vi "Main_GraphBasedSLAM.vi"() -> ()   [LabVIEW 2019]
uses:
  Ctrl/cmd_ini-RW.ctl
  Ctrl/cmd_common.ctl
  <vilib>/Analysis/Matrix/Datatypes/RealMatrix.ctl
  <vilib>/Analysis/Matrix/Numeric/Conversions/Matrix To Array - RM.vi
  <vilib>/Analysis/Matrix/NI_Matrix.lvlib
panel:
  in  "tab":enum32{"ini val", "Graph"}(tab)=enum."Graph"
  in  "rf_id":cluster{"x":dbl, "y":dbl, "yaw":dbl}[](array[cluster])=[{"x"=10.0, "y"=-2.0, "yaw"=0.0}, {"x"=15.0, "y"=10.0, "yaw"=0.0}, {"x"=3.0, "y"=15.0, "yaw"=0.0}, {"x"=-5.0, "y"=20.0, "yaw"=0.0}, {"x"=-5.0, "y"=5.0, "yaw"=0.0}]
  out "x_opt out":cluster{"x":dbl, "y":dbl, "yaw":dbl}[](array[cluster])
  out "cost":cluster{"cost":dbl, "cost sum":dbl}(graph)
  out "inv(H) matrix":dbl[][](graph)
  out "H matrix":dbl[][](graph)
  in  "Show graph time":dbl=5.0
  out "GNSS Lat-Long":T1(graph)=[{[{"Real Matrix Element"=-0.03468968743701403, "Real Matrix Element"=0.0}, {"Real Matrix Element"=0.0053006342525533596, "Real Matrix Element"=0.0026827157844343482}, {"Real Matrix Element"=0.07941001084047958, "Real Matrix Element"=0.004354973789417695}, {"Real Matrix Element"=0.3362327951507724, "Real Matrix Element"=-0.0058186211497051445}, {"Real Matrix Element"=0.583991471643908, "Real Matrix Element"=-0.014127319370192896}, {"Real Matrix Element"=0.6015779562809649, "Real Matrix Element"=-0.01792914288198029}, {"Real Matrix Element"=0.781024837247035, "Real Matrix Element"=-0.03778541178555447}, {"Real Matrix Element"=0.7766402178508468, "Real Matrix Element"=-0.030292841174655537}, {"Real Matrix Element"=0.9431072219093555, "Real Matrix Element"=-0.011465267340174822}, {"Real Matrix Element"=0.9753969820468079, "Real Matrix Element"=-0.015941763963851434}, {"Real Matrix Element"=1.2132401576078795, "Real Matrix Element"=0.041893519310891164}, {"Real Matrix Element"=1.225107293796763, "Real Matrix Element"=0.047604652068552356}, {"Real Matrix Element"=1.2761491555327105, "Real Matrix Element"=0.0704489082853088}, {"Real Matrix Element"=1.4096463396242502, "Real Matrix Element"=0.0514810355329801}, {"Real Matrix Element"=1.6740586724996822, "Real Matrix Element"=0.009317748649650522}, {"Real Matrix Element"=1.8512682178384547, "Real Matrix Element"=-0.00638301099148434}, {"Real Matrix Element"=1.7681597665695883, "Real Matrix Element"=0.01034169292533106}, {"Real Matrix Element"=1.695081912768819, "Real Matrix Element"=0.0771652637847412}, {"Real Matrix Element"=1.8401006709321701, "Real Matrix Element"=0.03677338128353985}, {"Real Matrix Element"=2.1461565709863093, "Real Matrix Element"=0.01382817628790585}, {"Real Matrix Element"=2.1374096596401855, "Real Matrix Element"=0.057469030626545535}, {"Real Matrix Element"=2.1543438113032565, "Real Matrix Element"=0.1009952688750678}, {"Real Matrix Element"=2.146823758678734, "Real Matrix Element"=0.1367303180764168}, {"Real Matrix Element"=2.313726904376567, "Real Matrix Element"=0.15669480341095504}, {"Real Matrix Element"=2.448165076358712, "Real Matrix Element"=0.11806130227193384}, {"Real Matrix Element"=2.7581327970333787, "Real Matrix Element"=0.26114866202850523}, {"Real Matrix Element"=2.7786219786094453, "Real Matrix Element"=0.26959867008849003}, {"Real Matrix Element"=2.7594754945447324, "Real Matrix Element"=0.3049764548145187}, {"Real Matrix Element"=2.84464001198685, "Real Matrix Element"=0.3740548085974285}, {"Real Matrix Element"=3.0672617807939404, "Real Matrix Element"=0.4708806158706211}, {"Real Matrix Element"=3.0361758327160504, "Real Matrix Element"=0.44569336725203174}, {"Real Matrix Element"=3.2385063300702264, "Real Matrix Element"=0.6279704263246847}, {"Real Matrix Element"=3.158876246209658, "Real Matrix Element"=0.5887655997024159}, {"Real Matrix Element"=3.2657902319652283, "Real Matrix Element"=0.5698844075564534}, {"Real Matrix Element"=3.4763236561457407, "Real Matrix Element"=0.6411314057308733}, {"Real Matrix Element"=3.7070629090554124, "Real Matrix Element"=0.7376824418190701}, {"Real Matrix Element"=3.471507531519639, "Real Matrix Element"=0.6082208970914108}, {"Real Matrix Element"=3.468422407890875, "Real Matrix Element"=0.5832337660513986}, {"Real Matrix Element"=3.6926573968702523, "Real Matrix Element"=0.650637040965163}, {"Real Matrix Element"=3.786513246652574, "Real Matrix Element"=0.6968034902141617}, {"Real Matrix Element"=3.8331446853344846, "Real Matrix Element"=0.7214149291160856}, {"Real Matrix Element"=4.139757466627785, "Real Matrix Element"=0.809998000333033}, {"Real Matrix Element"=4.248379077592784, "Real Matrix Element"=0.8887749010940235}, {"Real Matrix Element"=4.291416416102754, "Real Matrix Element"=0.9302004333873511}, {"Real Matrix Element"=4.388536273927073, "Real Matrix Element"=0.9726232319618774}, {"Real Matrix Element"=4.441533604730054, "Real Matrix Element"=0.982456213949647}, {"Real Matrix Element"=4.378412481659074, "Real Matrix Element"=0.9890784356681216}, {"Real Matrix Element"=4.340768240114929, "Real Matrix Element"=0.9501541887317771}, {"Real Matrix Element"=4.730916620020055, "Real Matrix Element"=1.0838146366018384}, {"Real Matrix Element"=4.912452197538009, "Real Matrix Element"=1.162342901661344}, {"Real Matrix Element"=4.825944638027306, "Real Matrix Element"=1.1586414211370888}, {"Real Matrix Element"=4.9213835121734855, "Real Matrix Element"=1.2233317580436667}, {"Real Matrix Element"=5.101684298563478, "Real Matrix Element"=1.28468992427372}, {"Real Matrix Element"=5.158081340723653, "Real Matrix Element"=1.3099289126706322}, {"Real Matrix Element"=5.159416761230016, "Real Matrix Element"=1.398556706013839}, {"Real Matrix Element"=5.3471415623690275, "Real Matrix Element"=1.5654936582727805}, {"Real Matrix Element"=5.328698595785637, "Real Matrix Element"=1.5248269436628135}, {"Real Matrix Element"=5.379360527810359, "Real Matrix Element"=1.5866110047489936}, {"Real Matrix Element"=5.35038316326285, "Real Matrix Element"=1.5377931623663355}, {"Real Matrix Element"=5.443660439629705, "Real Matrix Element"=1.5760009953026846}, {"Real Matrix Element"=5.55009144649403, "Real Matrix Element"=1.5827157152432425}, {"Real Matrix Element"=5.630932772361487, "Real Matrix Element"=1.651698572576983}, {"Real Matrix Element"=5.80878936655062, "Real Matrix Element"=1.7980429647417366}, {"Real Matrix Element"=5.866750613452901, "Real Matrix Element"=1.8406843191521158}, {"Real Matrix Element"=6.148904460793132, "Real Matrix Element"=2.0349587948261143}, {"Real Matrix Element"=6.199722277513993, "Real Matrix Element"=2.162546289313033}, {"Real Matrix Element"=6.273186799733598, "Real Matrix Element"=2.2143895799792257}, {"Real Matrix Element"=6.257435774415471, "Real Matrix Element"=2.16572006395123}, {"Real Matrix Element"=6.305396243815897, "Real Matrix Element"=2.137282024059232}, {"Real Matrix Element"=6.505305716477432, "Real Matrix Element"=2.2743982916383523}, {"Real Matrix Element"=6.724475476833821, "Real Matrix Element"=2.439450988877147}, {"Real Matrix Element"=6.946569400735926, "Real Matrix Element"=2.604318681364871}, {"Real Matrix Element"=6.653000783211806, "Real Matrix Element"=2.4169256335119607}, {"Real Matrix Element"=6.73427443971705, "Real Matrix Element"=2.491353741536716}, {"Real Matrix Element"=6.9052374013046345, "Real Matrix Element"=2.626868519132758}, {"Real Matrix Element"=6.893956205594916, "Real Matrix Element"=2.624484623904043}, {"Real Matrix Element"=7.04426827535472, "Real Matrix Element"=2.747191138164331}, {"Real Matrix Element"=6.990174871380481, "Real Matrix Element"=2.695254099345242}, {"Real Matrix Element"=7.007024544463572, "Real Matrix Element"=2.7211094022272366}, {"Real Matrix Element"=7.1766175063450195, "Real Matrix Element"=2.870310687044355}, {"Real Matrix Element"=7.449190792560847, "Real Matrix Element"=3.1179512689421256}, {"Real Matrix Element"=7.469388700071343, "Real Matrix Element"=3.1398319180341128}, {"Real Matrix Element"=7.624314922187709, "Real Matrix Element"=3.2932663538566587}, {"Real Matrix Element"=7.781989543008123, "Real Matrix Element"=3.437678606345636}, {"Real Matrix Element"=7.77953650519987, "Real Matrix Element"=3.479662617914875}, {"Real Matrix Element"=7.751830731131396, "Real Matrix Element"=3.564090678543888}, {"Real Matrix Element"=7.679780382368366, "Real Matrix Element"=3.5042469842473074}, {"Real Matrix Element"=7.68903372893383, "Real Matrix Element"=3.5235343769124006}, {"Real Matrix Element"=7.7500557341243885, "Real Matrix Element"=3.5803002767540892}, {"Real Matrix Element"=7.879450248061815, "Real Matrix Element"=3.6595173257087565}, {"Real Matrix Element"=8.043957091054015, "Real Matrix Element"=3.8685315777721416}, {"Real Matrix Element"=8.05864625885395, "Real Matrix Element"=3.919715437341979}, {"Real Matrix Element"=8.028384162747386, "Real Matrix Element"=3.8964158670860845}, {"Real Matrix Element"=8.127439035035303, "Real Matrix Element"=3.955172234989489}, {"Real Matrix Element"=8.197030981277198, "Real Matrix Element"=4.051067169641669}, {"Real Matrix Element"=8.290825422349103, "Real Matrix Element"=4.254545440502117}, {"Real Matrix Element"=8.365502774498013, "Real Matrix Element"=4.352985571112935}, {"Real Matrix Element"=8.443200210371124, "Real Matrix Element"=4.451055738157268}, {"Real Matrix Element"=8.431750227334298, "Real Matrix Element"=4.5050817067549245}, {"Real Matrix Element"=8.550286889019615, "Real Matrix Element"=4.587270025887594}, {"Real Matrix Element"=8.655984807507547, "Real Matrix Element"=4.702848486958322}, {"Real Matrix Element"=8.7348113753029, "Real Matrix Element"=4.822863446270891}, {"Real Matrix Element"=8.890929752995335, "Real Matrix Element"=4.884559500188374}, {"Real Matrix Element"=8.904444786282742, "Real Matrix Element"=4.8913058137575085}, {"Real Matrix Element"=8.95248901538359, "Real Matrix Element"=5.043214702865114}, {"Real Matrix Element"=8.862493310795744, "Real Matrix Element"=4.941626877820068}, {"Real Matrix Element"=9.09178551016537, "Real Matrix Element"=5.215355670008168}, {"Real Matrix Element"=9.227547238024945, "Real Matrix Element"=5.418909983280011}, {"Real Matrix Element"=9.019949270660604, "Real Matrix Element"=5.381190670011399}, {"Real Matrix Element"=8.902531951325166, "Real Matrix Element"=5.293441005377548}, {"Real Matrix Element"=8.943158857688749, "Real Matrix Element"=5.417283923897843}, {"Real Matrix Element"=8.954552232844819, "Real Matrix Element"=5.542174997187985}, {"Real Matrix Element"=8.974372300088339, "Real Matrix Element"=5.642063167864399}, {"Real Matrix Element"=8.962737155688917, "Real Matrix Element"=5.654404711386451}, {"Real Matrix Element"=9.025737618510878, "Real Matrix Element"=5.833298394107455}, {"Real Matrix Element"=9.075254784427909, "Real Matrix Element"=6.021350980226874}, {"Real Matrix Element"=9.065960884888513, "Real Matrix Element"=6.027867120575307}, {"Real Matrix Element"=9.224204901053707, "Real Matrix Element"=6.105947456671318}, {"Real Matrix Element"=9.187613712193818, "Real Matrix Element"=6.051245464291332}, {"Real Matrix Element"=9.246097071838237, "Real Matrix Element"=6.157461731815137}, {"Real Matrix Element"=9.349248799464768, "Real Matrix Element"=6.313060466328618}, {"Real Matrix Element"=9.532656646093448, "Real Matrix Element"=6.465934574847335}, {"Real Matrix Element"=9.621107831340138, "Real Matrix Element"=6.601895387534528}, {"Real Matrix Element"=9.633238827003911, "Real Matrix Element"=6.586457724060519}, {"Real Matrix Element"=9.629635920761233, "Real Matrix Element"=6.668819486890973}, {"Real Matrix Element"=9.848505498190669, "Real Matrix Element"=6.980639728314059}, {"Real Matrix Element"=9.776130216267585, "Real Matrix Element"=7.0039438168116215}, {"Real Matrix Element"=9.724835179001373, "Real Matrix Element"=6.999432070804583}, {"Real Matrix Element"=9.769350212050192, "Real Matrix Element"=7.11657047190726}, {"Real Matrix Element"=9.84737105007721, "Real Matrix Element"=7.2787851626182904}, {"Real Matrix Element"=9.904498370680217, "Real Matrix Element"=7.7022006939560725}, {"Real Matrix Element"=9.852720819729717, "Real Matrix Element"=7.526539204709166}, {"Real Matrix Element"=9.871788029686165, "Real Matrix Element"=7.5037016748604}, {"Real Matrix Element"=9.900351156834887, "Real Matrix Element"=7.648470740173559}, {"Real Matrix Element"=9.88986257123532, "Real Matrix Element"=7.678880896080778}, {"Real Matrix Element"=10.07847433662867, "Real Matrix Element"=8.082474114095065}, {"Real Matrix Element"=10.022684238972921, "Real Matrix Element"=7.958307280059712}, {"Real Matrix Element"=10.02463365645684, "Real Matrix Element"=8.012849780357792}, {"Real Matrix Element"=10.029412871278998, "Real Matrix Element"=8.165425351868802}, {"Real Matrix Element"=10.054328298882655, "Real Matrix Element"=8.374441730258086}, {"Real Matrix Element"=9.961596787706776, "Real Matrix Element"=8.285582107994475}, {"Real Matrix Element"=10.00575919840209, "Real Matrix Element"=8.59102227348544}, {"Real Matrix Element"=10.116701880207133, "Real Matrix Element"=8.662211347605572}, {"Real Matrix Element"=10.067266555941785, "Real Matrix Element"=8.474118654060423}, {"Real Matrix Element"=10.128057929134007, "Real Matrix Element"=8.660141128696779}, {"Real Matrix Element"=10.079071156248302, "Real Matrix Element"=8.768850612025686}, {"Real Matrix Element"=10.10027890687739, "Real Matrix Element"=8.991463361488702}, {"Real Matrix Element"=10.060651726414047, "Real Matrix Element"=9.11908297578028}, {"Real Matrix Element"=9.916440339048242, "Real Matrix Element"=9.285053689363842}, {"Real Matrix Element"=9.91586017664551, "Real Matrix Element"=9.463518857014039}, {"Real Matrix Element"=9.81173882931321, "Real Matrix Element"=9.442756978179288}, {"Real Matrix Element"=9.96137271074314, "Real Matrix Element"=9.286782455007117}, {"Real Matrix Element"=9.824565598325435, "Real Matrix Element"=9.619284721164862}, {"Real Matrix Element"=9.92793838557228, "Real Matrix Element"=9.524140760440789}, {"Real Matrix Element"=9.880931444609335, "Real Matrix Element"=9.788960416667566}, {"Real Matrix Element"=9.915039245751517, "Real Matrix Element"=9.810297209615387}, {"Real Matrix Element"=9.924016272338754, "Real Matrix Element"=9.79733578278899}, {"Real Matrix Element"=9.918698787142002, "Real Matrix Element"=9.828787008204957}, {"Real Matrix Element"=9.920719096710409, "Real Matrix Element"=9.981572114989616}, {"Real Matrix Element"=9.945958087549677, "Real Matrix Element"=10.045720805438242}, {"Real Matrix Element"=9.860041385600256, "Real Matrix Element"=10.238399836578763}, {"Real Matrix Element"=9.9507002921587, "Real Matrix Element"=10.295744294865079}, {"Real Matrix Element"=10.01278224421081, "Real Matrix Element"=10.476659456234666}, {"Real Matrix Element"=9.991508550805726, "Real Matrix Element"=10.683837189279918}, {"Real Matrix Element"=9.945592240943817, "Real Matrix Element"=10.958614838986609}, {"Real Matrix Element"=9.945377330760733, "Real Matrix Element"=11.0469128019319}, {"Real Matrix Element"=9.941295397295482, "Real Matrix Element"=11.005648846749006}, {"Real Matrix Element"=9.875761349770913, "Real Matrix Element"=11.280257076914275}, {"Real Matrix Element"=9.87579740713653, "Real Matrix Element"=11.374864690067911}, {"Real Matrix Element"=9.855083135796619, "Real Matrix Element"=11.473145479478884}, {"Real Matrix Element"=9.829514681159326, "Real Matrix Element"=11.510988849300338}, {"Real Matrix Element"=9.894649739442537, "Real Matrix Element"=11.436291080516865}, {"Real Matrix Element"=9.88686381414674, "Real Matrix Element"=11.553454826976933}, {"Real Matrix Element"=9.794425116792429, "Real Matrix Element"=11.677862098534543}, {"Real Matrix Element"=9.804426340818509, "Real Matrix Element"=11.632584157808767}, {"Real Matrix Element"=9.77039061025429, "Real Matrix Element"=11.723572483384102}, {"Real Matrix Element"=9.834314051242325, "Real Matrix Element"=12.11952531981535}, {"Real Matrix Element"=9.867716180129866, "Real Matrix Element"=12.172936851702284}, {"Real Matrix Element"=9.901883644300801, "Real Matrix Element"=12.160348147158548}, {"Real Matrix Element"=9.890220710596573, "Real Matrix Element"=12.001850458445725}, {"Real Matrix Element"=9.837432718319059, "Real Matrix Element"=12.377725051617269}, {"Real Matrix Element"=9.867957576127036, "Real Matrix Element"=12.225752433857426}, {"Real Matrix Element"=9.845226898568914, "Real Matrix Element"=12.52471434746288}, {"Real Matrix Element"=9.816843082217062, "Real Matrix Element"=12.73812142324634}, {"Real Matrix Element"=9.662390401222558, "Real Matrix Element"=12.853985192052154}, {"Real Matrix Element"=9.571821797416716, "Real Matrix Element"=12.852708844948223}, {"Real Matrix Element"=9.551552455445933, "Real Matrix Element"=12.936960509671016}, {"Real Matrix Element"=9.54527834591418, "Real Matrix Element"=13.009467072593939}, {"Real Matrix Element"=9.517297725748248, "Real Matrix Element"=13.13902990376155}, {"Real Matrix Element"=9.434993632431034, "Real Matrix Element"=13.325924259956803}, {"Real Matrix Element"=9.501864840546176, "Real Matrix Element"=13.258855685075169}, {"Real Matrix Element"=9.426267292147163, "Real Matrix Element"=13.34674762888347}, {"Real Matrix Element"=9.532841939869472, "Real Matrix Element"=13.505649986724883}, {"Real Matrix Element"=9.42207728143737, "Real Matrix Element"=13.49945444707442}, {"Real Matrix Element"=9.394580285201748, "Real Matrix Element"=13.758550318867218}, {"Real Matrix Element"=9.234980449171267, "Real Matrix Element"=13.665985485091577}, {"Real Matrix Element"=9.161996981698925, "Real Matrix Element"=13.817063958882272}, {"Real Matrix Element"=9.20591574506749, "Real Matrix Element"=13.798712837375055}, {"Real Matrix Element"=9.133725667437963, "Real Matrix Element"=13.88782288668861}, {"Real Matrix Element"=9.09201417149409, "Real Matrix Element"=14.07472354474414}, {"Real Matrix Element"=9.146446373431704, "Real Matrix Element"=13.964969514003947}, {"Real Matrix Element"=9.003214752914296, "Real Matrix Element"=14.289688224115656}, {"Real Matrix Element"=9.03187905272531, "Real Matrix Element"=14.352718328431514}, {"Real Matrix Element"=8.987197663892374, "Real Matrix Element"=14.503874917434764}, {"Real Matrix Element"=8.896568382331566, "Real Matrix Element"=14.711155955179148}, {"Real Matrix Element"=8.863582369910583, "Real Matrix Element"=14.6807068039072}, {"Real Matrix Element"=8.92755362952385, "Real Matrix Element"=14.807019909032793}, {"Real Matrix Element"=8.929160525699093, "Real Matrix Element"=14.704743536172431}, {"Real Matrix Element"=8.793900022113176, "Real Matrix Element"=14.949367130028444}, {"Real Matrix Element"=8.78017150877093, "Real Matrix Element"=15.141187262957187}, {"Real Matrix Element"=8.7399034089085, "Real Matrix Element"=15.16159237871607}, {"Real Matrix Element"=8.695367104843049, "Real Matrix Element"=15.156410157813466}, {"Real Matrix Element"=8.622573306792289, "Real Matrix Element"=15.211836228911128}, {"Real Matrix Element"=8.590260308077044, "Real Matrix Element"=15.259754921652934}, {"Real Matrix Element"=8.585189846021304, "Real Matrix Element"=15.3261291919036}, {"Real Matrix Element"=8.494497336103569, "Real Matrix Element"=15.522870439592577}, {"Real Matrix Element"=8.393519437393039, "Real Matrix Element"=15.632209768168496}, {"Real Matrix Element"=8.361143425952093, "Real Matrix Element"=15.646702119363924}, {"Real Matrix Element"=8.290414268944321, "Real Matrix Element"=15.797940613467164}, {"Real Matrix Element"=8.304590461322375, "Real Matrix Element"=15.75698759980346}, {"Real Matrix Element"=8.13659747350902, "Real Matrix Element"=15.971144102734959}, {"Real Matrix Element"=8.09466233970046, "Real Matrix Element"=15.972848079670731}, {"Real Matrix Element"=8.05644908252468, "Real Matrix Element"=16.08570451873167}, {"Real Matrix Element"=7.935908043214175, "Real Matrix Element"=16.185270719148416}, {"Real Matrix Element"=7.930561082846518, "Real Matrix Element"=16.306740941355194}, {"Real Matrix Element"=7.84899646736477, "Real Matrix Element"=16.38735469492071}, {"Real Matrix Element"=7.700072424649776, "Real Matrix Element"=16.455917496120126}, {"Real Matrix Element"=7.6471251254366, "Real Matrix Element"=16.551010044009914}, {"Real Matrix Element"=7.454767277572828, "Real Matrix Element"=16.783973139564825}, {"Real Matrix Element"=7.5801749729545795, "Real Matrix Element"=16.666587689528857}, {"Real Matrix Element"=7.438916557973434, "Real Matrix Element"=16.84169933095558}, {"Real Matrix Element"=7.395363755908117, "Real Matrix Element"=16.838151132574154}, {"Real Matrix Element"=7.4484757425925485, "Real Matrix Element"=16.82163101720974}, {"Real Matrix Element"=7.369431097348007, "Real Matrix Element"=16.88966005377285}, {"Real Matrix Element"=7.210792803295144, "Real Matrix Element"=17.016807905066592}, {"Real Matrix Element"=7.106956799863978, "Real Matrix Element"=17.131262550453613}, {"Real Matrix Element"=7.001706371541313, "Real Matrix Element"=17.211281387632894}, {"Real Matrix Element"=6.920493430282399, "Real Matrix Element"=17.26139699652119}, {"Real Matrix Element"=6.810628273383016, "Real Matrix Element"=17.305106911503472}, {"Real Matrix Element"=6.84712382939114, "Real Matrix Element"=17.269094879356864}, {"Real Matrix Element"=6.755046661796092, "Real Matrix Element"=17.334649555369104}, {"Real Matrix Element"=6.566821376801988, "Real Matrix Element"=17.47474399500857}, {"Real Matrix Element"=6.60002989528175, "Real Matrix Element"=17.443611940496975}, {"Real Matrix Element"=6.5551302313636235, "Real Matrix Element"=17.469096460361676}, {"Real Matrix Element"=6.429289906630709, "Real Matrix Element"=17.515201018696605}, {"Real Matrix Element"=6.240429162253012, "Real Matrix Element"=17.63474300564612}, {"Real Matrix Element"=6.163426397206234, "Real Matrix Element"=17.666570824258184}, {"Real Matrix Element"=6.117660748561346, "Real Matrix Element"=17.707596110492428}, {"Real Matrix Element"=6.104767709273946, "Real Matrix Element"=17.747512932765417}, {"Real Matrix Element"=5.950168620943996, "Real Matrix Element"=17.88641202980151}, {"Real Matrix Element"=5.904601353299042, "Real Matrix Element"=17.940683062231695}, {"Real Matrix Element"=5.845969221242629, "Real Matrix Element"=17.989450748140335}, {"Real Matrix Element"=5.703357185170327, "Real Matrix Element"=18.09683074564596}, {"Real Matrix Element"=5.678480689976378, "Real Matrix Element"=18.099871485054056}, {"Real Matrix Element"=5.740684153548074, "Real Matrix Element"=18.08967913636726}, {"Real Matrix Element"=5.585136340987132, "Real Matrix Element"=18.169440706276227}, {"Real Matrix Element"=5.3073483746023005, "Real Matrix Element"=18.54045821787915}, {"Real Matrix Element"=5.375714581930705, "Real Matrix Element"=18.396726460097458}, {"Real Matrix Element"=5.299163987326189, "Real Matrix Element"=18.46403607778465}, {"Real Matrix Element"=5.197099253400948, "Real Matrix Element"=18.42474704623824}, {"Real Matrix Element"=5.112611553578863, "Real Matrix Element"=18.503154499182703}, {"Real Matrix Element"=5.107015922545976, "Real Matrix Element"=18.507797384563784}, {"Real Matrix Element"=4.849586707929752, "Real Matrix Element"=18.6799037480304}, {"Real Matrix Element"=4.722423547350224, "Real Matrix Element"=18.780231817315997}, {"Real Matrix Element"=4.869826401939896, "Real Matrix Element"=18.708003302908597}, {"Real Matrix Element"=4.74859656744415, "Real Matrix Element"=18.869336901249984}, {"Real Matrix Element"=4.5694141893642675, "Real Matrix Element"=18.889400570921037}, {"Real Matrix Element"=4.539116202957918, "Real Matrix Element"=18.89774860310237}, {"Real Matrix Element"=4.392750957458958, "Real Matrix Element"=19.002789093207806}, {"Real Matrix Element"=4.259250678983671, "Real Matrix Element"=19.106175271197937}, {"Real Matrix Element"=4.214743643664578, "Real Matrix Element"=19.125419485795376}, {"Real Matrix Element"=4.053996318029018, "Real Matrix Element"=19.15470643355179}, {"Real Matrix Element"=4.140094621473842, "Real Matrix Element"=19.130161466921308}, {"Real Matrix Element"=3.980832730840746, "Real Matrix Element"=19.182537301901146}, {"Real Matrix Element"=4.150663980302334, "Real Matrix Element"=19.124313608890354}, {"Real Matrix Element"=3.771477111182339, "Real Matrix Element"=19.253717732931225}, {"Real Matrix Element"=3.883391674301052, "Real Matrix Element"=19.21556098701026}, {"Real Matrix Element"=3.633298371658127, "Real Matrix Element"=19.36355241512018}, {"Real Matrix Element"=3.382858863495134, "Real Matrix Element"=19.49921752990067}, {"Real Matrix Element"=3.299124750722708, "Real Matrix Element"=19.516605026087763}, {"Real Matrix Element"=3.325406725344531, "Real Matrix Element"=19.4547048398925}, {"Real Matrix Element"=3.30930200264818, "Real Matrix Element"=19.445182272776503}, {"Real Matrix Element"=3.170858419727473, "Real Matrix Element"=19.450369189313836}, {"Real Matrix Element"=2.845488706168646, "Real Matrix Element"=19.48817024077186}, {"Real Matrix Element"=3.041244663695119, "Real Matrix Element"=19.47052087030442}, {"Real Matrix Element"=2.7533033875306785, "Real Matrix Element"=19.463339757850196}, {"Real Matrix Element"=2.6246487056615937, "Real Matrix Element"=19.460627830947473}, {"Real Matrix Element"=2.9047802348563616, "Real Matrix Element"=19.49715553720029}, {"Real Matrix Element"=2.7062109840561086, "Real Matrix Element"=19.52593914748948}, {"Real Matrix Element"=2.361347671892243, "Real Matrix Element"=19.572854909054836}, {"Real Matrix Element"=2.2725283450898237, "Real Matrix Element"=19.55826516258584}, {"Real Matrix Element"=2.19872425393435, "Real Matrix Element"=19.59030951897816}, {"Real Matrix Element"=2.1622345703484163, "Real Matrix Element"=19.612913135702247}, {"Real Matrix Element"=2.128802658214441, "Real Matrix Element"=19.622403545017747}, {"Real Matrix Element"=1.9205973027856327, "Real Matrix Element"=19.642540187711802}, {"Real Matrix Element"=1.8052733841439972, "Real Matrix Element"=19.74165067445746}, {"Real Matrix Element"=1.6495538333392152, "Real Matrix Element"=19.7949447338851}, {"Real Matrix Element"=1.7192914610727683, "Real Matrix Element"=19.761747770990944}, {"Real Matrix Element"=1.556265366384677, "Real Matrix Element"=19.800857592102552}, {"Real Matrix Element"=1.417189572852484, "Real Matrix Element"=19.86483478616262}, {"Real Matrix Element"=1.3514533837893123, "Real Matrix Element"=19.862084716110417}, {"Real Matrix Element"=1.303871192734623, "Real Matrix Element"=19.871784081912875}, {"Real Matrix Element"=1.0676898847775556, "Real Matrix Element"=19.878112855124755}, {"Real Matrix Element"=0.8553293895647015, "Real Matrix Element"=19.924170695347865}, {"Real Matrix Element"=0.9604404595298575, "Real Matrix Element"=19.976005244858452}, {"Real Matrix Element"=0.9649235343696104, "Real Matrix Element"=19.98753680102894}, {"Real Matrix Element"=0.8401836142037414, "Real Matrix Element"=19.98351883772752}, {"Real Matrix Element"=0.7777104207534306, "Real Matrix Element"=19.985452835528907}, {"Real Matrix Element"=0.5985248413407827, "Real Matrix Element"=19.988987840963414}, {"Real Matrix Element"=0.6832745873564265, "Real Matrix Element"=20.001097694331946}, {"Real Matrix Element"=0.4579433023653162, "Real Matrix Element"=20.013471752238175}, {"Real Matrix Element"=0.025252478555629333, "Real Matrix Element"=20.095975685216963}, {"Real Matrix Element"=0.10693563275810292, "Real Matrix Element"=20.04489196388176}, {"Real Matrix Element"=-0.023780220086366658, "Real Matrix Element"=20.098438489972807}, {"Real Matrix Element"=0.08565945343971836, "Real Matrix Element"=20.06208688314802}, {"Real Matrix Element"=-0.06961325067465408, "Real Matrix Element"=20.136202695962055}, {"Real Matrix Element"=-0.11782645235843013, "Real Matrix Element"=20.131313182314383}, {"Real Matrix Element"=-0.08864992694348649, "Real Matrix Element"=20.0838270762904}, {"Real Matrix Element"=-0.22527915335645132, "Real Matrix Element"=20.127339372978586}, {"Real Matrix Element"=-0.3008712929292075, "Real Matrix Element"=20.131856580310075}, {"Real Matrix Element"=-0.34993206608568295, "Real Matrix Element"=20.090931373866063}, {"Real Matrix Element"=-0.5606787922516503, "Real Matrix Element"=20.065695516748203}, {"Real Matrix Element"=-0.7344999957322501, "Real Matrix Element"=20.077125959313413}, {"Real Matrix Element"=-1.003215412542282, "Real Matrix Element"=20.15461564571834}, {"Real Matrix Element"=-0.8083322075081077, "Real Matrix Element"=20.110072726393966}, {"Real Matrix Element"=-1.0671356357128223, "Real Matrix Element"=20.05904561404013}, {"Real Matrix Element"=-1.1161243930073745, "Real Matrix Element"=20.125503707343547}, {"Real Matrix Element"=-1.0928943575333043, "Real Matrix Element"=20.10460355047025}, {"Real Matrix Element"=-1.5554084477534762, "Real Matrix Element"=19.89003881334554}, {"Real Matrix Element"=-1.4732909705297064, "Real Matrix Element"=19.945033728043533}, {"Real Matrix Element"=-1.616024054603416, "Real Matrix Element"=19.91638549584566}, {"Real Matrix Element"=-1.7280533180145414, "Real Matrix Element"=19.93688811338996}, {"Real Matrix Element"=-1.725748298380875, "Real Matrix Element"=19.959482347190107}, {"Real Matrix Element"=-1.9504954301010005, "Real Matrix Element"=19.878786399546257}, {"Real Matrix Element"=-2.0858677203107128, "Real Matrix Element"=19.79520978554725}, {"Real Matrix Element"=-2.2091876801094967, "Real Matrix Element"=19.79573865461739}, {"Real Matrix Element"=-2.2713678806879813, "Real Matrix Element"=19.71575089895021}, {"Real Matrix Element"=-2.24376238704464, "Real Matrix Element"=19.735929252462512}, {"Real Matrix Element"=-2.307608832675007, "Real Matrix Element"=19.68923282966359}, {"Real Matrix Element"=-2.5267571172198457, "Real Matrix Element"=19.585328161548528}, {"Real Matrix Element"=-2.5902824988184316, "Real Matrix Element"=19.528192985336272}, {"Real Matrix Element"=-2.67290080254935, "Real Matrix Element"=19.507395436734758}, {"Real Matrix Element"=-3.003101850803522, "Real Matrix Element"=19.369644360111597}, {"Real Matrix Element"=-2.840899292110878, "Real Matrix Element"=19.473696896354642}, {"Real Matrix Element"=-3.203599795409282, "Real Matrix Element"=19.233920942218855}, {"Real Matrix Element"=-3.1882922096648953, "Real Matrix Element"=19.216371676412567}, {"Real Matrix Element"=-3.101426504698728, "Real Matrix Element"=19.380018935207303}, {"Real Matrix Element"=-3.2711676533941567, "Real Matrix Element"=19.28399706452759}, {"Real Matrix Element"=-3.117392703935339, "Real Matrix Element"=19.335628442459814}, {"Real Matrix Element"=-3.2426814371583745, "Real Matrix Element"=19.24510341802347}, {"Real Matrix Element"=-3.4071355244128156, "Real Matrix Element"=19.093821789981522}, {"Real Matrix Element"=-3.9048827836161837, "Real Matrix Element"=18.880166385784243}, {"Real Matrix Element"=-4.077255257963245, "Real Matrix Element"=18.81383739339177}, {"Real Matrix Element"=-4.029606594227185, "Real Matrix Element"=18.838304395565302}, {"Real Matrix Element"=-4.2984807288347895, "Real Matrix Element"=18.784742761715002}, {"Real Matrix Element"=-4.436864314013776, "Real Matrix Element"=18.7622278090133}, {"Real Matrix Element"=-4.319217979210337, "Real Matrix Element"=18.819478727854012}, {"Real Matrix Element"=-4.427657051545266, "Real Matrix Element"=18.821164352722153}, {"Real Matrix Element"=-4.356975054402508, "Real Matrix Element"=18.85221308620525}, {"Real Matrix Element"=-4.370875708069801, "Real Matrix Element"=18.86670987692545}, {"Real Matrix Element"=-4.310049522897323, "Real Matrix Element"=18.884446687718025}, {"Real Matrix Element"=-4.487771427316906, "Real Matrix Element"=18.845350255771045}, {"Real Matrix Element"=-4.6397633010224615, "Real Matrix Element"=18.82340494809872}, {"Real Matrix Element"=-4.651801350127629, "Real Matrix Element"=18.812742138977836}, {"Real Matrix Element"=-4.6893642256318975, "Real Matrix Element"=18.81466813682964}, {"Real Matrix Element"=-4.665439374714008, "Real Matrix Element"=18.814998157937772}, {"Real Matrix Element"=-4.872454287142064, "Real Matrix Element"=18.803788578530508}, {"Real Matrix Element"=-4.881354605377065, "Real Matrix Element"=18.75695911286054}, {"Real Matrix Element"=-4.8558911993319915, "Real Matrix Element"=18.79590156264286}, {"Real Matrix Element"=-5.152468466352134, "Real Matrix Element"=18.679556363896324}, {"Real Matrix Element"=-5.1933725207390555, "Real Matrix Element"=18.64544269803664}, {"Real Matrix Element"=-5.180252523018569, "Real Matrix Element"=18.668274416385408}, {"Real Matrix Element"=-5.388781087135984, "Real Matrix Element"=18.591838248712097}, {"Real Matrix Element"=-5.509059219227287, "Real Matrix Element"=18.53114306080663}, {"Real Matrix Element"=-5.5747637778320716, "Real Matrix Element"=18.474170114674536}, {"Real Matrix Element"=-5.4892095700566, "Real Matrix Element"=18.51676948923419}, {"Real Matrix Element"=-5.907690917127198, "Real Matrix Element"=18.30202644450812}, {"Real Matrix Element"=-5.8657596522743125, "Real Matrix Element"=18.302191986474273}, {"Real Matrix Element"=-5.99680425478754, "Real Matrix Element"=18.21094264801285}, {"Real Matrix Element"=-6.086979939707041, "Real Matrix Element"=18.070339950914555}, {"Real Matrix Element"=-6.2046975725010105, "Real Matrix Element"=17.935906399008484}, {"Real Matrix Element"=-6.3102497725908435, "Real Matrix Element"=17.804907067541333}, {"Real Matrix Element"=-6.212079019489753, "Real Matrix Element"=17.900630411864885}, {"Real Matrix Element"=-6.381388661509583, "Real Matrix Element"=17.727286242364976}, {"Real Matrix Element"=-6.506495579939761, "Real Matrix Element"=17.615817816001783}, {"Real Matrix Element"=-6.6366758844601295, "Real Matrix Element"=17.41944136660784}, {"Real Matrix Element"=-6.592704953759556, "Real Matrix Element"=17.45314106792762}, {"Real Matrix Element"=-6.671727990276716, "Real Matrix Element"=17.388438561751403}, {"Real Matrix Element"=-6.7273633427276724, "Real Matrix Element"=17.287879851753246}, {"Real Matrix Element"=-6.71565746420877, "Real Matrix Element"=17.26371709134385}, {"Real Matrix Element"=-6.734650398864989, "Real Matrix Element"=17.288869842934478}, {"Real Matrix Element"=-6.841021712844639, "Real Matrix Element"=17.159365675690673}, {"Real Matrix Element"=-6.8676576989971805, "Real Matrix Element"=17.14280139733503}, {"Real Matrix Element"=-7.166339827243839, "Real Matrix Element"=17.009240206456166}, {"Real Matrix Element"=-7.178174746968349, "Real Matrix Element"=16.982879082657504}, {"Real Matrix Element"=-7.307231236015355, "Real Matrix Element"=16.84267365474082}, {"Real Matrix Element"=-7.264181866720001, "Real Matrix Element"=16.961498100257952}, {"Real Matrix Element"=-7.2835182188912535, "Real Matrix Element"=16.919565190312372}, {"Real Matrix Element"=-7.358445979441395, "Real Matrix Element"=16.80680545713764}, {"Real Matrix Element"=-7.51419390004495, "Real Matrix Element"=16.576903807234874}, {"Real Matrix Element"=-7.75647770871642, "Real Matrix Element"=16.33858485457655}, {"Real Matrix Element"=-7.705797618399651, "Real Matrix Element"=16.45902962975307}, {"Real Matrix Element"=-7.672887004988971, "Real Matrix Element"=16.43970442849819}, {"Real Matrix Element"=-7.747705835104613, "Real Matrix Element"=16.2381645673467}, {"Real Matrix Element"=-7.757059637689601, "Real Matrix Element"=16.111368412182422}, {"Real Matrix Element"=-7.777702178243173, "Real Matrix Element"=16.08941764369036}, {"Real Matrix Element"=-7.839455487366121, "Real Matrix Element"=16.073164274545586}, {"Real Matrix Element"=-7.926026471661833, "Real Matrix Element"=15.969141684528921}, {"Real Matrix Element"=-7.952966009543173, "Real Matrix Element"=15.980146211190188}, {"Real Matrix Element"=-8.113776134634865, "Real Matrix Element"=15.80044311301177}, {"Real Matrix Element"=-8.130048057406029, "Real Matrix Element"=15.729626698016906}, {"Real Matrix Element"=-8.236713293984314, "Real Matrix Element"=15.296853315108786}, {"Real Matrix Element"=-8.342754997977586, "Real Matrix Element"=15.18296811845647}, {"Real Matrix Element"=-8.370762066115942, "Real Matrix Element"=15.358968318913758}, {"Real Matrix Element"=-8.381429927525462, "Real Matrix Element"=15.253530619738031}, {"Real Matrix Element"=-8.363944412668513, "Real Matrix Element"=15.294907087562413}, {"Real Matrix Element"=-8.40834196865725, "Real Matrix Element"=15.26395939863297}, {"Real Matrix Element"=-8.467803869576606, "Real Matrix Element"=15.114674106508865}, {"Real Matrix Element"=-8.461425727231195, "Real Matrix Element"=14.979357437671437}, {"Real Matrix Element"=-8.470231135387081, "Real Matrix Element"=14.808527623729177}, {"Real Matrix Element"=-8.576965505977258, "Real Matrix Element"=14.595640664874901}, {"Real Matrix Element"=-8.602417438363338, "Real Matrix Element"=14.612468877225915}, {"Real Matrix Element"=-8.677315674258576, "Real Matrix Element"=14.615174533374743}, {"Real Matrix Element"=-8.796794924731106, "Real Matrix Element"=14.349268243241097}, {"Real Matrix Element"=-8.699569343333666, "Real Matrix Element"=14.426798766746401}, {"Real Matrix Element"=-8.786891089482891, "Real Matrix Element"=14.374625456995261}, {"Real Matrix Element"=-8.79161926708816, "Real Matrix Element"=14.242347471759878}, {"Real Matrix Element"=-8.83516829481909, "Real Matrix Element"=14.137868659310213}, {"Real Matrix Element"=-8.917358778499143, "Real Matrix Element"=14.074728687709603}, {"Real Matrix Element"=-9.033628172356075, "Real Matrix Element"=13.866404734370539}, {"Real Matrix Element"=-9.04604901658646, "Real Matrix Element"=13.826471761683957}, {"Real Matrix Element"=-9.101229828436852, "Real Matrix Element"=13.731162907343656}, {"Real Matrix Element"=-9.142639740950186, "Real Matrix Element"=13.750750915932526}, {"Real Matrix Element"=-9.272906033638222, "Real Matrix Element"=13.623347404179313}, {"Real Matrix Element"=-9.316825252418147, "Real Matrix Element"=13.498178004676195}, {"Real Matrix Element"=-9.361231960210254, "Real Matrix Element"=13.348989409182197}, {"Real Matrix Element"=-9.439619097551835, "Real Matrix Element"=13.176468796322212}, {"Real Matrix Element"=-9.438749345177813, "Real Matrix Element"=13.09876698909348}, {"Real Matrix Element"=-9.441527299982695, "Real Matrix Element"=13.140845064475062}, {"Real Matrix Element"=-9.507918387155469, "Real Matrix Element"=12.929917848570275}, {"Real Matrix Element"=-9.4899633664178, "Real Matrix Element"=12.940765336695351}, {"Real Matrix Element"=-9.552008153103746, "Real Matrix Element"=12.837787513899904}, {"Real Matrix Element"=-9.53442766413345, "Real Matrix Element"=12.966902865524078}, {"Real Matrix Element"=-9.588948268675548, "Real Matrix Element"=12.726215900628691}, {"Real Matrix Element"=-9.663583011355795, "Real Matrix Element"=12.501523423539087}, {"Real Matrix Element"=-9.65847918432415, "Real Matrix Element"=12.529203496462221}, {"Real Matrix Element"=-9.616608831907893, "Real Matrix Element"=12.523872479546519}, {"Real Matrix Element"=-9.664990017122054, "Real Matrix Element"=12.46120046684089}, {"Real Matrix Element"=-9.689403243643538, "Real Matrix Element"=12.41941350651441}, {"Real Matrix Element"=-9.680902808260875, "Real Matrix Element"=12.470326128473157}, {"Real Matrix Element"=-9.790077408098906, "Real Matrix Element"=11.991627836860527}, {"Real Matrix Element"=-9.748058925769437, "Real Matrix Element"=12.102152734956432}, {"Real Matrix Element"=-9.823144998021322, "Real Matrix Element"=11.805492409999692}, {"Real Matrix Element"=-9.687119684296322, "Real Matrix Element"=11.359966425225359}, {"Real Matrix Element"=-9.751768259953707, "Real Matrix Element"=11.912149317743783}, {"Real Matrix Element"=-9.882135012151021, "Real Matrix Element"=11.714498905647757}, {"Real Matrix Element"=-9.900909419759667, "Real Matrix Element"=11.388487064073724}, {"Real Matrix Element"=-9.88888050784687, "Real Matrix Element"=11.323451509200464}, {"Real Matrix Element"=-9.925410807736219, "Real Matrix Element"=11.32835870644055}, {"Real Matrix Element"=-9.964218333912799, "Real Matrix Element"=11.117984935041259}, {"Real Matrix Element"=-9.935628492048927, "Real Matrix Element"=10.866267413716496}, {"Real Matrix Element"=-9.892821252634336, "Real Matrix Element"=10.90473676534773}, {"Real Matrix Element"=-9.86832387306563, "Real Matrix Element"=10.798200420829753}, {"Real Matrix Element"=-9.929082099860894, "Real Matrix Element"=10.764830522453984}, {"Real Matrix Element"=-9.919490036176747, "Real Matrix Element"=10.535745346450652}, {"Real Matrix Element"=-9.9486859295269, "Real Matrix Element"=10.551399755916371}, {"Real Matrix Element"=-9.925961654218693, "Real Matrix Element"=10.536678196197943}, {"Real Matrix Element"=-9.903128577862049, "Real Matrix Element"=10.460066754563963}, {"Real Matrix Element"=-9.964924851111109, "Real Matrix Element"=10.54382926217752}, {"Real Matrix Element"=-9.969160087851126, "Real Matrix Element"=10.45375056609254}, {"Real Matrix Element"=-9.91080218532036, "Real Matrix Element"=10.343656726424491}, {"Real Matrix Element"=-9.85292860657401, "Real Matrix Element"=10.236578434956833}, {"Real Matrix Element"=-9.889155203225133, "Real Matrix Element"=9.988087484180248}, {"Real Matrix Element"=-9.870291176639551, "Real Matrix Element"=9.695733226391777}, {"Real Matrix Element"=-9.863770290590983, "Real Matrix Element"=9.64052348491733}, {"Real Matrix Element"=-9.871339272800107, "Real Matrix Element"=9.62859899666055}, {"Real Matrix Element"=-9.860207843026556, "Real Matrix Element"=9.190307780920994}, {"Real Matrix Element"=-9.845054385919727, "Real Matrix Element"=9.140757544925142}, {"Real Matrix Element"=-9.840152579856525, "Real Matrix Element"=9.161983105044573}, {"Real Matrix Element"=-9.824422480110215, "Real Matrix Element"=9.152742100638456}, {"Real Matrix Element"=-9.832635243157402, "Real Matrix Element"=9.095380333996147}, {"Real Matrix Element"=-9.847510136907843, "Real Matrix Element"=9.128398196755574}, {"Real Matrix Element"=-9.685219689279036, "Real Matrix Element"=8.664855587621863}, {"Real Matrix Element"=-9.710010733341566, "Real Matrix Element"=8.667992764944568}, {"Real Matrix Element"=-9.699723488316309, "Real Matrix Element"=8.447839420987114}, {"Real Matrix Element"=-9.744172863896251, "Real Matrix Element"=8.629624179132312}, {"Real Matrix Element"=-9.743011381603814, "Real Matrix Element"=8.555283433988944}, {"Real Matrix Element"=-9.77606000992399, "Real Matrix Element"=8.351688187508161}, {"Real Matrix Element"=-9.694349476669203, "Real Matrix Element"=8.185528786499576}, {"Real Matrix Element"=-9.620994351989884, "Real Matrix Element"=8.061756874574638}, {"Real Matrix Element"=-9.566844018955424, "Real Matrix Element"=7.846516370586158}, {"Real Matrix Element"=-9.59821506672264, "Real Matrix Element"=7.954859888164237}, {"Real Matrix Element"=-9.55387171110457, "Real Matrix Element"=7.7678174993235904}, {"Real Matrix Element"=-9.579363216184452, "Real Matrix Element"=7.800539592577933}, {"Real Matrix Element"=-9.595760755314881, "Real Matrix Element"=7.758405549155411}, {"Real Matrix Element"=-9.581374939215609, "Real Matrix Element"=7.6633969632017624}, {"Real Matrix Element"=-9.5202454956336, "Real Matrix Element"=7.445286887116947}, {"Real Matrix Element"=-9.543442384724043, "Real Matrix Element"=7.298261935412495}, {"Real Matrix Element"=-9.53454666092335, "Real Matrix Element"=7.136237223778328}, {"Real Matrix Element"=-9.556772372391219, "Real Matrix Element"=7.337836644679887}, {"Real Matrix Element"=-9.53864241690208, "Real Matrix Element"=7.1408900897714105}, {"Real Matrix Element"=-9.56658327678482, "Real Matrix Element"=7.044649634457716}, {"Real Matrix Element"=-9.570874338893901, "Real Matrix Element"=6.963449886207173}, {"Real Matrix Element"=-9.429465711563042, "Real Matrix Element"=6.661848006895548}, {"Real Matrix Element"=-9.428042278090976, "Real Matrix Element"=6.593605470977914}, {"Real Matrix Element"=-9.334396891272643, "Real Matrix Element"=6.506235338117513}, {"Real Matrix Element"=-9.236302991916991, "Real Matrix Element"=6.414600237002674}, {"Real Matrix Element"=-9.205298086496173, "Real Matrix Element"=6.401580106408379}, {"Real Matrix Element"=-9.16761250590211, "Real Matrix Element"=6.289360848805674}, {"Real Matrix Element"=-9.196697213892403, "Real Matrix Element"=6.295991843952822}, {"Real Matrix Element"=-9.093849953482003, "Real Matrix Element"=6.175604937329429}, {"Real Matrix Element"=-9.121811653039588, "Real Matrix Element"=6.1279694463025765}, {"Real Matrix Element"=-9.093191338985443, "Real Matrix Element"=6.002553999906821}, {"Real Matrix Element"=-9.125800308346756, "Real Matrix Element"=6.086374754193676}, {"Real Matrix Element"=-9.039493417166895, "Real Matrix Element"=5.902743844225093}, {"Real Matrix Element"=-9.002638158338971, "Real Matrix Element"=5.822507307736133}, {"Real Matrix Element"=-8.716880218832562, "Real Matrix Element"=5.594745327036123}, {"Real Matrix Element"=-8.762169650136814, "Real Matrix Element"=5.576085564357628}, {"Real Matrix Element"=-8.818912600721744, "Real Matrix Element"=5.6046906608515625}, {"Real Matrix Element"=-8.794660673117287, "Real Matrix Element"=5.500709013101367}, {"Real Matrix Element"=-8.801407638234533, "Real Matrix Element"=5.423470383849976}, {"Real Matrix Element"=-8.792273860009324, "Real Matrix Element"=5.3374503347805105}, {"Real Matrix Element"=-8.690222121448, "Real Matrix Element"=5.126326086026486}, {"Real Matrix Element"=-8.65986764347385, "Real Matrix Element"=5.077433753158627}, {"Real Matrix Element"=-8.57159158186599, "Real Matrix Element"=4.9319923140617234}, {"Real Matrix Element"=-8.454122524827369, "Real Matrix Element"=4.6561744106120795}, {"Real Matrix Element"=-8.404791384464085, "Real Matrix Element"=4.643695661123129}, {"Real Matrix Element"=-8.4162933210205, "Real Matrix Element"=4.69600547991946}, {"Real Matrix Element"=-8.30236127627309, "Real Matrix Element"=4.433444264825811}, {"Real Matrix Element"=-8.311958931476608, "Real Matrix Element"=4.460911798351172}, {"Real Matrix Element"=-8.15602702389522, "Real Matrix Element"=4.161249857753865}, {"Real Matrix Element"=-8.245429127394113, "Real Matrix Element"=4.317292586733914}, {"Real Matrix Element"=-8.151900663355969, "Real Matrix Element"=4.160863747741385}, {"Real Matrix Element"=-8.137460903109433, "Real Matrix Element"=4.160272214201775}, {"Real Matrix Element"=-8.135393198735516, "Real Matrix Element"=4.141687242861944}, {"Real Matrix Element"=-7.957489201926172, "Real Matrix Element"=3.9710092983704466}, {"Real Matrix Element"=-7.931595279053337, "Real Matrix Element"=4.032303213595297}, {"Real Matrix Element"=-7.840856639153985, "Real Matrix Element"=3.928963904581966}, {"Real Matrix Element"=-7.780518738103036, "Real Matrix Element"=3.898321684286224}, {"Real Matrix Element"=-7.765034954557837, "Real Matrix Element"=3.8908996558234503}, {"Real Matrix Element"=-7.616303023575313, "Real Matrix Element"=3.7455066528028103}, {"Real Matrix Element"=-7.411740072861701, "Real Matrix Element"=3.591511044215894}, {"Real Matrix Element"=-7.372289137511588, "Real Matrix Element"=3.5902570774057474}, {"Real Matrix Element"=-7.367213551969565, "Real Matrix Element"=3.53256200543927}, {"Real Matrix Element"=-7.230151629317489, "Real Matrix Element"=3.4103754939171296}, {"Real Matrix Element"=-7.142198648397332, "Real Matrix Element"=3.267919432593225}, {"Real Matrix Element"=-7.142622682052703, "Real Matrix Element"=3.2158024949626767}, {"Real Matrix Element"=-7.077975740842653, "Real Matrix Element"=2.960883565502989}, {"Real Matrix Element"=-7.11149409519979, "Real Matrix Element"=2.980434960583258}, {"Real Matrix Element"=-6.946063501923866, "Real Matrix Element"=2.668435348885316}, {"Real Matrix Element"=-6.907635288605566, "Real Matrix Element"=2.570212672441143}, {"Real Matrix Element"=-6.937947678681285, "Real Matrix Element"=2.6455401725123653}, {"Real Matrix Element"=-6.979605265473616, "Real Matrix Element"=2.82279844717505}, {"Real Matrix Element"=-6.975030204189117, "Real Matrix Element"=2.863117775702541}, {"Real Matrix Element"=-6.933628586240636, "Real Matrix Element"=2.717192874460288}, {"Real Matrix Element"=-6.823557832451774, "Real Matrix Element"=2.452131450843491}, {"Real Matrix Element"=-6.578164566342432, "Real Matrix Element"=2.359399768641936}, {"Real Matrix Element"=-6.31201991428602, "Real Matrix Element"=2.2370288696605045}, {"Real Matrix Element"=-6.3451049609711845, "Real Matrix Element"=2.259807114786354}, {"Real Matrix Element"=-6.245189126780757, "Real Matrix Element"=2.1981880375955942}, {"Real Matrix Element"=-6.289139915750641, "Real Matrix Element"=2.2254617046123615}, {"Real Matrix Element"=-6.183826762230907, "Real Matrix Element"=2.1465455275287844}, {"Real Matrix Element"=-6.102945756325922, "Real Matrix Element"=2.0835206336671632}, {"Real Matrix Element"=-5.996404460928842, "Real Matrix Element"=1.9942416958718912}, {"Real Matrix Element"=-5.8307561687410825, "Real Matrix Element"=1.8425164047946476}, {"Real Matrix Element"=-5.693729364251016, "Real Matrix Element"=1.7710322036667696}, {"Real Matrix Element"=-5.762813053330886, "Real Matrix Element"=1.80576202182336}, {"Real Matrix Element"=-5.675712861782517, "Real Matrix Element"=1.7433626328452454}, {"Real Matrix Element"=-5.49821900230417, "Real Matrix Element"=1.7249400472367766}, {"Real Matrix Element"=-5.472716058727373, "Real Matrix Element"=1.7120986083674588}, {"Real Matrix Element"=-5.580833108782727, "Real Matrix Element"=1.774284898621329}, {"Real Matrix Element"=-5.4891921354582545, "Real Matrix Element"=1.7269166347033162}, {"Real Matrix Element"=-5.381151658819562, "Real Matrix Element"=1.6796630738975014}, {"Real Matrix Element"=-5.237641882725536, "Real Matrix Element"=1.6199357679285364}, {"Real Matrix Element"=-4.938874164189613, "Real Matrix Element"=1.2683575766135806}, {"Real Matrix Element"=-4.91499289524495, "Real Matrix Element"=1.2017318696335924}, {"Real Matrix Element"=-4.936663355050133, "Real Matrix Element"=1.2557670296443573}, {"Real Matrix Element"=-4.889440927650259, "Real Matrix Element"=1.302121028272718}, {"Real Matrix Element"=-4.861355581363706, "Real Matrix Element"=1.3060839806437174}, {"Real Matrix Element"=-4.784687131527333, "Real Matrix Element"=1.2180865923885313}, {"Real Matrix Element"=-4.712818693402973, "Real Matrix Element"=1.173795431143632}, {"Real Matrix Element"=-4.477845438933498, "Real Matrix Element"=0.9959726592717439}, {"Real Matrix Element"=-4.445164537014579, "Real Matrix Element"=0.9778633039076446}, {"Real Matrix Element"=-4.304288755638437, "Real Matrix Element"=0.9583772463781385}, {"Real Matrix Element"=-4.2466059092384665, "Real Matrix Element"=0.9116335298363291}, {"Real Matrix Element"=-4.229375501080681, "Real Matrix Element"=0.9042259899498809}, {"Real Matrix Element"=-4.049954398622778, "Real Matrix Element"=0.8537058599867107}, {"Real Matrix Element"=-3.8194721591332277, "Real Matrix Element"=0.978507297971665}, {"Real Matrix Element"=-3.999492858425133, "Real Matrix Element"=0.9323873016084036}, {"Real Matrix Element"=-3.828984577462761, "Real Matrix Element"=0.8775450629203853}, {"Real Matrix Element"=-3.871205075688366, "Real Matrix Element"=0.8588025984039368}, {"Real Matrix Element"=-3.6709434403160497, "Real Matrix Element"=0.7972989450575733}, {"Real Matrix Element"=-3.5192320672533186, "Real Matrix Element"=0.7173372534722566}, {"Real Matrix Element"=-3.345507073599771, "Real Matrix Element"=0.6524612681176445}, {"Real Matrix Element"=-3.348266669656683, "Real Matrix Element"=0.6684333599677963}, {"Real Matrix Element"=-3.1875146910386354, "Real Matrix Element"=0.6114704017642564}, {"Real Matrix Element"=-3.0404805525489955, "Real Matrix Element"=0.5207978587052569}, {"Real Matrix Element"=-2.988950173848367, "Real Matrix Element"=0.49700017820196235}, {"Real Matrix Element"=-2.8338442902367302, "Real Matrix Element"=0.4472615050378237}, {"Real Matrix Element"=-2.685899306266628, "Real Matrix Element"=0.3294281364304737}, {"Real Matrix Element"=-2.844499084827324, "Real Matrix Element"=0.4243618502599534}, {"Real Matrix Element"=-2.5914315375213226, "Real Matrix Element"=0.32166309791325287}, {"Real Matrix Element"=-2.4084666194623536, "Real Matrix Element"=0.21393369651678448}, {"Real Matrix Element"=-2.2821301688759674, "Real Matrix Element"=0.20989734498023896}, {"Real Matrix Element"=-2.0704099290057583, "Real Matrix Element"=0.04872971624650477}, {"Real Matrix Element"=-2.211762742095328, "Real Matrix Element"=0.16775354587269842}, {"Real Matrix Element"=-2.1585307561154443, "Real Matrix Element"=0.18416501292381265}, {"Real Matrix Element"=-1.8962194141145476, "Real Matrix Element"=0.17799606856185363}, {"Real Matrix Element"=-1.8979975095246266, "Real Matrix Element"=0.15080040734614927}, {"Real Matrix Element"=-1.9195677507148479, "Real Matrix Element"=0.15727813351418743}, {"Real Matrix Element"=-1.9051820105067776, "Real Matrix Element"=0.14046928484745663}, {"Real Matrix Element"=-1.673496549788643, "Real Matrix Element"=0.20405990424022147}, {"Real Matrix Element"=-1.7484696831182176, "Real Matrix Element"=0.1722039923175607}, {"Real Matrix Element"=-1.2981358494055688, "Real Matrix Element"=0.1996633688958312}, {"Real Matrix Element"=-1.291846177225915, "Real Matrix Element"=0.21317397616247113}, {"Real Matrix Element"=-1.1897678559056013, "Real Matrix Element"=0.27760485346088914}, {"Real Matrix Element"=-1.112898671453695, "Real Matrix Element"=0.24323677110579384}, {"Real Matrix Element"=-1.159725832784002, "Real Matrix Element"=0.23996740089066398}, {"Real Matrix Element"=-1.0104198572781093, "Real Matrix Element"=0.2686011059698839}, {"Real Matrix Element"=-1.0769022320075783, "Real Matrix Element"=0.20932632856437794}, {"Real Matrix Element"=-0.9605746306541683, "Real Matrix Element"=0.22575706856279393}, {"Real Matrix Element"=-0.6598891055426613, "Real Matrix Element"=0.21961176698627802}, {"Real Matrix Element"=-0.5940983339974449, "Real Matrix Element"=0.18920303348373524}, {"Real Matrix Element"=-0.4686115310467917, "Real Matrix Element"=0.11354674938274689}, {"Real Matrix Element"=-0.385567661366674, "Real Matrix Element"=0.08515402668212922}, {"Real Matrix Element"=-0.4541449312553905, "Real Matrix Element"=0.08127859195148279}, {"Real Matrix Element"=-0.33701803408294617, "Real Matrix Element"=0.06392028511039594}, {"Real Matrix Element"=-0.25009242998944714, "Real Matrix Element"=0.06552582806209707}, {"Real Matrix Element"=-0.004358422272312156, "Real Matrix Element"=0.0709727489552854}, {"Real Matrix Element"=0.056862391330129866, "Real Matrix Element"=0.0881150794775779}, {"Real Matrix Element"=0.2806716415817157, "Real Matrix Element"=0.06769301899334014}, {"Real Matrix Element"=0.37342055474424174, "Real Matrix Element"=0.033925906300860745}, {"Real Matrix Element"=0.5086651328136088, "Real Matrix Element"=-0.018257465620279325}, {"Real Matrix Element"=0.4987791510651565, "Real Matrix Element"=0.088292923931462}, {"Real Matrix Element"=0.8089384541486138, "Real Matrix Element"=0.0817207244688458}, {"Real Matrix Element"=0.5934064996824356, "Real Matrix Element"=0.042278953597911104}, {"Real Matrix Element"=0.7493885472973185, "Real Matrix Element"=0.09845399748143607}, {"Real Matrix Element"=1.0643031261728126, "Real Matrix Element"=0.07843151459066114}, {"Real Matrix Element"=1.0303345159539494, "Real Matrix Element"=0.052814892493281446}, {"Real Matrix Element"=1.1860003529012708, "Real Matrix Element"=0.15463053943029373}, {"Real Matrix Element"=1.334645615102202, "Real Matrix Element"=0.11271959661411662}, {"Real Matrix Element"=1.386357495972317, "Real Matrix Element"=0.05818196843373065}, {"Real Matrix Element"=1.3345004402476672, "Real Matrix Element"=0.08709692595855081}, {"Real Matrix Element"=1.5049686665604514, "Real Matrix Element"=0.18023805426398987}, {"Real Matrix Element"=1.796113604770399, "Real Matrix Element"=0.2727782406974419}, {"Real Matrix Element"=1.8253471527009015, "Real Matrix Element"=0.19636701402589218}, {"Real Matrix Element"=2.0298803125778355, "Real Matrix Element"=0.2050945998577422}, {"Real Matrix Element"=2.1131441886044104, "Real Matrix Element"=0.2575817154140886}, {"Real Matrix Element"=2.088441783058089, "Real Matrix Element"=0.2832396419541013}, {"Real Matrix Element"=2.234641467649826, "Real Matrix Element"=0.26566514720175244}, {"Real Matrix Element"=2.0491938814572426, "Real Matrix Element"=0.2454545667123883}, {"Real Matrix Element"=2.3192377786228273, "Real Matrix Element"=0.2698193892969923}, {"Real Matrix Element"=2.2908220556332197, "Real Matrix Element"=0.33992331471996656}, {"Real Matrix Element"=2.749769738871576, "Real Matrix Element"=0.36663796051038444}, {"Real Matrix Element"=2.5095755772389685, "Real Matrix Element"=0.3516819852032583}, {"Real Matrix Element"=2.6579948809961476, "Real Matrix Element"=0.3635906673686652}, {"Real Matrix Element"=2.782886990484266, "Real Matrix Element"=0.32715481264681634}, {"Real Matrix Element"=2.9056649569674744, "Real Matrix Element"=0.3478152773830737}, {"Real Matrix Element"=3.1364357083529795, "Real Matrix Element"=0.45374987809516737}, {"Real Matrix Element"=3.1103538340349535, "Real Matrix Element"=0.49977143329327633}, {"Real Matrix Element"=3.117261604707535, "Real Matrix Element"=0.4736150279122502}, {"Real Matrix Element"=3.335182768192005, "Real Matrix Element"=0.5231718703333259}, {"Real Matrix Element"=3.5453586016075795, "Real Matrix Element"=0.5920353792857493}, {"Real Matrix Element"=3.653800229067975, "Real Matrix Element"=0.6800613075573605}, {"Real Matrix Element"=3.645748068346742, "Real Matrix Element"=0.6677551019630433}, {"Real Matrix Element"=3.6678640128302913, "Real Matrix Element"=0.7905746893563288}, {"Real Matrix Element"=3.7255578910203577, "Real Matrix Element"=0.8009521002747795}, {"Real Matrix Element"=3.827199469075306, "Real Matrix Element"=0.9163162386941972}, {"Real Matrix Element"=4.009474904646554, "Real Matrix Element"=0.9763536140198523}, {"Real Matrix Element"=3.9516757822313004, "Real Matrix Element"=0.8858919070997742}, {"Real Matrix Element"=4.011318809383869, "Real Matrix Element"=0.9707558618492947}, {"Real Matrix Element"=4.073332872811307, "Real Matrix Element"=0.9882266731422583}, {"Real Matrix Element"=4.167641985098122, "Real Matrix Element"=0.9961419976473832}, {"Real Matrix Element"=4.205435438599394, "Real Matrix Element"=0.9182682444426271}, {"Real Matrix Element"=4.473464752914125, "Real Matrix Element"=1.0718144913275691}, {"Real Matrix Element"=4.647422100115804, "Real Matrix Element"=1.21299923008441}, {"Real Matrix Element"=4.698994211726901, "Real Matrix Element"=1.241286374113763}, {"Real Matrix Element"=4.813521221898043, "Real Matrix Element"=1.3313419943647602}, {"Real Matrix Element"=5.056692600492057, "Real Matrix Element"=1.4210304151964794}, {"Real Matrix Element"=5.040038976022885, "Real Matrix Element"=1.3372693533279365}, {"Real Matrix Element"=5.017309648278492, "Real Matrix Element"=1.3329513836094742}, {"Real Matrix Element"=5.208159687565554, "Real Matrix Element"=1.4517235904136907}, {"Real Matrix Element"=5.284311534109123, "Real Matrix Element"=1.4823740979822448}, {"Real Matrix Element"=5.502729131930209, "Real Matrix Element"=1.5799588831042737}, {"Real Matrix Element"=5.437326733877642, "Real Matrix Element"=1.5458339159022392}, {"Real Matrix Element"=5.394055764991277, "Real Matrix Element"=1.5340772630494226}, {"Real Matrix Element"=5.4048214934320065, "Real Matrix Element"=1.5144892546522504}, {"Real Matrix Element"=5.3534648866887435, "Real Matrix Element"=1.517370294116197}, {"Real Matrix Element"=5.654003552524832, "Real Matrix Element"=1.6353526103659972}, {"Real Matrix Element"=5.687936062183252, "Real Matrix Element"=1.6624365534720413}, {"Real Matrix Element"=6.044993982923136, "Real Matrix Element"=1.8398205999029362}, {"Real Matrix Element"=5.9978369899196915, "Real Matrix Element"=1.8600051093480818}, {"Real Matrix Element"=6.135421317258252, "Real Matrix Element"=2.082481552326532}, {"Real Matrix Element"=6.243696325817253, "Real Matrix Element"=2.131176659180894}, {"Real Matrix Element"=6.314994981032224, "Real Matrix Element"=2.135166697749251}, {"Real Matrix Element"=6.17597630426492, "Real Matrix Element"=2.0889623707741865}, {"Real Matrix Element"=6.364545796315758, "Real Matrix Element"=2.2339468718828823}, {"Real Matrix Element"=6.533072833531854, "Real Matrix Element"=2.1798656095341187}, {"Real Matrix Element"=6.3957189871986975, "Real Matrix Element"=2.28077244166509}, {"Real Matrix Element"=6.590007262141513, "Real Matrix Element"=2.490560468010627}, {"Real Matrix Element"=6.695409533281442, "Real Matrix Element"=2.5822626561678512}, {"Real Matrix Element"=6.737224300631012, "Real Matrix Element"=2.5838330862165395}, {"Real Matrix Element"=6.827122522687116, "Real Matrix Element"=2.663220749720166}, {"Real Matrix Element"=6.882624518186017, "Real Matrix Element"=2.7248366269202453}, {"Real Matrix Element"=6.918603149302258, "Real Matrix Element"=2.72213896893756}, {"Real Matrix Element"=6.991060736294549, "Real Matrix Element"=2.8654738496072145}, {"Real Matrix Element"=7.060289243947935, "Real Matrix Element"=3.011231011905791}, {"Real Matrix Element"=7.055444995956011, "Real Matrix Element"=2.963684032149325}, {"Real Matrix Element"=7.174837074097535, "Real Matrix Element"=3.0701358617057237}, {"Real Matrix Element"=7.392880439977292, "Real Matrix Element"=3.184798750276924}, {"Real Matrix Element"=7.441859663452126, "Real Matrix Element"=3.321200326164854}, {"Real Matrix Element"=7.47067934175207, "Real Matrix Element"=3.338287887234092}, {"Real Matrix Element"=7.39911730267326, "Real Matrix Element"=3.2686602543506638}, {"Real Matrix Element"=7.479251250105851, "Real Matrix Element"=3.398872417052792}, {"Real Matrix Element"=7.504920361037026, "Real Matrix Element"=3.3994439599708044}, {"Real Matrix Element"=7.617897752292696, "Real Matrix Element"=3.495005168158899}, {"Real Matrix Element"=7.651286073273848, "Real Matrix Element"=3.5774395398657837}, {"Real Matrix Element"=7.739950496239503, "Real Matrix Element"=3.6527734145094866}, {"Real Matrix Element"=7.892251575021676, "Real Matrix Element"=3.84526759555801}, {"Real Matrix Element"=7.910473314338433, "Real Matrix Element"=3.839807020012921}, {"Real Matrix Element"=7.931569933001409, "Real Matrix Element"=3.8513863798486274}, {"Real Matrix Element"=7.991555303786628, "Real Matrix Element"=4.137334548345187}, {"Real Matrix Element"=8.029802725951564, "Real Matrix Element"=3.9878060002145186}, {"Real Matrix Element"=8.082801274117664, "Real Matrix Element"=4.156953164451653}, {"Real Matrix Element"=8.308088952161265, "Real Matrix Element"=4.323047838161546}, {"Real Matrix Element"=8.343590446277053, "Real Matrix Element"=4.501191612504699}, {"Real Matrix Element"=8.393302438291649, "Real Matrix Element"=4.53974634637022}, {"Real Matrix Element"=8.445253389828574, "Real Matrix Element"=4.658913377705868}, {"Real Matrix Element"=8.391084624199513, "Real Matrix Element"=4.620020530855246}, {"Real Matrix Element"=8.408210003282406, "Real Matrix Element"=4.677274033460871}, {"Real Matrix Element"=8.401670096442947, "Real Matrix Element"=4.6851537546848565}, {"Real Matrix Element"=8.428632543132323, "Real Matrix Element"=4.769874744172709}, {"Real Matrix Element"=8.470442643706425, "Real Matrix Element"=4.877474729011388}, {"Real Matrix Element"=8.558818732688854, "Real Matrix Element"=5.157084949439115}, {"Real Matrix Element"=8.506870181969823, "Real Matrix Element"=4.9176490359078615}, {"Real Matrix Element"=8.539865386861141, "Real Matrix Element"=5.0322306209061125}, {"Real Matrix Element"=8.549873900638975, "Real Matrix Element"=5.028154558901196}, {"Real Matrix Element"=8.660639366069136, "Real Matrix Element"=5.263169380599752}, {"Real Matrix Element"=8.581428415850402, "Real Matrix Element"=5.1925510074827805}, {"Real Matrix Element"=8.701530572480015, "Real Matrix Element"=5.5391681005944875}, {"Real Matrix Element"=8.80070575643965, "Real Matrix Element"=5.787796011578065}, {"Real Matrix Element"=8.958151458737191, "Real Matrix Element"=5.892696700263682}, {"Real Matrix Element"=9.06108236094766, "Real Matrix Element"=6.0109519910138385}, {"Real Matrix Element"=9.06592212334002, "Real Matrix Element"=5.963204537369079}, {"Real Matrix Element"=9.248725252163732, "Real Matrix Element"=6.312163268413845}, {"Real Matrix Element"=9.18572461493545, "Real Matrix Element"=6.205613658194413}, {"Real Matrix Element"=9.155608225774095, "Real Matrix Element"=6.184061853557403}, {"Real Matrix Element"=9.167672123533894, "Real Matrix Element"=6.1732743691917475}, {"Real Matrix Element"=9.239122739227549, "Real Matrix Element"=6.307472012252517}, {"Real Matrix Element"=9.317589393529584, "Real Matrix Element"=6.5024709529422005}, {"Real Matrix Element"=9.336358337997723, "Real Matrix Element"=6.535274738436384}, {"Real Matrix Element"=9.31226063591658, "Real Matrix Element"=6.507830502104101}, {"Real Matrix Element"=9.521217527298111, "Real Matrix Element"=6.818017974269288}, {"Real Matrix Element"=9.526274396490242, "Real Matrix Element"=6.944366830633533}, {"Real Matrix Element"=9.463965266725051, "Real Matrix Element"=7.0443834439523165}, {"Real Matrix Element"=9.583310261858015, "Real Matrix Element"=7.181019170549652}, {"Real Matrix Element"=9.71405700210094, "Real Matrix Element"=7.30467982920008}, {"Real Matrix Element"=9.651801651876788, "Real Matrix Element"=7.217199163130451}, {"Real Matrix Element"=9.732226473233137, "Real Matrix Element"=7.427943621926604}, {"Real Matrix Element"=9.872959446755818, "Real Matrix Element"=7.670105101160749}, {"Real Matrix Element"=9.741996939944361, "Real Matrix Element"=7.4729633385636145}, {"Real Matrix Element"=9.874768469610222, "Real Matrix Element"=7.701031757117981}, {"Real Matrix Element"=9.851448865412012, "Real Matrix Element"=7.68571284661257}, {"Real Matrix Element"=9.921388930537328, "Real Matrix Element"=7.848762721384946}, {"Real Matrix Element"=9.860200569467583, "Real Matrix Element"=7.752805704889625}, {"Real Matrix Element"=9.923083866533553, "Real Matrix Element"=7.958073312642442}, {"Real Matrix Element"=9.834873134958144, "Real Matrix Element"=7.9769494158792345}, {"Real Matrix Element"=9.862374950245371, "Real Matrix Element"=8.198184384916557}, {"Real Matrix Element"=9.921625947052272, "Real Matrix Element"=8.368788470007265}, {"Real Matrix Element"=9.935007771737114, "Real Matrix Element"=8.292376359076215}, {"Real Matrix Element"=10.115991283702483, "Real Matrix Element"=8.618664997002945}, {"Real Matrix Element"=9.968281630743501, "Real Matrix Element"=8.811937104770522}, {"Real Matrix Element"=9.945401385264168, "Real Matrix Element"=8.81586387190795}, {"Real Matrix Element"=10.057524803858092, "Real Matrix Element"=8.97130897472962}, {"Real Matrix Element"=9.996227559661884, "Real Matrix Element"=8.820309131698592}, {"Real Matrix Element"=10.0967766845661, "Real Matrix Element"=9.080835139105117}, {"Real Matrix Element"=10.04360152684346, "Real Matrix Element"=9.109386748324958}, {"Real Matrix Element"=9.947399575431245, "Real Matrix Element"=8.981901640625598}, {"Real Matrix Element"=9.943688006822917, "Real Matrix Element"=9.287661233088905}, {"Real Matrix Element"=9.845943521642214, "Real Matrix Element"=9.253519401111651}, {"Real Matrix Element"=9.961174515060794, "Real Matrix Element"=9.407464567679183}, {"Real Matrix Element"=10.029935835355706, "Real Matrix Element"=9.661983300052214}, {"Real Matrix Element"=10.10050118829862, "Real Matrix Element"=9.751307852894556}, {"Real Matrix Element"=10.087155599981381, "Real Matrix Element"=9.757386167320666}, {"Real Matrix Element"=10.265343294583388, "Real Matrix Element"=9.991441469387244}, {"Real Matrix Element"=10.235314443241014, "Real Matrix Element"=10.032551915523374}, {"Real Matrix Element"=10.177098441092548, "Real Matrix Element"=10.017806502378209}, {"Real Matrix Element"=10.201540049853964, "Real Matrix Element"=10.159550503835314}, {"Real Matrix Element"=10.067435820788544, "Real Matrix Element"=10.4146170872031}, {"Real Matrix Element"=10.057166633819763, "Real Matrix Element"=10.45146629303184}, {"Real Matrix Element"=10.065351553734802, "Real Matrix Element"=10.519877507818594}, {"Real Matrix Element"=10.066288570297546, "Real Matrix Element"=10.467395229469107}, {"Real Matrix Element"=10.052721567440464, "Real Matrix Element"=10.746080483474062}, {"Real Matrix Element"=10.062355128273063, "Real Matrix Element"=10.57005365381229}, {"Real Matrix Element"=10.045304325028928, "Real Matrix Element"=10.821371587392822}, {"Real Matrix Element"=10.083205828585477, "Real Matrix Element"=10.915529985169119}, {"Real Matrix Element"=10.027972047318785, "Real Matrix Element"=11.125421533054627}, {"Real Matrix Element"=10.085163542434609, "Real Matrix Element"=11.096870689698116}, {"Real Matrix Element"=9.980981145684785, "Real Matrix Element"=11.152505394190493}, {"Real Matrix Element"=9.917590266941566, "Real Matrix Element"=11.269476180732907}, {"Real Matrix Element"=9.91227602245228, "Real Matrix Element"=11.320643536369689}, {"Real Matrix Element"=9.754296757636823, "Real Matrix Element"=11.549621445853054}, {"Real Matrix Element"=9.716228999480041, "Real Matrix Element"=11.591239125083625}, {"Real Matrix Element"=9.784571788088417, "Real Matrix Element"=11.888426885054972}, {"Real Matrix Element"=9.684691855728708, "Real Matrix Element"=11.816042275828579}, {"Real Matrix Element"=9.723627286527698, "Real Matrix Element"=12.012568621671894}, {"Real Matrix Element"=9.763225197810009, "Real Matrix Element"=12.054090227836916}, {"Real Matrix Element"=9.776611375654474, "Real Matrix Element"=12.189369778491287}, {"Real Matrix Element"=9.768048808305112, "Real Matrix Element"=12.203207220197156}, {"Real Matrix Element"=9.787134659906407, "Real Matrix Element"=12.1414090164173}, {"Real Matrix Element"=9.787915916736283, "Real Matrix Element"=12.403572313457753}, {"Real Matrix Element"=9.729628095182271, "Real Matrix Element"=12.493560366122633}, {"Real Matrix Element"=9.690692077667794, "Real Matrix Element"=12.542080680157813}, {"Real Matrix Element"=9.652012143635213, "Real Matrix Element"=12.61276937247362}, {"Real Matrix Element"=9.545851884300316, "Real Matrix Element"=12.749340093225962}, {"Real Matrix Element"=9.61225449165834, "Real Matrix Element"=12.93916921297777}, {"Real Matrix Element"=9.565079677246908, "Real Matrix Element"=13.004833162724237}, {"Real Matrix Element"=9.576363126015238, "Real Matrix Element"=13.107476051310702}, {"Real Matrix Element"=9.587810109896122, "Real Matrix Element"=13.098114768004669}, {"Real Matrix Element"=9.545899033042371, "Real Matrix Element"=13.285439440258092}, {"Real Matrix Element"=9.461390020260186, "Real Matrix Element"=13.498352791435657}, {"Real Matrix Element"=9.475907126427042, "Real Matrix Element"=13.536398609663214}, {"Real Matrix Element"=9.379140986161042, "Real Matrix Element"=13.706375947383366}, {"Real Matrix Element"=9.343101571105583, "Real Matrix Element"=13.768460634204283}, {"Real Matrix Element"=9.375765574812235, "Real Matrix Element"=13.824220360005915}, {"Real Matrix Element"=9.273895369526947, "Real Matrix Element"=14.065732906310284}, {"Real Matrix Element"=9.238562839930378, "Real Matrix Element"=14.11712205090259}, {"Real Matrix Element"=9.247382728447244, "Real Matrix Element"=14.096459539162966}, {"Real Matrix Element"=9.11954638212646, "Real Matrix Element"=14.245059664578186}, {"Real Matrix Element"=9.089756756237309, "Real Matrix Element"=14.222713905186525}, {"Real Matrix Element"=8.950878667882005, "Real Matrix Element"=14.400886963378055}, {"Real Matrix Element"=9.025236363917527, "Real Matrix Element"=14.346658854854113}, {"Real Matrix Element"=9.012929558938918, "Real Matrix Element"=14.521470357443826}, {"Real Matrix Element"=9.005627311678046, "Real Matrix Element"=14.595577658297469}, {"Real Matrix Element"=8.822858249454136, "Real Matrix Element"=14.592858521604182}, {"Real Matrix Element"=8.768381130504123, "Real Matrix Element"=14.746867284489957}, {"Real Matrix Element"=8.713065057713415, "Real Matrix Element"=14.823270915692257}, {"Real Matrix Element"=8.799457726561565, "Real Matrix Element"=14.807500198894187}, {"Real Matrix Element"=8.683996206569592, "Real Matrix Element"=14.937837301991195}, {"Real Matrix Element"=8.668504217588383, "Real Matrix Element"=14.996730780191717}, {"Real Matrix Element"=8.51029134894619, "Real Matrix Element"=15.151343028869945}, {"Real Matrix Element"=8.511499522505524, "Real Matrix Element"=15.202750163283726}, {"Real Matrix Element"=8.403457728782884, "Real Matrix Element"=15.280491098268902}, {"Real Matrix Element"=8.379093763177933, "Real Matrix Element"=15.410468676377624}, {"Real Matrix Element"=8.260613222834033, "Real Matrix Element"=15.477135724183004}, {"Real Matrix Element"=8.14203583370747, "Real Matrix Element"=15.680896629892874}, {"Real Matrix Element"=7.999862125185345, "Real Matrix Element"=15.748397518039145}, {"Real Matrix Element"=8.050002491549659, "Real Matrix Element"=15.78285052185178}, {"Real Matrix Element"=8.04997924621621, "Real Matrix Element"=15.809726319225154}, {"Real Matrix Element"=7.854124115767891, "Real Matrix Element"=15.987693110763017}, {"Real Matrix Element"=7.839740424463557, "Real Matrix Element"=16.019619773692266}, {"Real Matrix Element"=7.868380043167934, "Real Matrix Element"=15.986801824175085}, {"Real Matrix Element"=7.651254874605333, "Real Matrix Element"=16.27050373944315}, {"Real Matrix Element"=7.740515917733237, "Real Matrix Element"=16.153865386225416}, {"Real Matrix Element"=7.684508775760696, "Real Matrix Element"=16.245083069672773}, {"Real Matrix Element"=7.500600081883108, "Real Matrix Element"=16.40698642893933}, {"Real Matrix Element"=7.36140468340194, "Real Matrix Element"=16.539863200007215}, {"Real Matrix Element"=7.432270996116548, "Real Matrix Element"=16.518780883668374}, {"Real Matrix Element"=7.344108029000622, "Real Matrix Element"=16.684009939123108}, {"Real Matrix Element"=7.198191722751275, "Real Matrix Element"=16.86496860384791}, {"Real Matrix Element"=7.380156229894206, "Real Matrix Element"=16.734470280584247}, {"Real Matrix Element"=7.296237019919352, "Real Matrix Element"=16.82801546844929}, {"Real Matrix Element"=6.969259751650961, "Real Matrix Element"=16.96083205966299}, {"Real Matrix Element"=6.946601059429115, "Real Matrix Element"=17.027887862932033}, {"Real Matrix Element"=6.880056897104314, "Real Matrix Element"=17.144061181211956}, {"Real Matrix Element"=6.910902726575327, "Real Matrix Element"=17.080074147717202}, {"Real Matrix Element"=6.887899485709661, "Real Matrix Element"=17.13290428854722}, {"Real Matrix Element"=6.712729283120207, "Real Matrix Element"=17.26571834489801}, {"Real Matrix Element"=6.745499823218749, "Real Matrix Element"=17.27928061553169}, {"Real Matrix Element"=6.716719487049669, "Real Matrix Element"=17.350694552379856}, {"Real Matrix Element"=6.611719649371916, "Real Matrix Element"=17.59706181631262}, {"Real Matrix Element"=6.634585720774832, "Real Matrix Element"=17.499051363757587}, {"Real Matrix Element"=6.490094020240054, "Real Matrix Element"=17.734580199663988}, {"Real Matrix Element"=6.3515800576813835, "Real Matrix Element"=17.697719896401587}, {"Real Matrix Element"=6.466525662447988, "Real Matrix Element"=17.623788617843672}, {"Real Matrix Element"=6.298202547192715, "Real Matrix Element"=17.712844946037492}, {"Real Matrix Element"=6.36344914395392, "Real Matrix Element"=17.654748483969904}, {"Real Matrix Element"=6.035843302876096, "Real Matrix Element"=17.860458449063113}, {"Real Matrix Element"=5.912593859994829, "Real Matrix Element"=17.926457784868113}, {"Real Matrix Element"=5.988619968495865, "Real Matrix Element"=17.88652206354578}, {"Real Matrix Element"=5.913260307034307, "Real Matrix Element"=17.960742146693928}, {"Real Matrix Element"=5.820700624162123, "Real Matrix Element"=18.030471584997283}, {"Real Matrix Element"=5.543337599033096, "Real Matrix Element"=18.16642929605888}, {"Real Matrix Element"=5.363883802379263, "Real Matrix Element"=18.222899727519717}, {"Real Matrix Element"=5.403054628610711, "Real Matrix Element"=18.212552436376132}, {"Real Matrix Element"=5.2994277735369115, "Real Matrix Element"=18.293975610193964}, {"Real Matrix Element"=5.265108392336042, "Real Matrix Element"=18.366017323427425}, {"Real Matrix Element"=5.171136305175223, "Real Matrix Element"=18.44517559307985}, {"Real Matrix Element"=5.296779076410989, "Real Matrix Element"=18.34232652955345}, {"Real Matrix Element"=5.208133546929963, "Real Matrix Element"=18.440165693616414}, {"Real Matrix Element"=5.000806624320417, "Real Matrix Element"=18.56095734966771}, {"Real Matrix Element"=4.90942735454128, "Real Matrix Element"=18.67992519340265}, {"Real Matrix Element"=4.900623899838394, "Real Matrix Element"=18.679130021951504}, {"Real Matrix Element"=4.726875832596918, "Real Matrix Element"=18.80270319091632}, {"Real Matrix Element"=4.61903813496203, "Real Matrix Element"=18.921663706179483}, {"Real Matrix Element"=4.677484084166555, "Real Matrix Element"=18.8281185541888}, {"Real Matrix Element"=4.647285580087437, "Real Matrix Element"=18.937689417807626}, {"Real Matrix Element"=4.371500385252254, "Real Matrix Element"=19.007444326033276}, {"Real Matrix Element"=4.280738946286091, "Real Matrix Element"=19.070540705029117}, {"Real Matrix Element"=4.087408909280009, "Real Matrix Element"=19.146381812139975}, {"Real Matrix Element"=3.966187993833548, "Real Matrix Element"=19.14705729460426}, {"Real Matrix Element"=4.099685611944329, "Real Matrix Element"=19.129399028660654}, {"Real Matrix Element"=4.007225562088749, "Real Matrix Element"=19.173250715039984}, {"Real Matrix Element"=3.7474176174030274, "Real Matrix Element"=19.306065740255843}, {"Real Matrix Element"=3.6674430803309828, "Real Matrix Element"=19.292721246590542}, {"Real Matrix Element"=3.7007577797008397, "Real Matrix Element"=19.270200787313772}, {"Real Matrix Element"=3.578951162351194, "Real Matrix Element"=19.297073969003726}, {"Real Matrix Element"=3.3375889382343877, "Real Matrix Element"=19.40879134516953}, {"Real Matrix Element"=3.2447115833287064, "Real Matrix Element"=19.55256814501684}, {"Real Matrix Element"=3.25445795571832, "Real Matrix Element"=19.504301738166486}, {"Real Matrix Element"=3.0942092408224506, "Real Matrix Element"=19.56101816306673}, {"Real Matrix Element"=2.925364442811101, "Real Matrix Element"=19.61005398260163}, {"Real Matrix Element"=2.9229701962907124, "Real Matrix Element"=19.643768602322012}, {"Real Matrix Element"=2.7834620955902456, "Real Matrix Element"=19.698083685819967}, {"Real Matrix Element"=2.9688037581487734, "Real Matrix Element"=19.595093132097265}, {"Real Matrix Element"=2.879689191492334, "Real Matrix Element"=19.621680883608228}, {"Real Matrix Element"=2.372848651961739, "Real Matrix Element"=19.75699587546722}, {"Real Matrix Element"=2.245506053168764, "Real Matrix Element"=19.79381307171641}, {"Real Matrix Element"=2.3397667414530967, "Real Matrix Element"=19.729382829829074}, {"Real Matrix Element"=2.1143497741324904, "Real Matrix Element"=19.80740530441308}, {"Real Matrix Element"=1.9699499024780616, "Real Matrix Element"=19.809397438577548}, {"Real Matrix Element"=2.0320500870979403, "Real Matrix Element"=19.803938783397612}, {"Real Matrix Element"=1.9840277804513573, "Real Matrix Element"=19.780655620037724}, {"Real Matrix Element"=1.9349939220567032, "Real Matrix Element"=19.87086555278097}, {"Real Matrix Element"=1.8401845588316643, "Real Matrix Element"=19.890998460958578}, {"Real Matrix Element"=1.7748175152828067, "Real Matrix Element"=19.939749948744158}, {"Real Matrix Element"=1.741720002506905, "Real Matrix Element"=19.88541183916118}, {"Real Matrix Element"=1.76380850640306, "Real Matrix Element"=19.8395356113979}, {"Real Matrix Element"=1.637380462100561, "Real Matrix Element"=19.922800659574854}, {"Real Matrix Element"=1.346895681152792, "Real Matrix Element"=19.965958843360088}, {"Real Matrix Element"=1.292230869305927, "Real Matrix Element"=19.95690725544971}, {"Real Matrix Element"=1.218369798686595, "Real Matrix Element"=19.971292746979444}, {"Real Matrix Element"=1.0422657052227533, "Real Matrix Element"=20.088338983378918}, {"Real Matrix Element"=1.0774122487861166, "Real Matrix Element"=20.03579953556799}, {"Real Matrix Element"=1.0744859185079454, "Real Matrix Element"=20.033772866224076}, {"Real Matrix Element"=0.8576211501037454, "Real Matrix Element"=20.043408379386726}, {"Real Matrix Element"=0.7104348822194454, "Real Matrix Element"=20.0043706831368}, {"Real Matrix Element"=0.48614206415348366, "Real Matrix Element"=19.947343598846373}, {"Real Matrix Element"=0.3689934439197959, "Real Matrix Element"=19.95418154361023}, {"Real Matrix Element"=0.6004573149871282, "Real Matrix Element"=20.036775655997673}, {"Real Matrix Element"=0.2579255394264074, "Real Matrix Element"=19.970959749989127}, {"Real Matrix Element"=0.3022639488913275, "Real Matrix Element"=19.95744219352385}, {"Real Matrix Element"=0.10033567644612382, "Real Matrix Element"=19.97105558425893}, {"Real Matrix Element"=-0.11869771179289905, "Real Matrix Element"=19.935540102473}, {"Real Matrix Element"=-0.21863412488313486, "Real Matrix Element"=19.916878649971913}, {"Real Matrix Element"=-0.47596397363185283, "Real Matrix Element"=19.810675352920693}, {"Real Matrix Element"=-0.03253882010235312, "Real Matrix Element"=19.94479207527093}, {"Real Matrix Element"=-0.08207305147610738, "Real Matrix Element"=19.949612927220457}, {"Real Matrix Element"=-0.29310494041577306, "Real Matrix Element"=19.877749090652628}, {"Real Matrix Element"=-0.31891703753811723, "Real Matrix Element"=19.899941183533564}, {"Real Matrix Element"=-0.6749780722327472, "Real Matrix Element"=19.75546104025796}, {"Real Matrix Element"=-0.8742197840270242, "Real Matrix Element"=19.75158856679466}, {"Real Matrix Element"=-1.1114361652900582, "Real Matrix Element"=19.685348463521553}, {"Real Matrix Element"=-1.1433863549979906, "Real Matrix Element"=19.720687306159324}, {"Real Matrix Element"=-1.079595420718162, "Real Matrix Element"=19.728939504733415}, {"Real Matrix Element"=-1.1971233329710953, "Real Matrix Element"=19.72756445489966}, {"Real Matrix Element"=-1.253731860009308, "Real Matrix Element"=19.679537108053022}, {"Real Matrix Element"=-1.46478876723728, "Real Matrix Element"=19.679365815959525}, {"Real Matrix Element"=-1.5746910508034897, "Real Matrix Element"=19.74125727854582}, {"Real Matrix Element"=-1.420054283923338, "Real Matrix Element"=19.805675190310215}, {"Real Matrix Element"=-1.634332962103529, "Real Matrix Element"=19.729240489131268}, {"Real Matrix Element"=-1.834297108536761, "Real Matrix Element"=19.784947943003253}, {"Real Matrix Element"=-2.0811596320824033, "Real Matrix Element"=19.78424362525594}, {"Real Matrix Element"=-1.909903486215273, "Real Matrix Element"=19.804030164904443}, {"Real Matrix Element"=-2.161839251424535, "Real Matrix Element"=19.81182147646651}, {"Real Matrix Element"=-2.221607377475923, "Real Matrix Element"=19.821199569296077}, {"Real Matrix Element"=-2.3398627963619725, "Real Matrix Element"=19.792649861054763}, {"Real Matrix Element"=-2.5475396444467244, "Real Matrix Element"=19.772243758002304}, {"Real Matrix Element"=-2.659958602537772, "Real Matrix Element"=19.702931839451303}, {"Real Matrix Element"=-2.589811783042669, "Real Matrix Element"=19.66857700660545}, {"Real Matrix Element"=-2.6699660155627036, "Real Matrix Element"=19.68517455658433}, {"Real Matrix Element"=-2.873837906160292, "Real Matrix Element"=19.628999408196634}, {"Real Matrix Element"=-2.7287554295451746, "Real Matrix Element"=19.6530918686706}, {"Real Matrix Element"=-2.8248987575803626, "Real Matrix Element"=19.665673894745236}, {"Real Matrix Element"=-3.096483098862953, "Real Matrix Element"=19.573858246616105}, {"Real Matrix Element"=-3.459545791955244, "Real Matrix Element"=19.403483593362292}, {"Real Matrix Element"=-3.5001876490376724, "Real Matrix Element"=19.24328478439325}, {"Real Matrix Element"=-3.523855320123152, "Real Matrix Element"=19.24192421340059}, {"Real Matrix Element"=-3.6300453979043987, "Real Matrix Element"=19.21150740709184}, {"Real Matrix Element"=-3.4045610637893056, "Real Matrix Element"=19.317108542709878}, {"Real Matrix Element"=-3.547946389424415, "Real Matrix Element"=19.267408349535597}, {"Real Matrix Element"=-3.5821750828997576, "Real Matrix Element"=19.283756869681262}, {"Real Matrix Element"=-3.712498183449937, "Real Matrix Element"=19.169114353142678}, {"Real Matrix Element"=-3.7586731565250533, "Real Matrix Element"=19.122697668238295}, {"Real Matrix Element"=-3.9870451933563427, "Real Matrix Element"=19.09715847690375}, {"Real Matrix Element"=-4.146516326164448, "Real Matrix Element"=19.04868488433741}, {"Real Matrix Element"=-4.142394023995336, "Real Matrix Element"=19.03682270825432}, {"Real Matrix Element"=-4.214814722130296, "Real Matrix Element"=19.013137239782303}, {"Real Matrix Element"=-4.24471132522973, "Real Matrix Element"=18.947474163246252}, {"Real Matrix Element"=-4.322813185919806, "Real Matrix Element"=18.897879708834168}, {"Real Matrix Element"=-4.432206655147543, "Real Matrix Element"=18.8486091620742}, {"Real Matrix Element"=-4.421487428478846, "Real Matrix Element"=18.905812137680357}, {"Real Matrix Element"=-4.4860338774182, "Real Matrix Element"=18.91141131997031}, {"Real Matrix Element"=-4.594603966173011, "Real Matrix Element"=18.809786834536013}, {"Real Matrix Element"=-4.968686656009144, "Real Matrix Element"=18.58838362199552}, {"Real Matrix Element"=-5.027711044999022, "Real Matrix Element"=18.578285626577944}, {"Real Matrix Element"=-5.088733673058099, "Real Matrix Element"=18.51849250760569}, {"Real Matrix Element"=-5.096104891518352, "Real Matrix Element"=18.442973752543164}, {"Real Matrix Element"=-5.4093429005270055, "Real Matrix Element"=18.279865277856107}, {"Real Matrix Element"=-5.472383180151836, "Real Matrix Element"=18.230591243770405}, {"Real Matrix Element"=-5.414859982941357, "Real Matrix Element"=18.334120954729666}, {"Real Matrix Element"=-5.584072508352708, "Real Matrix Element"=18.330716807521117}, {"Real Matrix Element"=-5.465596746330523, "Real Matrix Element"=18.348124956413603}, {"Real Matrix Element"=-5.701327206147861, "Real Matrix Element"=18.23648719461537}, {"Real Matrix Element"=-5.766341640271329, "Real Matrix Element"=18.187323317380596}, {"Real Matrix Element"=-5.686852328085646, "Real Matrix Element"=18.298067720661884}, {"Real Matrix Element"=-5.923556479513387, "Real Matrix Element"=18.066382097754325}, {"Real Matrix Element"=-5.8842313551207726, "Real Matrix Element"=18.098723778709832}, {"Real Matrix Element"=-6.059247435368079, "Real Matrix Element"=17.961343766192705}, {"Real Matrix Element"=-5.993682612456029, "Real Matrix Element"=17.983396573764338}, {"Real Matrix Element"=-6.144698331606486, "Real Matrix Element"=17.820723742990577}, {"Real Matrix Element"=-6.297244859692786, "Real Matrix Element"=17.676510352584476}, {"Real Matrix Element"=-6.340959847300945, "Real Matrix Element"=17.73213817616045}, {"Real Matrix Element"=-6.606604062745652, "Real Matrix Element"=17.55658561551106}, {"Real Matrix Element"=-6.7942074904535, "Real Matrix Element"=17.426892171245793}, {"Real Matrix Element"=-6.759008904602816, "Real Matrix Element"=17.399228932716127}, {"Real Matrix Element"=-6.841664600199093, "Real Matrix Element"=17.296916632143468}, {"Real Matrix Element"=-6.785519911506022, "Real Matrix Element"=17.289693414802098}, {"Real Matrix Element"=-6.749120263097507, "Real Matrix Element"=17.346148936822537}, {"Real Matrix Element"=-6.811961628247967, "Real Matrix Element"=17.289246152154544}, {"Real Matrix Element"=-6.928297189838397, "Real Matrix Element"=17.165276806403092}, {"Real Matrix Element"=-6.908575023661083, "Real Matrix Element"=17.142897098543024}, {"Real Matrix Element"=-7.019344433659546, "Real Matrix Element"=17.0820835198406}, {"Real Matrix Element"=-7.357788926085682, "Real Matrix Element"=16.764086846281202}, {"Real Matrix Element"=-7.406265509676493, "Real Matrix Element"=16.73154975369563}, {"Real Matrix Element"=-7.42036178822834, "Real Matrix Element"=16.65741249395844}, {"Real Matrix Element"=-7.463528332905717, "Real Matrix Element"=16.658099874947403}, {"Real Matrix Element"=-7.567907578364607, "Real Matrix Element"=16.506950672187422}, {"Real Matrix Element"=-7.615944724660424, "Real Matrix Element"=16.461722576266837}, {"Real Matrix Element"=-7.655873033283315, "Real Matrix Element"=16.46168568570257}, {"Real Matrix Element"=-7.706507733921145, "Real Matrix Element"=16.374776858190454}, {"Real Matrix Element"=-7.846017668164562, "Real Matrix Element"=16.24942167333011}, {"Real Matrix Element"=-7.857757108132345, "Real Matrix Element"=16.053384442969673}, {"Real Matrix Element"=-7.793472375124623, "Real Matrix Element"=16.16291838281126}, {"Real Matrix Element"=-7.890141704683177, "Real Matrix Element"=15.868665529830979}, {"Real Matrix Element"=-7.967212256110334, "Real Matrix Element"=15.699057516895166}, {"Real Matrix Element"=-7.92086145383362, "Real Matrix Element"=15.86302776588854}, {"Real Matrix Element"=-7.942301765689768, "Real Matrix Element"=15.879919464654208}, {"Real Matrix Element"=-7.977646223628317, "Real Matrix Element"=15.790060605481123}, {"Real Matrix Element"=-8.023438154511208, "Real Matrix Element"=15.807372812068248}, {"Real Matrix Element"=-8.115051684221566, "Real Matrix Element"=15.662271974060012}, {"Real Matrix Element"=-8.269820803286382, "Real Matrix Element"=15.475512919530333}, {"Real Matrix Element"=-8.355551727837417, "Real Matrix Element"=15.343053404552153}, {"Real Matrix Element"=-8.49438439276272, "Real Matrix Element"=15.208135697322062}, {"Real Matrix Element"=-8.602189672856285, "Real Matrix Element"=15.018230926744327}, {"Real Matrix Element"=-8.716376252033172, "Real Matrix Element"=15.00739020594311}, {"Real Matrix Element"=-8.620763513870639, "Real Matrix Element"=15.033628865686762}, {"Real Matrix Element"=-8.637524546194022, "Real Matrix Element"=14.772381379379702}, {"Real Matrix Element"=-8.568723682685878, "Real Matrix Element"=14.976378908475509}, {"Real Matrix Element"=-8.722376709392002, "Real Matrix Element"=14.762353889455008}, {"Real Matrix Element"=-8.910952936630698, "Real Matrix Element"=14.5835922811282}, {"Real Matrix Element"=-8.823998813852088, "Real Matrix Element"=14.61738863283166}, {"Real Matrix Element"=-8.822220105094592, "Real Matrix Element"=14.616740930102287}, {"Real Matrix Element"=-8.87195858069016, "Real Matrix Element"=14.57204066667054}, {"Real Matrix Element"=-8.912828920880289, "Real Matrix Element"=14.512877519838884}, {"Real Matrix Element"=-9.20864778064972, "Real Matrix Element"=14.331562401717186}, {"Real Matrix Element"=-9.092432269802018, "Real Matrix Element"=14.329921885073444}, {"Real Matrix Element"=-9.248391158367127, "Real Matrix Element"=14.12730989313166}, {"Real Matrix Element"=-9.276262358266502, "Real Matrix Element"=14.160801162542654}, {"Real Matrix Element"=-9.252389020129378, "Real Matrix Element"=14.178740089642929}, {"Real Matrix Element"=-9.226118300750272, "Real Matrix Element"=14.154894247536582}, {"Real Matrix Element"=-9.303888971677111, "Real Matrix Element"=14.00853409494262}, {"Real Matrix Element"=-9.386395069427573, "Real Matrix Element"=13.784108795073616}, {"Real Matrix Element"=-9.420997473042332, "Real Matrix Element"=13.66921675611135}, {"Real Matrix Element"=-9.487267792236981, "Real Matrix Element"=13.409265034937981}, {"Real Matrix Element"=-9.426812731485544, "Real Matrix Element"=13.57911237454815}, {"Real Matrix Element"=-9.428082334132181, "Real Matrix Element"=13.567926012551544}, {"Real Matrix Element"=-9.544587474726463, "Real Matrix Element"=13.268767837059725}, {"Real Matrix Element"=-9.559522443218484, "Real Matrix Element"=13.128120985084717}, {"Real Matrix Element"=-9.578672975867576, "Real Matrix Element"=12.979444211121665}, {"Real Matrix Element"=-9.555416209360299, "Real Matrix Element"=13.04356302533869}, {"Real Matrix Element"=-9.547963106746732, "Real Matrix Element"=12.955945754280016}, {"Real Matrix Element"=-9.583096415194097, "Real Matrix Element"=12.75616232824049}, {"Real Matrix Element"=-9.579916866973637, "Real Matrix Element"=12.707527595254708}, {"Real Matrix Element"=-9.608406559208314, "Real Matrix Element"=12.499872787471721}, {"Real Matrix Element"=-9.64001267395752, "Real Matrix Element"=12.456625225320984}, {"Real Matrix Element"=-9.61535388955382, "Real Matrix Element"=12.41209904565396}, {"Real Matrix Element"=-9.668040697591632, "Real Matrix Element"=12.292614373588414}, {"Real Matrix Element"=-9.772496925047935, "Real Matrix Element"=12.06376761485773}, {"Real Matrix Element"=-9.73531555033164, "Real Matrix Element"=12.123359018335744}, {"Real Matrix Element"=-9.738084170592497, "Real Matrix Element"=11.890900665760828}, {"Real Matrix Element"=-9.785709765068054, "Real Matrix Element"=11.814942514771744}, {"Real Matrix Element"=-9.825609739372679, "Real Matrix Element"=11.49521807490202}, {"Real Matrix Element"=-9.851746408288774, "Real Matrix Element"=11.417901369954699}, {"Real Matrix Element"=-9.854525605073889, "Real Matrix Element"=11.536184466678085}, {"Real Matrix Element"=-9.901375307310913, "Real Matrix Element"=11.437048008149029}, {"Real Matrix Element"=-9.907881353029758, "Real Matrix Element"=11.35939672213105}, {"Real Matrix Element"=-9.92029963181502, "Real Matrix Element"=11.20996773564769}, {"Real Matrix Element"=-10.064543212297343, "Real Matrix Element"=10.960844305990648}, {"Real Matrix Element"=-10.05601442251815, "Real Matrix Element"=10.945279457405993}, {"Real Matrix Element"=-10.009796626350267, "Real Matrix Element"=11.11458883901818}, {"Real Matrix Element"=-10.106842990914126, "Real Matrix Element"=10.88820489817789}, {"Real Matrix Element"=-10.040561279730307, "Real Matrix Element"=10.961799424778414}, {"Real Matrix Element"=-10.065914911071637, "Real Matrix Element"=10.834339876320692}, {"Real Matrix Element"=-10.163028976250894, "Real Matrix Element"=10.595966477687574}, {"Real Matrix Element"=-10.171350257377215, "Real Matrix Element"=10.521423653431839}, {"Real Matrix Element"=-10.063241245359919, "Real Matrix Element"=10.76474902103273}, {"Real Matrix Element"=-10.10342977530472, "Real Matrix Element"=10.66995506693628}, {"Real Matrix Element"=-10.15088861411603, "Real Matrix Element"=10.476295586433572}, {"Real Matrix Element"=-10.19634363117352, "Real Matrix Element"=10.300026901497098}, {"Real Matrix Element"=-10.245515736074061, "Real Matrix Element"=10.062642775400539}, {"Real Matrix Element"=-10.24099434901633, "Real Matrix Element"=10.001612388527732}, {"Real Matrix Element"=-10.229526360773452, "Real Matrix Element"=9.944443246724262}, {"Real Matrix Element"=-10.221015835247153, "Real Matrix Element"=9.948472345309144}, {"Real Matrix Element"=-10.177288019337087, "Real Matrix Element"=9.735978699469804}, {"Real Matrix Element"=-10.09378496562067, "Real Matrix Element"=9.51418936298621}, {"Real Matrix Element"=-9.912698493778258, "Real Matrix Element"=9.124660067418862}, {"Real Matrix Element"=-9.877025436809928, "Real Matrix Element"=8.955048726352448}, {"Real Matrix Element"=-9.902731609497973, "Real Matrix Element"=9.045638795804251}, {"Real Matrix Element"=-9.804168898876219, "Real Matrix Element"=8.74338078626154}, {"Real Matrix Element"=-9.808454080925841, "Real Matrix Element"=8.776619287289762}, {"Real Matrix Element"=-9.831972968103395, "Real Matrix Element"=8.700355640865322}, {"Real Matrix Element"=-9.756571127396317, "Real Matrix Element"=8.362702240680571}, {"Real Matrix Element"=-9.822783532612966, "Real Matrix Element"=8.707696286251954}, {"Real Matrix Element"=-9.744598282293623, "Real Matrix Element"=8.192726675953173}, {"Real Matrix Element"=-9.708924429323323, "Real Matrix Element"=8.138923284645564}, {"Real Matrix Element"=-9.64025129895936, "Real Matrix Element"=8.092015004838188}, {"Real Matrix Element"=-9.692419722112652, "Real Matrix Element"=8.153343956110767}, {"Real Matrix Element"=-9.722570840299767, "Real Matrix Element"=8.198873329578195}, {"Real Matrix Element"=-9.743331016135281, "Real Matrix Element"=7.955066778404824}, {"Real Matrix Element"=-9.712989527810642, "Real Matrix Element"=7.927891641441574}, {"Real Matrix Element"=-9.682161137718643, "Real Matrix Element"=7.703739279870044}, {"Real Matrix Element"=-9.674693764543159, "Real Matrix Element"=7.686237823640707}, {"Real Matrix Element"=-9.693802312825659, "Real Matrix Element"=7.796653678097531}, {"Real Matrix Element"=-9.734690412270906, "Real Matrix Element"=7.567973272882505}, {"Real Matrix Element"=-9.629452807163323, "Real Matrix Element"=7.553531784966619}, {"Real Matrix Element"=-9.609587028132795, "Real Matrix Element"=7.519548402691971}, {"Real Matrix Element"=-9.276231004900149, "Real Matrix Element"=6.872379883721609}, {"Real Matrix Element"=-9.411931109634446, "Real Matrix Element"=7.151810064000592}, {"Real Matrix Element"=-9.348194772929999, "Real Matrix Element"=6.8591748082688575}, {"Real Matrix Element"=-9.409801031258192, "Real Matrix Element"=6.911569434980947}, {"Real Matrix Element"=-9.406810421406261, "Real Matrix Element"=6.816605960094776}, {"Real Matrix Element"=-9.456184038380275, "Real Matrix Element"=6.952440558415744}, {"Real Matrix Element"=-9.440085164284564, "Real Matrix Element"=6.766597504950259}, {"Real Matrix Element"=-9.445133343036812, "Real Matrix Element"=6.753193879676117}, {"Real Matrix Element"=-9.51320991737569, "Real Matrix Element"=6.917126220938826}, {"Real Matrix Element"=-9.398463481568234, "Real Matrix Element"=6.416441496388521}, {"Real Matrix Element"=-9.437763550908132, "Real Matrix Element"=6.204897939815499}, {"Real Matrix Element"=-9.38368190188581, "Real Matrix Element"=6.215565262989236}, {"Real Matrix Element"=-9.325602222844472, "Real Matrix Element"=6.16743073510507}, {"Real Matrix Element"=-9.266341331864329, "Real Matrix Element"=5.978192308567106}, {"Real Matrix Element"=-9.237920067552366, "Real Matrix Element"=5.942689928834683}, {"Real Matrix Element"=-9.060857859757085, "Real Matrix Element"=5.791765238798215}, {"Real Matrix Element"=-9.125677723368645, "Real Matrix Element"=5.828996251383734}, {"Real Matrix Element"=-9.06867982230412, "Real Matrix Element"=5.729502317563743}, {"Real Matrix Element"=-8.96068987516246, "Real Matrix Element"=5.57466363031194}, {"Real Matrix Element"=-8.882962106253274, "Real Matrix Element"=5.540072312383251}, {"Real Matrix Element"=-8.780364646381953, "Real Matrix Element"=5.535321943171675}, {"Real Matrix Element"=-8.658415907496126, "Real Matrix Element"=5.313962185168001}, {"Real Matrix Element"=-8.658834782684727, "Real Matrix Element"=5.275039761629756}, {"Real Matrix Element"=-8.603003983110419, "Real Matrix Element"=5.144634153050872}, {"Real Matrix Element"=-8.59455066894399, "Real Matrix Element"=5.110085006799983}, {"Real Matrix Element"=-8.626261365830857, "Real Matrix Element"=5.136349578515332}, {"Real Matrix Element"=-8.521110681536602, "Real Matrix Element"=4.931491253002303}, {"Real Matrix Element"=-8.494370305774478, "Real Matrix Element"=4.864118065144198}, {"Real Matrix Element"=-8.431633616316077, "Real Matrix Element"=4.73170307326922}, {"Real Matrix Element"=-8.381460580944005, "Real Matrix Element"=4.661493776390952}, {"Real Matrix Element"=-8.186402991018545, "Real Matrix Element"=4.567437898438884}, {"Real Matrix Element"=-8.189034293008406, "Real Matrix Element"=4.496072164338133}, {"Real Matrix Element"=-8.19071674279047, "Real Matrix Element"=4.470416846014742}, {"Real Matrix Element"=-8.102230746038751, "Real Matrix Element"=4.369220599761081}, {"Real Matrix Element"=-8.141737652845155, "Real Matrix Element"=4.299961787934484}, {"Real Matrix Element"=-8.175059009123189, "Real Matrix Element"=4.329630995656957}, {"Real Matrix Element"=-8.085567945416054, "Real Matrix Element"=4.290145377508109}, {"Real Matrix Element"=-7.960641069437882, "Real Matrix Element"=4.062451637064886}, {"Real Matrix Element"=-7.842042202188181, "Real Matrix Element"=3.8598022401168284}, {"Real Matrix Element"=-7.789335245927225, "Real Matrix Element"=3.8381413733236034}, {"Real Matrix Element"=-7.593490064630421, "Real Matrix Element"=3.6973253436184943}, {"Real Matrix Element"=-7.528315565212855, "Real Matrix Element"=3.655284359434639}, {"Real Matrix Element"=-7.486990683149448, "Real Matrix Element"=3.6150999672796895}, {"Real Matrix Element"=-7.420118471369763, "Real Matrix Element"=3.518524953566094}, {"Real Matrix Element"=-7.465296334003506, "Real Matrix Element"=3.5585533486944403}, {"Real Matrix Element"=-7.378367946624692, "Real Matrix Element"=3.441061685376617}, {"Real Matrix Element"=-7.357203888149772, "Real Matrix Element"=3.391026393091389}, {"Real Matrix Element"=-7.233527374980325, "Real Matrix Element"=3.187349948351454}, {"Real Matrix Element"=-7.2934578007710185, "Real Matrix Element"=3.2900948143453284}, {"Real Matrix Element"=-7.238248638165405, "Real Matrix Element"=3.139831833619214}, {"Real Matrix Element"=-7.123675150698881, "Real Matrix Element"=3.1301575964934303}, {"Real Matrix Element"=-6.97107387344392, "Real Matrix Element"=2.968451766996001}, {"Real Matrix Element"=-6.920132460701653, "Real Matrix Element"=2.7945957989560375}, {"Real Matrix Element"=-6.79612037310448, "Real Matrix Element"=2.649215065966586}, {"Real Matrix Element"=-6.527166313579803, "Real Matrix Element"=2.6179666793089162}, {"Real Matrix Element"=-6.649180959111971, "Real Matrix Element"=2.596684547747543}, {"Real Matrix Element"=-6.5225501157870855, "Real Matrix Element"=2.5069517869365665}, {"Real Matrix Element"=-6.566844410116811, "Real Matrix Element"=2.566326498563466}, {"Real Matrix Element"=-6.33006119060101, "Real Matrix Element"=2.3294640381318903}, {"Real Matrix Element"=-6.38191669328145, "Real Matrix Element"=2.358678993240383}, {"Real Matrix Element"=-6.248921442848741, "Real Matrix Element"=2.174726541098687}, {"Real Matrix Element"=-6.324625444317432, "Real Matrix Element"=2.2242034478183577}, {"Real Matrix Element"=-6.238498496408809, "Real Matrix Element"=2.164460722606962}, {"Real Matrix Element"=-6.091793603859644, "Real Matrix Element"=2.069784914330779}, {"Real Matrix Element"=-6.048144495468988, "Real Matrix Element"=2.0566528302934652}, {"Real Matrix Element"=-5.958351043265749, "Real Matrix Element"=1.9829064275365818}, {"Real Matrix Element"=-5.724002953783958, "Real Matrix Element"=1.9219731938907576}, {"Real Matrix Element"=-5.84615420015502, "Real Matrix Element"=1.9352016429850862}, {"Real Matrix Element"=-5.815785703628918, "Real Matrix Element"=1.9106989440701454}, {"Real Matrix Element"=-5.570845936636707, "Real Matrix Element"=1.8027935283293777}, {"Real Matrix Element"=-5.463498209245966, "Real Matrix Element"=1.7092365473596904}, {"Real Matrix Element"=-5.4731422794090925, "Real Matrix Element"=1.743231668035098}, {"Real Matrix Element"=-5.372080287068641, "Real Matrix Element"=1.745450176038625}, {"Real Matrix Element"=-5.01389502782636, "Real Matrix Element"=1.496431270007249}, {"Real Matrix Element"=-5.06080419761598, "Real Matrix Element"=1.5911242814611044}, {"Real Matrix Element"=-5.021070014300207, "Real Matrix Element"=1.5310759244350995}, {"Real Matrix Element"=-4.942972193858035, "Real Matrix Element"=1.453639382280097}, {"Real Matrix Element"=-4.859914765079465, "Real Matrix Element"=1.439505557821833}, {"Real Matrix Element"=-4.790602110515505, "Real Matrix Element"=1.3779596782259353}, {"Real Matrix Element"=-4.793789817518051, "Real Matrix Element"=1.3697114399815205}, {"Real Matrix Element"=-4.392568404457909, "Real Matrix Element"=1.2000477366761009}, {"Real Matrix Element"=-4.3698457302399145, "Real Matrix Element"=1.1110650038602767}, {"Real Matrix Element"=-4.519975483842312, "Real Matrix Element"=1.1781035038542862}, {"Real Matrix Element"=-4.380274471902355, "Real Matrix Element"=1.1274551763056502}, {"Real Matrix Element"=-4.403941970787262, "Real Matrix Element"=1.1495151197080884}, {"Real Matrix Element"=-4.141625380141059, "Real Matrix Element"=0.9926810459331082}, {"Real Matrix Element"=-4.024739838950894, "Real Matrix Element"=0.8937429661043096}, {"Real Matrix Element"=-3.9101292896576503, "Real Matrix Element"=0.8459435684361913}, {"Real Matrix Element"=-3.80694786350699, "Real Matrix Element"=0.79234712436912}, {"Real Matrix Element"=-4.019863830788703, "Real Matrix Element"=0.9002611834889935}, {"Real Matrix Element"=-3.823863198232145, "Real Matrix Element"=0.8156092728022238}, {"Real Matrix Element"=-3.698779264145462, "Real Matrix Element"=0.7238919592953792}, {"Real Matrix Element"=-3.517450014412432, "Real Matrix Element"=0.6385666823484833}, {"Real Matrix Element"=-3.5586264900036544, "Real Matrix Element"=0.6626703539532454}, {"Real Matrix Element"=-3.3345898181153406, "Real Matrix Element"=0.551138140447731}, {"Real Matrix Element"=-3.425743530563711, "Real Matrix Element"=0.5245120477203156}, {"Real Matrix Element"=-3.171683147014441, "Real Matrix Element"=0.5062813889334657}, {"Real Matrix Element"=-2.8890899089625504, "Real Matrix Element"=0.47684778544709006}, {"Real Matrix Element"=-2.9002833962072754, "Real Matrix Element"=0.5361578024440675}, {"Real Matrix Element"=-2.865750956412222, "Real Matrix Element"=0.5257245027746684}, {"Real Matrix Element"=-2.8415555836523096, "Real Matrix Element"=0.5567428267662712}, {"Real Matrix Element"=-2.740665326422215, "Real Matrix Element"=0.5325231586599319}, {"Real Matrix Element"=-2.742930456970592, "Real Matrix Element"=0.5329131399992207}, {"Real Matrix Element"=-2.3972703143805028, "Real Matrix Element"=0.3942380806301396}, {"Real Matrix Element"=-2.4104122472263665, "Real Matrix Element"=0.41913499395971465}, {"Real Matrix Element"=-2.174302932778657, "Real Matrix Element"=0.3250924816024241}, {"Real Matrix Element"=-2.1003478404897304, "Real Matrix Element"=0.22513344568560986}, {"Real Matrix Element"=-2.1774442969573893, "Real Matrix Element"=0.2674315109377016}, {"Real Matrix Element"=-2.217989662606111, "Real Matrix Element"=0.26869292938644196}, {"Real Matrix Element"=-2.032410934369105, "Real Matrix Element"=0.2552486981923703}, {"Real Matrix Element"=-1.8482653920402803, "Real Matrix Element"=0.2476866224332171}, {"Real Matrix Element"=-1.8958374263854199, "Real Matrix Element"=0.2933057378847507}, {"Real Matrix Element"=-1.7892378306316234, "Real Matrix Element"=0.29678627086779097}, {"Real Matrix Element"=-1.685058802006406, "Real Matrix Element"=0.29215469483710105}, {"Real Matrix Element"=-1.5554563768944247, "Real Matrix Element"=0.2488237087955089}, {"Real Matrix Element"=-1.192361377134566, "Real Matrix Element"=0.2656527418444694}, {"Real Matrix Element"=-1.000599203084601, "Real Matrix Element"=-0.05934301434072994}, {"Real Matrix Element"=-1.1536011581524936, "Real Matrix Element"=0.039615412917648175}, {"Real Matrix Element"=-0.7419632791639659, "Real Matrix Element"=0.12147721373925341}, {"Real Matrix Element"=-0.8340110569815569, "Real Matrix Element"=0.1969576251952177}, {"Real Matrix Element"=-1.027898367305768, "Real Matrix Element"=0.2029727456473001}, {"Real Matrix Element"=-0.6500314227191863, "Real Matrix Element"=-0.03306266662094916}, {"Real Matrix Element"=-0.7530664765759607, "Real Matrix Element"=0.06349808799296484}, {"Real Matrix Element"=-0.6773312680683672, "Real Matrix Element"=-0.02585629968287406}, {"Real Matrix Element"=-0.5956514518130793, "Real Matrix Element"=-0.048447442407375224}, {"Real Matrix Element"=-0.4049314479269736, "Real Matrix Element"=-0.11496537064166594}, {"Real Matrix Element"=-0.16267304849708267, "Real Matrix Element"=-0.16748855273923496}, {"Real Matrix Element"=-0.24085198302405209, "Real Matrix Element"=-0.17293359666842767}, {"Real Matrix Element"=-0.0391792194748969, "Real Matrix Element"=-0.1619398622894085}, {"Real Matrix Element"=-0.007849954227983109, "Real Matrix Element"=-0.10067800935234084}, {"Real Matrix Element"=0.09337275193410202, "Real Matrix Element"=-0.10376959991882143}, {"Real Matrix Element"=0.2357566091917929, "Real Matrix Element"=-0.09335570294023252}, {"Real Matrix Element"=0.2923751734109657, "Real Matrix Element"=-0.09532366297820115}, {"Real Matrix Element"=0.23869009773238797, "Real Matrix Element"=-0.0910201490885043}, {"Real Matrix Element"=0.45860650677328313, "Real Matrix Element"=0.0451635634144893}, {"Real Matrix Element"=0.5167389626106872, "Real Matrix Element"=0.05456517737912229}, {"Real Matrix Element"=0.7445343124253421, "Real Matrix Element"=0.051117804477761264}, {"Real Matrix Element"=0.7302042906817997, "Real Matrix Element"=0.08144405672133272}, {"Real Matrix Element"=0.7962630453647265, "Real Matrix Element"=0.07991379030794636}, {"Real Matrix Element"=0.9204911546955988, "Real Matrix Element"=0.09509155082009046}, {"Real Matrix Element"=1.0991292732426006, "Real Matrix Element"=0.1309645907226577}, {"Real Matrix Element"=1.2585769495873678, "Real Matrix Element"=0.1919215631955834}, {"Real Matrix Element"=1.2393018053750844, "Real Matrix Element"=0.1869477188145354}, {"Real Matrix Element"=1.4613173477205736, "Real Matrix Element"=0.2285125407653715}, {"Real Matrix Element"=1.5005324954649555, "Real Matrix Element"=0.24906811112565563}, {"Real Matrix Element"=1.5802152529235542, "Real Matrix Element"=0.22981366950312926}, {"Real Matrix Element"=1.675042802431092, "Real Matrix Element"=0.24575664277323903}, {"Real Matrix Element"=1.943943516882229, "Real Matrix Element"=0.1367891598852499}, {"Real Matrix Element"=1.8644628762884323, "Real Matrix Element"=0.11178832925114736}, {"Real Matrix Element"=2.084207290727597, "Real Matrix Element"=0.17377650204375522}, {"Real Matrix Element"=2.125452821054328, "Real Matrix Element"=0.1693199354539219}, {"Real Matrix Element"=2.1125451840897775, "Real Matrix Element"=0.14770348264746797}, {"Real Matrix Element"=2.28023706285353, "Real Matrix Element"=0.2962287029612582}, {"Real Matrix Element"=2.4505851631986983, "Real Matrix Element"=0.3190398289513382}, {"Real Matrix Element"=2.3684218612105994, "Real Matrix Element"=0.4196693893194462}, {"Real Matrix Element"=2.8932325619735186, "Real Matrix Element"=0.5634119554183398}, {"Real Matrix Element"=2.566507412010397, "Real Matrix Element"=0.42872988095369363}, {"Real Matrix Element"=2.8307405105698114, "Real Matrix Element"=0.4895099660869246}, {"Real Matrix Element"=3.0449238001310213, "Real Matrix Element"=0.49097933166667695}, {"Real Matrix Element"=3.076697899495772, "Real Matrix Element"=0.46132264360117575}, {"Real Matrix Element"=3.2713771131753067, "Real Matrix Element"=0.4676710880329487}, {"Real Matrix Element"=3.282387588769298, "Real Matrix Element"=0.4484950614712362}, {"Real Matrix Element"=3.3303030205730133, "Real Matrix Element"=0.517914844958116}, {"Real Matrix Element"=3.4574146080557226, "Real Matrix Element"=0.5760596688122895}, {"Real Matrix Element"=3.4139829615258113, "Real Matrix Element"=0.5991720602415525}, {"Real Matrix Element"=3.6989093758229004, "Real Matrix Element"=0.7000471242778273}, {"Real Matrix Element"=3.8617296325127586, "Real Matrix Element"=0.6027750251924466}, {"Real Matrix Element"=3.7709960796693087, "Real Matrix Element"=0.6181807503517146}, {"Real Matrix Element"=3.941831877692702, "Real Matrix Element"=0.6610868359137454}, {"Real Matrix Element"=3.886076529377795, "Real Matrix Element"=0.6424025862282078}, {"Real Matrix Element"=4.103122071088338, "Real Matrix Element"=0.7757695267703894}, {"Real Matrix Element"=4.229778370299839, "Real Matrix Element"=0.8941841243898413}, {"Real Matrix Element"=4.124883813093223, "Real Matrix Element"=0.8862270671025756}, {"Real Matrix Element"=4.163637621181438, "Real Matrix Element"=0.9072989522199845}, {"Real Matrix Element"=4.288139591494989, "Real Matrix Element"=0.9742695749617105}, {"Real Matrix Element"=4.261108934109162, "Real Matrix Element"=0.9298270735984686}, {"Real Matrix Element"=4.535275826366214, "Real Matrix Element"=1.1266082518763387}, {"Real Matrix Element"=4.480009280719288, "Real Matrix Element"=1.0924595658018554}, {"Real Matrix Element"=4.578432475184731, "Real Matrix Element"=1.1723805582831528}, {"Real Matrix Element"=4.7683655941810095, "Real Matrix Element"=1.3154914137005984}, {"Real Matrix Element"=4.796507774636926, "Real Matrix Element"=1.352509310326659}, {"Real Matrix Element"=4.900878607938295, "Real Matrix Element"=1.4271732300787716}, {"Real Matrix Element"=4.939846964336004, "Real Matrix Element"=1.4188491625680464}, {"Real Matrix Element"=5.185280506138785, "Real Matrix Element"=1.4853457048720398}, {"Real Matrix Element"=5.119019264689455, "Real Matrix Element"=1.4266916457141745}, {"Real Matrix Element"=5.240316194321512, "Real Matrix Element"=1.4744890496861103}, {"Real Matrix Element"=5.185460334925421, "Real Matrix Element"=1.4327579376302846}, {"Real Matrix Element"=5.572487518785223, "Real Matrix Element"=1.6190743110768056}, {"Real Matrix Element"=5.699237352922708, "Real Matrix Element"=1.6581137768102194}, {"Real Matrix Element"=5.866002924177275, "Real Matrix Element"=1.7609424028523646}, {"Real Matrix Element"=5.8776411008785745, "Real Matrix Element"=1.8149893898837124}, {"Real Matrix Element"=6.083847859881567, "Real Matrix Element"=1.9206831251944687}, {"Real Matrix Element"=6.173711422305054, "Real Matrix Element"=1.9796753952823047}, {"Real Matrix Element"=6.087510626856309, "Real Matrix Element"=1.954184648997332}, {"Real Matrix Element"=6.032009741824098, "Real Matrix Element"=1.9240945899491004}, {"Real Matrix Element"=6.023081196558264, "Real Matrix Element"=1.9290265243410705}, {"Real Matrix Element"=6.229634926602499, "Real Matrix Element"=2.0851734555721024}, {"Real Matrix Element"=6.227714460075391, "Real Matrix Element"=2.0646541781595698}, {"Real Matrix Element"=6.384841047817527, "Real Matrix Element"=2.168423906127086}, {"Real Matrix Element"=6.516909843016781, "Real Matrix Element"=2.3008215543033845}, {"Real Matrix Element"=6.6398087592706165, "Real Matrix Element"=2.5329097146897688}, {"Real Matrix Element"=6.777523765741138, "Real Matrix Element"=2.587130318293964}, {"Real Matrix Element"=6.455977125395683, "Real Matrix Element"=2.4560829670355564}, {"Real Matrix Element"=6.688365959041406, "Real Matrix Element"=2.6058301428700603}, {"Real Matrix Element"=6.882183195792442, "Real Matrix Element"=2.7476840050839453}, {"Real Matrix Element"=6.8781759495388775, "Real Matrix Element"=2.6900768674355144}, {"Real Matrix Element"=7.126557706130636, "Real Matrix Element"=2.918319018772779}, {"Real Matrix Element"=7.214973843654836, "Real Matrix Element"=3.0202086308410476}, {"Real Matrix Element"=7.194403497613271, "Real Matrix Element"=2.9735667274685107}, {"Real Matrix Element"=7.2267363246394885, "Real Matrix Element"=3.0516746666797947}, {"Real Matrix Element"=7.256491660151073, "Real Matrix Element"=3.09411420466817}, {"Real Matrix Element"=7.371439149319787, "Real Matrix Element"=3.1877657672169986}, {"Real Matrix Element"=7.392138079885269, "Real Matrix Element"=3.1927038469283966}, {"Real Matrix Element"=7.292607108185961, "Real Matrix Element"=3.101612909346431}, {"Real Matrix Element"=7.604478717420238, "Real Matrix Element"=3.306776249449587}, {"Real Matrix Element"=7.812879599242161, "Real Matrix Element"=3.4666888041457384}, {"Real Matrix Element"=7.822805558473037, "Real Matrix Element"=3.50066029190377}, {"Real Matrix Element"=7.9715052191916715, "Real Matrix Element"=3.5422719443842654}, {"Real Matrix Element"=8.005009348965084, "Real Matrix Element"=3.5541315617342013}, {"Real Matrix Element"=8.105938322510795, "Real Matrix Element"=3.791591415882158}, {"Real Matrix Element"=7.990203759119015, "Real Matrix Element"=3.6824762257987995}, {"Real Matrix Element"=8.04529413010032, "Real Matrix Element"=3.7336563813063375}, {"Real Matrix Element"=8.134487610984282, "Real Matrix Element"=3.829726541353045}, {"Real Matrix Element"=8.048311155727323, "Real Matrix Element"=3.8280949674010705}, {"Real Matrix Element"=8.280071852152016, "Real Matrix Element"=4.245729437830963}, {"Real Matrix Element"=8.348907375076854, "Real Matrix Element"=4.338003717511133}, {"Real Matrix Element"=8.325201510898596, "Real Matrix Element"=4.376190153173533}, {"Real Matrix Element"=8.33508541826863, "Real Matrix Element"=4.446366854782025}, {"Real Matrix Element"=8.417605976673599, "Real Matrix Element"=4.628243342405137}, {"Real Matrix Element"=8.54838497245888, "Real Matrix Element"=4.763884130640754}, {"Real Matrix Element"=8.53641073103145, "Real Matrix Element"=4.78773793590799}, {"Real Matrix Element"=8.52582801495695, "Real Matrix Element"=4.704153590857627}, {"Real Matrix Element"=8.639207434754635, "Real Matrix Element"=4.871439509103279}, {"Real Matrix Element"=8.574104601202514, "Real Matrix Element"=4.766634503390851}, {"Real Matrix Element"=8.682322787046576, "Real Matrix Element"=4.927609466421556}, {"Real Matrix Element"=8.78641901048453, "Real Matrix Element"=5.166548360356944}, {"Real Matrix Element"=8.757246551807047, "Real Matrix Element"=5.246000976221646}, {"Real Matrix Element"=8.79297328475289, "Real Matrix Element"=5.226824527233645}, {"Real Matrix Element"=8.874420789709083, "Real Matrix Element"=5.4904154197870865}, {"Real Matrix Element"=8.925783595335218, "Real Matrix Element"=5.388965143604032}, {"Real Matrix Element"=8.954105857499234, "Real Matrix Element"=5.536717675856532}, {"Real Matrix Element"=9.02678902185365, "Real Matrix Element"=5.610587571021968}, {"Real Matrix Element"=9.010807902329242, "Real Matrix Element"=5.657731859291321}, {"Real Matrix Element"=9.098476529932622, "Real Matrix Element"=5.878581680664117}, {"Real Matrix Element"=9.097508663634974, "Real Matrix Element"=5.93805904457568}, {"Real Matrix Element"=9.126344133170123, "Real Matrix Element"=6.039849559128261}, {"Real Matrix Element"=9.101370060423228, "Real Matrix Element"=6.0278048117140575}, {"Real Matrix Element"=9.133889639696681, "Real Matrix Element"=6.030342801488644}, {"Real Matrix Element"=9.145643237931777, "Real Matrix Element"=6.355311943462956}, {"Real Matrix Element"=9.212387164760417, "Real Matrix Element"=6.444865005827915}, {"Real Matrix Element"=9.247157106898142, "Real Matrix Element"=6.4776351891757455}, {"Real Matrix Element"=9.279822685707591, "Real Matrix Element"=6.548454296513395}, {"Real Matrix Element"=9.338984421594082, "Real Matrix Element"=6.611657442586804}, {"Real Matrix Element"=9.333559042128318, "Real Matrix Element"=6.627523687451309}, {"Real Matrix Element"=9.492017412285715, "Real Matrix Element"=6.81536030758438}, {"Real Matrix Element"=9.618663272297873, "Real Matrix Element"=6.9628446044238315}, {"Real Matrix Element"=9.687197442638656, "Real Matrix Element"=7.025962028978325}, {"Real Matrix Element"=9.820169601837344, "Real Matrix Element"=7.166971320943348}, {"Real Matrix Element"=9.804166090501964, "Real Matrix Element"=7.153930318142333}, {"Real Matrix Element"=9.774811939998743, "Real Matrix Element"=7.404171935773015}, {"Real Matrix Element"=9.730157379739465, "Real Matrix Element"=7.2682359488715935}, {"Real Matrix Element"=9.896562091538858, "Real Matrix Element"=7.568296064252648}, {"Real Matrix Element"=9.871569230405642, "Real Matrix Element"=7.481249094801417}, {"Real Matrix Element"=9.971254446313717, "Real Matrix Element"=7.758216409184326}, {"Real Matrix Element"=9.942286482735936, "Real Matrix Element"=7.88376806384654}, {"Real Matrix Element"=9.945733242683938, "Real Matrix Element"=7.891806980468231}, {"Real Matrix Element"=9.960704279660613, "Real Matrix Element"=7.891191825530252}, {"Real Matrix Element"=10.066894298486769, "Real Matrix Element"=8.173846340355464}, {"Real Matrix Element"=10.070118304860056, "Real Matrix Element"=8.473415731738525}, {"Real Matrix Element"=10.054613936231954, "Real Matrix Element"=8.483370665880699}, {"Real Matrix Element"=9.986157544035715, "Real Matrix Element"=8.348802413540678}, {"Real Matrix Element"=9.980216350573365, "Real Matrix Element"=8.506351120766364}, {"Real Matrix Element"=9.9568643994038, "Real Matrix Element"=8.685423276241325}, {"Real Matrix Element"=9.984555949783676, "Real Matrix Element"=8.81322932222992}, {"Real Matrix Element"=10.00239403166861, "Real Matrix Element"=8.788144787206539}, {"Real Matrix Element"=9.92320448208154, "Real Matrix Element"=8.91319765187153}, {"Real Matrix Element"=10.009743772932831, "Real Matrix Element"=9.10256189086073}, {"Real Matrix Element"=9.98311828740161, "Real Matrix Element"=9.156377086221084}, {"Real Matrix Element"=9.983112713875705, "Real Matrix Element"=9.226120075406847}, {"Real Matrix Element"=9.86178069358069, "Real Matrix Element"=9.505313833944804}, {"Real Matrix Element"=9.93970251651499, "Real Matrix Element"=9.351260049027905}, {"Real Matrix Element"=9.978090983506299, "Real Matrix Element"=9.225339317895846}, {"Real Matrix Element"=9.871093734641432, "Real Matrix Element"=9.50876025688642}, {"Real Matrix Element"=9.950888250661134, "Real Matrix Element"=9.358758565119103}, {"Real Matrix Element"=9.790386393757391, "Real Matrix Element"=9.704948083615985}, {"Real Matrix Element"=9.725589239823647, "Real Matrix Element"=9.945984647107357}, {"Real Matrix Element"=9.767041823260309, "Real Matrix Element"=9.927635702496543}, {"Real Matrix Element"=9.80578800947246, "Real Matrix Element"=9.899409951117805}, {"Real Matrix Element"=9.75868838363499, "Real Matrix Element"=10.001939504817349}, {"Real Matrix Element"=9.64526268254352, "Real Matrix Element"=10.2222787719925}, {"Real Matrix Element"=9.759977245644754, "Real Matrix Element"=10.101820254586457}, {"Real Matrix Element"=9.790666017789436, "Real Matrix Element"=10.086194621952076}, {"Real Matrix Element"=9.727708133088605, "Real Matrix Element"=10.165842222352412}, {"Real Matrix Element"=9.623141680989468, "Real Matrix Element"=10.318043623738982}, {"Real Matrix Element"=9.534423632249206, "Real Matrix Element"=10.584864462877528}, {"Real Matrix Element"=9.539749658174577, "Real Matrix Element"=10.708373545287317}, {"Real Matrix Element"=9.597689988347776, "Real Matrix Element"=10.695788627732199}, {"Real Matrix Element"=9.5988371161813, "Real Matrix Element"=10.731888831551561}, {"Real Matrix Element"=9.585819124115565, "Real Matrix Element"=10.857740783384353}, {"Real Matrix Element"=9.597156782082148, "Real Matrix Element"=11.059844929703868}, {"Real Matrix Element"=9.60213723741855, "Real Matrix Element"=11.167434103610487}, {"Real Matrix Element"=9.623986904884497, "Real Matrix Element"=11.297865733269667}, {"Real Matrix Element"=9.674424858200355, "Real Matrix Element"=11.548136284278257}, {"Real Matrix Element"=9.744567105793374, "Real Matrix Element"=11.90523694660968}, {"Real Matrix Element"=9.77783258331913, "Real Matrix Element"=11.997656531971419}, {"Real Matrix Element"=9.777188935409294, "Real Matrix Element"=11.926210501495802}, {"Real Matrix Element"=9.753280133435608, "Real Matrix Element"=11.686326642693231}, {"Real Matrix Element"=9.786091591389111, "Real Matrix Element"=12.005219406189912}, {"Real Matrix Element"=9.77902782232204, "Real Matrix Element"=11.841442130719564}, {"Real Matrix Element"=9.724936186416093, "Real Matrix Element"=12.13300153739661}, {"Real Matrix Element"=9.762396697675445, "Real Matrix Element"=12.188640835565948}, {"Real Matrix Element"=9.822827399601996, "Real Matrix Element"=12.489131228809114}, {"Real Matrix Element"=9.759184114580169, "Real Matrix Element"=12.595852344973043}, {"Real Matrix Element"=9.722203959282606, "Real Matrix Element"=12.804587795833726}, {"Real Matrix Element"=9.698674747005738, "Real Matrix Element"=12.5161881599458}, {"Real Matrix Element"=9.684379476353605, "Real Matrix Element"=12.756615413038432}, {"Real Matrix Element"=9.621588069943035, "Real Matrix Element"=13.004383834395963}, {"Real Matrix Element"=9.575898782096612, "Real Matrix Element"=13.285161743756902}, {"Real Matrix Element"=9.54688739728672, "Real Matrix Element"=13.19417009646656}, {"Real Matrix Element"=9.565435775342966, "Real Matrix Element"=13.248623556726422}, {"Real Matrix Element"=9.484260167770564, "Real Matrix Element"=13.471141290464095}, {"Real Matrix Element"=9.494667248860463, "Real Matrix Element"=13.378264573025685}, {"Real Matrix Element"=9.39855832107206, "Real Matrix Element"=13.69479969886697}, {"Real Matrix Element"=9.371182634352877, "Real Matrix Element"=13.702038677890556}, {"Real Matrix Element"=9.366381224621785, "Real Matrix Element"=13.75045910915255}, {"Real Matrix Element"=9.390465299676833, "Real Matrix Element"=13.74368186337792}, {"Real Matrix Element"=9.342774537430317, "Real Matrix Element"=13.809426359127725}, {"Real Matrix Element"=9.37254299389718, "Real Matrix Element"=13.87301394484324}, {"Real Matrix Element"=9.297869288641287, "Real Matrix Element"=14.237721109699857}, {"Real Matrix Element"=9.201424809617755, "Real Matrix Element"=14.18648278041527}, {"Real Matrix Element"=9.201074797413327, "Real Matrix Element"=14.246807364116641}, {"Real Matrix Element"=9.151464201572605, "Real Matrix Element"=14.249106652103988}, {"Real Matrix Element"=9.112105238549569, "Real Matrix Element"=14.463514306092419}, {"Real Matrix Element"=9.035545194265813, "Real Matrix Element"=14.71070877713427}, {"Real Matrix Element"=9.038469881690176, "Real Matrix Element"=14.694426072357462}, {"Real Matrix Element"=9.019628530353742, "Real Matrix Element"=14.89839574172634}, {"Real Matrix Element"=8.948348092964471, "Real Matrix Element"=14.880251228796297}, {"Real Matrix Element"=8.822371286261008, "Real Matrix Element"=15.10368869935435}, {"Real Matrix Element"=8.850886715016895, "Real Matrix Element"=14.994280017567565}, {"Real Matrix Element"=8.775175307724055, "Real Matrix Element"=15.11929218753579}, {"Real Matrix Element"=8.618969450565965, "Real Matrix Element"=15.411797480662361}, {"Real Matrix Element"=8.611532220972599, "Real Matrix Element"=15.356084808237886}, {"Real Matrix Element"=8.59002226770729, "Real Matrix Element"=15.307026848922934}, {"Real Matrix Element"=8.521845214018851, "Real Matrix Element"=15.390856133828992}, {"Real Matrix Element"=8.417412467500524, "Real Matrix Element"=15.521099499544684}, {"Real Matrix Element"=8.364553136863503, "Real Matrix Element"=15.607554096476465}, {"Real Matrix Element"=8.129240800927526, "Real Matrix Element"=15.854473117236001}, {"Real Matrix Element"=8.266981315682091, "Real Matrix Element"=15.637443866454515}, {"Real Matrix Element"=8.169223410656427, "Real Matrix Element"=15.744640586282873}, {"Real Matrix Element"=8.01473233974601, "Real Matrix Element"=16.007751369154814}, {"Real Matrix Element"=8.132120351179067, "Real Matrix Element"=15.881234472774437}, {"Real Matrix Element"=8.139068154366894, "Real Matrix Element"=15.892621560233586}, {"Real Matrix Element"=7.97016861327872, "Real Matrix Element"=16.16443486144255}, {"Real Matrix Element"=7.804220115475935, "Real Matrix Element"=16.276161037246084}, {"Real Matrix Element"=7.823567848629205, "Real Matrix Element"=16.28175317293954}, {"Real Matrix Element"=7.7772954876375575, "Real Matrix Element"=16.374895327387897}, {"Real Matrix Element"=7.720812515765172, "Real Matrix Element"=16.39090670473211}, {"Real Matrix Element"=7.747002652427052, "Real Matrix Element"=16.427967839910323}, {"Real Matrix Element"=7.770274479889653, "Real Matrix Element"=16.453331006794706}, {"Real Matrix Element"=7.605063938113692, "Real Matrix Element"=16.788070554978496}, {"Real Matrix Element"=7.520251399703272, "Real Matrix Element"=16.909375081451802}, {"Real Matrix Element"=7.516756356103126, "Real Matrix Element"=16.85729725874903}, {"Real Matrix Element"=7.462735585433237, "Real Matrix Element"=16.942658292956374}, {"Real Matrix Element"=7.261335728252355, "Real Matrix Element"=17.10239812718219}, {"Real Matrix Element"=7.216504461350804, "Real Matrix Element"=17.08888715729156}, {"Real Matrix Element"=7.105342968917498, "Real Matrix Element"=17.16367677628471}, {"Real Matrix Element"=7.115049913634879, "Real Matrix Element"=17.150624614959103}, {"Real Matrix Element"=6.916247841222035, "Real Matrix Element"=17.286190190979926}, {"Real Matrix Element"=6.874378436736089, "Real Matrix Element"=17.302897013942445}, {"Real Matrix Element"=6.820785706177385, "Real Matrix Element"=17.348705967412833}, {"Real Matrix Element"=6.764550952853075, "Real Matrix Element"=17.342854775130935}, {"Real Matrix Element"=6.6907864148539655, "Real Matrix Element"=17.383948258975092}, {"Real Matrix Element"=6.546844819313545, "Real Matrix Element"=17.44139903938426}, {"Real Matrix Element"=6.508024105249184, "Real Matrix Element"=17.583098420068502}, {"Real Matrix Element"=6.429973482105771, "Real Matrix Element"=17.63311485006733}, {"Real Matrix Element"=6.242656603847212, "Real Matrix Element"=17.71972365920509}, {"Real Matrix Element"=6.235934315732861, "Real Matrix Element"=17.756149759697557}, {"Real Matrix Element"=6.194673312101115, "Real Matrix Element"=17.79328802327805}, {"Real Matrix Element"=6.1526545273278455, "Real Matrix Element"=17.852530728848475}, {"Real Matrix Element"=5.871520703735831, "Real Matrix Element"=18.007979643275977}, {"Real Matrix Element"=5.929134739845566, "Real Matrix Element"=17.96015049346766}, {"Real Matrix Element"=5.832135124337329, "Real Matrix Element"=18.04816316973673}, {"Real Matrix Element"=5.967064740010496, "Real Matrix Element"=17.97717829176057}, {"Real Matrix Element"=5.693999105189158, "Real Matrix Element"=18.343010213021362}, {"Real Matrix Element"=5.657777441268699, "Real Matrix Element"=18.476401281653537}, {"Real Matrix Element"=5.5816579630148215, "Real Matrix Element"=18.45900539066518}, {"Real Matrix Element"=5.471451974654111, "Real Matrix Element"=18.43335547447642}, {"Real Matrix Element"=5.4770288819161195, "Real Matrix Element"=18.39464668101496}, {"Real Matrix Element"=5.355970465487254, "Real Matrix Element"=18.483185733814466}, {"Real Matrix Element"=5.264388458517377, "Real Matrix Element"=18.501127195400407}, {"Real Matrix Element"=5.169188373346975, "Real Matrix Element"=18.54399284383817}, {"Real Matrix Element"=5.008090624165736, "Real Matrix Element"=18.709909767078567}, {"Real Matrix Element"=4.90512184465543, "Real Matrix Element"=18.783411346023158}, {"Real Matrix Element"=4.770399614829969, "Real Matrix Element"=18.827424260002633}, {"Real Matrix Element"=4.934389499934613, "Real Matrix Element"=18.709935485940512}, {"Real Matrix Element"=4.790398707376359, "Real Matrix Element"=18.815157777795378}, {"Real Matrix Element"=4.6448552202313556, "Real Matrix Element"=18.961423615210027}, {"Real Matrix Element"=4.584140732960507, "Real Matrix Element"=19.001544915397936}, {"Real Matrix Element"=4.447535761048353, "Real Matrix Element"=19.10837117578333}, {"Real Matrix Element"=4.420746510293564, "Real Matrix Element"=19.14004834260601}, {"Real Matrix Element"=4.407738971186914, "Real Matrix Element"=19.057685082677242}, {"Real Matrix Element"=4.322895588689966, "Real Matrix Element"=19.05297935502187}, {"Real Matrix Element"=4.116610114432733, "Real Matrix Element"=19.10949737568445}, {"Real Matrix Element"=4.036538754494437, "Real Matrix Element"=19.135558836745787}, {"Real Matrix Element"=4.0659722308264765, "Real Matrix Element"=19.11237169116917}, {"Real Matrix Element"=4.011251340535824, "Real Matrix Element"=19.121489602294602}, {"Real Matrix Element"=3.8813738110924367, "Real Matrix Element"=19.17830147827182}, {"Real Matrix Element"=3.552248934946511, "Real Matrix Element"=19.23611733939429}, {"Real Matrix Element"=3.484484028575303, "Real Matrix Element"=19.252542005902868}, {"Real Matrix Element"=3.4099767227715545, "Real Matrix Element"=19.3378961231521}, {"Real Matrix Element"=3.2020616673775484, "Real Matrix Element"=19.448725413186764}, {"Real Matrix Element"=3.1192441080607023, "Real Matrix Element"=19.48654300213322}, {"Real Matrix Element"=3.0556502606347555, "Real Matrix Element"=19.522677368255806}, {"Real Matrix Element"=2.823437065926758, "Real Matrix Element"=19.600059673424152}, {"Real Matrix Element"=3.022888752186925, "Real Matrix Element"=19.49313591389503}, {"Real Matrix Element"=2.728618357396417, "Real Matrix Element"=19.600371672071766}, {"Real Matrix Element"=2.851344902717735, "Real Matrix Element"=19.582789687464242}, {"Real Matrix Element"=2.675244255465557, "Real Matrix Element"=19.632690164368636}, {"Real Matrix Element"=2.6676780627470444, "Real Matrix Element"=19.695959607597164}, {"Real Matrix Element"=2.4816192594650057, "Real Matrix Element"=19.650311321508656}, {"Real Matrix Element"=2.294536770780834, "Real Matrix Element"=19.72330949579401}, {"Real Matrix Element"=2.1992378212083605, "Real Matrix Element"=19.74639220350119}, {"Real Matrix Element"=2.073108562255909, "Real Matrix Element"=19.798198084554095}, {"Real Matrix Element"=1.834078903092064, "Real Matrix Element"=19.867882747575436}, {"Real Matrix Element"=1.9612253478760155, "Real Matrix Element"=19.835902932840394}, {"Real Matrix Element"=1.801893578295809, "Real Matrix Element"=19.883518886596146}, {"Real Matrix Element"=1.7782481206074372, "Real Matrix Element"=19.89746212183498}, {"Real Matrix Element"=1.7294953057235205, "Real Matrix Element"=19.883192714452456}, {"Real Matrix Element"=1.592040801083075, "Real Matrix Element"=19.81313647836882}, {"Real Matrix Element"=1.3960736084984398, "Real Matrix Element"=19.96443738911608}, {"Real Matrix Element"=1.3871521010028922, "Real Matrix Element"=19.98335168703091}, {"Real Matrix Element"=1.1757052255042209, "Real Matrix Element"=19.950959239818527}, {"Real Matrix Element"=1.035041905422353, "Real Matrix Element"=19.938430444676086}, {"Real Matrix Element"=0.9270806636831437, "Real Matrix Element"=19.775465775495753}, {"Real Matrix Element"=0.9553449375418361, "Real Matrix Element"=19.879690631930647}, {"Real Matrix Element"=0.968591548354444, "Real Matrix Element"=19.881033710192423}, {"Real Matrix Element"=0.9189479167938511, "Real Matrix Element"=19.90458099452115}, {"Real Matrix Element"=0.6590978788503883, "Real Matrix Element"=19.89036524522598}, {"Real Matrix Element"=0.6614303466338883, "Real Matrix Element"=19.888484646400986}, {"Real Matrix Element"=0.6753231322169541, "Real Matrix Element"=19.898615305959613}, {"Real Matrix Element"=0.3740206996037374, "Real Matrix Element"=19.892774198214607}, {"Real Matrix Element"=0.34739155748461714, "Real Matrix Element"=19.905092290711565}, {"Real Matrix Element"=0.06965176792300488, "Real Matrix Element"=19.914124003117273}, {"Real Matrix Element"=0.023927283074007218, "Real Matrix Element"=19.872927757195697}, {"Real Matrix Element"=-0.024769183074944502, "Real Matrix Element"=19.84846913838246}, {"Real Matrix Element"=-0.28191898281748745, "Real Matrix Element"=19.873170757975405}, {"Real Matrix Element"=-0.1678447036901971, "Real Matrix Element"=19.893084017594095}, {"Real Matrix Element"=-0.3445585180695523, "Real Matrix Element"=19.84718370034653}, {"Real Matrix Element"=-0.4039746127380327, "Real Matrix Element"=19.862749914184015}, {"Real Matrix Element"=-0.4988911864353056, "Real Matrix Element"=19.92216636088148}, {"Real Matrix Element"=-0.5643302399048143, "Real Matrix Element"=19.910109599275742}, {"Real Matrix Element"=-0.7147279396542117, "Real Matrix Element"=19.941280871595517}, {"Real Matrix Element"=-0.9165485695827587, "Real Matrix Element"=19.95850582652412}, {"Real Matrix Element"=-0.9517676055743982, "Real Matrix Element"=19.944700736523565}, {"Real Matrix Element"=-1.1097808148756272, "Real Matrix Element"=19.92734124328764}, {"Real Matrix Element"=-1.2634792924212725, "Real Matrix Element"=19.892668825849704}, {"Real Matrix Element"=-1.3433341120474753, "Real Matrix Element"=19.89371424818296}, {"Real Matrix Element"=-1.5049842740970856, "Real Matrix Element"=19.853014965792635}, {"Real Matrix Element"=-1.3851662317760274, "Real Matrix Element"=19.876204736646496}, {"Real Matrix Element"=-1.4082342193458108, "Real Matrix Element"=19.894487051587323}, {"Real Matrix Element"=-1.4114331169010932, "Real Matrix Element"=19.935971638082204}, {"Real Matrix Element"=-1.8123237625176136, "Real Matrix Element"=20.04423788570179}, {"Real Matrix Element"=-1.8849191620771533, "Real Matrix Element"=19.904689495528643}, {"Real Matrix Element"=-1.9555477897892461, "Real Matrix Element"=19.8457447576879}, {"Real Matrix Element"=-2.0645622222633286, "Real Matrix Element"=19.827961197229197}, {"Real Matrix Element"=-2.1406975808829487, "Real Matrix Element"=19.80485104321441}, {"Real Matrix Element"=-2.1233615854921655, "Real Matrix Element"=19.885537725349558}, {"Real Matrix Element"=-2.3623616754805163, "Real Matrix Element"=19.77948237862293}, {"Real Matrix Element"=-2.526774395095306, "Real Matrix Element"=19.77066171844839}, {"Real Matrix Element"=-2.61880688676897, "Real Matrix Element"=19.70017785467804}, {"Real Matrix Element"=-2.5099372675829117, "Real Matrix Element"=19.715281836909153}, {"Real Matrix Element"=-2.7052675058361193, "Real Matrix Element"=19.615371947847407}, {"Real Matrix Element"=-2.84330079373202, "Real Matrix Element"=19.63695050288629}, {"Real Matrix Element"=-2.6716147833638, "Real Matrix Element"=19.64061099094386}, {"Real Matrix Element"=-2.963397654601283, "Real Matrix Element"=19.56935467562357}, {"Real Matrix Element"=-3.0410072150630567, "Real Matrix Element"=19.58489843180442}, {"Real Matrix Element"=-3.133280797659109, "Real Matrix Element"=19.57114161771706}, {"Real Matrix Element"=-2.942411401549076, "Real Matrix Element"=19.614952936402727}, {"Real Matrix Element"=-2.9117769215623803, "Real Matrix Element"=19.657078266140953}, {"Real Matrix Element"=-3.199554798619233, "Real Matrix Element"=19.554811886016147}, {"Real Matrix Element"=-3.3533912633229535, "Real Matrix Element"=19.569997291962988}, {"Real Matrix Element"=-3.396567797114521, "Real Matrix Element"=19.546609914452134}, {"Real Matrix Element"=-3.345036327786078, "Real Matrix Element"=19.523711330629524}, {"Real Matrix Element"=-3.681830023200861, "Real Matrix Element"=19.469238723834906}, {"Real Matrix Element"=-3.6824060651192774, "Real Matrix Element"=19.41721702384578}, {"Real Matrix Element"=-3.9184629462821374, "Real Matrix Element"=19.3274857608243}, {"Real Matrix Element"=-4.096320572968272, "Real Matrix Element"=19.1053820049069}, {"Real Matrix Element"=-4.249416160509664, "Real Matrix Element"=18.974252587201065}, {"Real Matrix Element"=-4.306032538112409, "Real Matrix Element"=18.93162270823365}, {"Real Matrix Element"=-4.672826660861853, "Real Matrix Element"=18.72464108945378}, {"Real Matrix Element"=-4.781245076258591, "Real Matrix Element"=18.59384328696795}, {"Real Matrix Element"=-4.589452800613404, "Real Matrix Element"=18.684667287549573}, {"Real Matrix Element"=-4.883761024739016, "Real Matrix Element"=18.621406629537915}, {"Real Matrix Element"=-4.908059362275409, "Real Matrix Element"=18.63045900425087}, {"Real Matrix Element"=-4.8295773615523565, "Real Matrix Element"=18.689962439356822}, {"Real Matrix Element"=-4.863348913262107, "Real Matrix Element"=18.66526942223912}, {"Real Matrix Element"=-4.930999459895792, "Real Matrix Element"=18.595177854593018}, {"Real Matrix Element"=-4.9578564084611365, "Real Matrix Element"=18.64408094891442}, {"Real Matrix Element"=-5.030231865458711, "Real Matrix Element"=18.583642663847968}, {"Real Matrix Element"=-5.023715750427326, "Real Matrix Element"=18.502485145506913}, {"Real Matrix Element"=-5.169900998277981, "Real Matrix Element"=18.49449389569717}, {"Real Matrix Element"=-5.196761133801141, "Real Matrix Element"=18.503630016450238}, {"Real Matrix Element"=-5.509711716226101, "Real Matrix Element"=18.304419353770815}, {"Real Matrix Element"=-5.493490819761743, "Real Matrix Element"=18.356989232391772}, {"Real Matrix Element"=-5.5908448746272095, "Real Matrix Element"=18.34094533796089}, {"Real Matrix Element"=-5.571321011963367, "Real Matrix Element"=18.306316565029952}, {"Real Matrix Element"=-5.7986398082973585, "Real Matrix Element"=18.182684571805936}, {"Real Matrix Element"=-5.870955182286434, "Real Matrix Element"=18.03258174521602}, {"Real Matrix Element"=-6.130065434027463, "Real Matrix Element"=17.888086503275584}, {"Real Matrix Element"=-6.175996917320804, "Real Matrix Element"=17.86482637976397}, {"Real Matrix Element"=-6.167817277873238, "Real Matrix Element"=17.828946799808932}, {"Real Matrix Element"=-6.2759314742047705, "Real Matrix Element"=17.75134899647914}, {"Real Matrix Element"=-6.231817904297413, "Real Matrix Element"=17.720932302001387}, {"Real Matrix Element"=-6.332937694730571, "Real Matrix Element"=17.7362369464768}, {"Real Matrix Element"=-6.435929932971732, "Real Matrix Element"=17.641114887767284}, {"Real Matrix Element"=-6.526540649669762, "Real Matrix Element"=17.6046364752875}, {"Real Matrix Element"=-6.644684398371386, "Real Matrix Element"=17.577802951195586}, {"Real Matrix Element"=-6.7157662824453315, "Real Matrix Element"=17.50352724643216}, {"Real Matrix Element"=-6.6519943548040095, "Real Matrix Element"=17.526883655167087}, {"Real Matrix Element"=-6.898749336038432, "Real Matrix Element"=17.394375699353933}, {"Real Matrix Element"=-6.971168373930361, "Real Matrix Element"=17.294025495664783}, {"Real Matrix Element"=-7.161250547756226, "Real Matrix Element"=17.126553119555215}, {"Real Matrix Element"=-6.953387521235868, "Real Matrix Element"=17.310232571142787}, {"Real Matrix Element"=-7.298628311719389, "Real Matrix Element"=17.03230171123997}, {"Real Matrix Element"=-7.413502905205735, "Real Matrix Element"=16.869259773048363}, {"Real Matrix Element"=-7.466074264710675, "Real Matrix Element"=16.894597176583577}, {"Real Matrix Element"=-7.446612135479184, "Real Matrix Element"=16.90228387362881}, {"Real Matrix Element"=-7.568401036545141, "Real Matrix Element"=16.65112475687052}, {"Real Matrix Element"=-7.45894065322769, "Real Matrix Element"=16.808493119395152}, {"Real Matrix Element"=-7.454709581573706, "Real Matrix Element"=16.707718840662448}, {"Real Matrix Element"=-7.5350559652560225, "Real Matrix Element"=16.66749052928071}, {"Real Matrix Element"=-7.585295880098653, "Real Matrix Element"=16.496076274372538}, {"Real Matrix Element"=-7.741589440899461, "Real Matrix Element"=16.19316988317955}, {"Real Matrix Element"=-7.798544091965774, "Real Matrix Element"=15.911063743590177}, {"Real Matrix Element"=-7.7559411851983375, "Real Matrix Element"=15.811260823032683}, {"Real Matrix Element"=-7.763564835467262, "Real Matrix Element"=15.844939860506505}, {"Real Matrix Element"=-7.855048204901442, "Real Matrix Element"=15.701525276270171}, {"Real Matrix Element"=-7.916502253624716, "Real Matrix Element"=15.728063591320087}, {"Real Matrix Element"=-7.895415426468601, "Real Matrix Element"=15.612226201174925}, {"Real Matrix Element"=-7.99121131582355, "Real Matrix Element"=15.70919531674548}, {"Real Matrix Element"=-8.17260699527194, "Real Matrix Element"=15.524804429018129}, {"Real Matrix Element"=-8.242407304136137, "Real Matrix Element"=15.434618357167961}, {"Real Matrix Element"=-8.200040586408642, "Real Matrix Element"=15.44575013685018}, {"Real Matrix Element"=-8.302662361729709, "Real Matrix Element"=15.37680903440047}, {"Real Matrix Element"=-8.485343716367767, "Real Matrix Element"=15.014278865431704}, {"Real Matrix Element"=-8.443594171567126, "Real Matrix Element"=15.170855965483263}, {"Real Matrix Element"=-8.49333941049472, "Real Matrix Element"=15.120675380902735}, {"Real Matrix Element"=-8.502363307251999, "Real Matrix Element"=15.094954432190905}, {"Real Matrix Element"=-8.666628578611427, "Real Matrix Element"=14.862168202021238}, {"Real Matrix Element"=-8.58631437849168, "Real Matrix Element"=15.049760679033625}, {"Real Matrix Element"=-8.707748018433765, "Real Matrix Element"=14.862910128338488}, {"Real Matrix Element"=-8.598898898970955, "Real Matrix Element"=14.925502448906972}, {"Real Matrix Element"=-8.66494156238723, "Real Matrix Element"=14.777626190332288}, {"Real Matrix Element"=-8.807404982430375, "Real Matrix Element"=14.513541836699199}, {"Real Matrix Element"=-8.707876030141147, "Real Matrix Element"=14.68296875784013}, {"Real Matrix Element"=-8.801290724580186, "Real Matrix Element"=14.468321575118676}, {"Real Matrix Element"=-8.96037757368756, "Real Matrix Element"=14.303751943548052}, {"Real Matrix Element"=-9.11069929611384, "Real Matrix Element"=14.156738268140238}, {"Real Matrix Element"=-9.246200560552511, "Real Matrix Element"=13.996295272387693}, {"Real Matrix Element"=-9.206510057520768, "Real Matrix Element"=14.13093175349474}, {"Real Matrix Element"=-9.354021818059323, "Real Matrix Element"=13.940520925054058}, {"Real Matrix Element"=-9.24529248016141, "Real Matrix Element"=13.966175713886788}, {"Real Matrix Element"=-9.27524610297175, "Real Matrix Element"=13.952150274394922}, {"Real Matrix Element"=-9.387555203486437, "Real Matrix Element"=13.868345439384868}, {"Real Matrix Element"=-9.281871818375997, "Real Matrix Element"=13.92886646736536}, {"Real Matrix Element"=-9.408518690295164, "Real Matrix Element"=13.814432073699908}, {"Real Matrix Element"=-9.53893123370487, "Real Matrix Element"=13.67508335899547}, {"Real Matrix Element"=-9.689273152351667, "Real Matrix Element"=13.369835931553265}, {"Real Matrix Element"=-9.55335725556932, "Real Matrix Element"=13.580199239466301}, {"Real Matrix Element"=-9.61849587724122, "Real Matrix Element"=13.457692425073661}, {"Real Matrix Element"=-9.719732689923585, "Real Matrix Element"=13.147683910698467}, {"Real Matrix Element"=-9.71081418030636, "Real Matrix Element"=13.214964673483188}, {"Real Matrix Element"=-9.725395169164548, "Real Matrix Element"=13.1631786444472}, {"Real Matrix Element"=-9.7918084737485, "Real Matrix Element"=12.990986839481458}, {"Real Matrix Element"=-9.793563567142714, "Real Matrix Element"=12.74668956436983}, {"Real Matrix Element"=-9.787969858505862, "Real Matrix Element"=12.749278580335373}, {"Real Matrix Element"=-9.802120627073649, "Real Matrix Element"=12.609534248935903}, {"Real Matrix Element"=-9.796136811346596, "Real Matrix Element"=12.678047708624266}, {"Real Matrix Element"=-9.836250238400014, "Real Matrix Element"=12.341638112411097}, {"Real Matrix Element"=-9.796818046002471, "Real Matrix Element"=12.116044304132059}, {"Real Matrix Element"=-9.719505053478738, "Real Matrix Element"=11.951606205950856}, {"Real Matrix Element"=-9.694756109049086, "Real Matrix Element"=11.99649996202263}, {"Real Matrix Element"=-9.744338324134223, "Real Matrix Element"=11.895104216865844}, {"Real Matrix Element"=-9.658610864251104, "Real Matrix Element"=11.600208119752889}, {"Real Matrix Element"=-9.786653681266607, "Real Matrix Element"=12.13466035817673}, {"Real Matrix Element"=-9.682835009819458, "Real Matrix Element"=11.629427999856654}, {"Real Matrix Element"=-9.693979442225077, "Real Matrix Element"=11.378566950766409}, {"Real Matrix Element"=-9.738185451281467, "Real Matrix Element"=11.210851533747093}, {"Real Matrix Element"=-9.762023023868707, "Real Matrix Element"=11.399475740916136}, {"Real Matrix Element"=-9.770697598595865, "Real Matrix Element"=11.377015469291262}, {"Real Matrix Element"=-9.733701366400933, "Real Matrix Element"=11.167448309860886}, {"Real Matrix Element"=-9.694369347687468, "Real Matrix Element"=10.945912486694912}, {"Real Matrix Element"=-9.812826512647552, "Real Matrix Element"=10.781154905016699}, {"Real Matrix Element"=-9.957465156990658, "Real Matrix Element"=10.625404383068478}, {"Real Matrix Element"=-9.890557682445301, "Real Matrix Element"=10.826727906751943}, {"Real Matrix Element"=-9.890504859931548, "Real Matrix Element"=10.682661692879591}, {"Real Matrix Element"=-10.036472953968891, "Real Matrix Element"=10.450065401552578}, {"Real Matrix Element"=-10.01745284474525, "Real Matrix Element"=10.178571428214259}, {"Real Matrix Element"=-9.992582176936734, "Real Matrix Element"=10.214471270322854}, {"Real Matrix Element"=-10.002558845952045, "Real Matrix Element"=10.143339534664841}, {"Real Matrix Element"=-9.958407001251084, "Real Matrix Element"=10.04377124805277}, {"Real Matrix Element"=-9.96363141147907, "Real Matrix Element"=10.025430596839119}, {"Real Matrix Element"=-9.929395881257518, "Real Matrix Element"=10.055560986505009}, {"Real Matrix Element"=-9.993035786907793, "Real Matrix Element"=9.766460848893958}, {"Real Matrix Element"=-10.001533562638347, "Real Matrix Element"=9.727437852936793}, {"Real Matrix Element"=-10.00588600697634, "Real Matrix Element"=9.6169826622764}, {"Real Matrix Element"=-9.998567929540755, "Real Matrix Element"=9.469019316396}, {"Real Matrix Element"=-10.02103994220378, "Real Matrix Element"=9.49275100672555}, {"Real Matrix Element"=-10.058287894619871, "Real Matrix Element"=9.275942788669822}, {"Real Matrix Element"=-10.03475740479754, "Real Matrix Element"=9.306539793031392}, {"Real Matrix Element"=-10.05129974772351, "Real Matrix Element"=9.156329334531938}, {"Real Matrix Element"=-10.004863941479645, "Real Matrix Element"=8.93206744487254}, {"Real Matrix Element"=-10.003384510458565, "Real Matrix Element"=8.931553301794038}, {"Real Matrix Element"=-9.9814540523903, "Real Matrix Element"=8.74912417196654}, {"Real Matrix Element"=-9.93461208937163, "Real Matrix Element"=8.388235125306199}, {"Real Matrix Element"=-9.931030616286291, "Real Matrix Element"=8.494792614664192}, {"Real Matrix Element"=-9.826900985442151, "Real Matrix Element"=8.375666647783614}, {"Real Matrix Element"=-9.773862975748273, "Real Matrix Element"=8.321414072768277}, {"Real Matrix Element"=-9.80026668585236, "Real Matrix Element"=8.374126988758814}, {"Real Matrix Element"=-9.814567856312273, "Real Matrix Element"=8.303417741553954}, {"Real Matrix Element"=-9.928518062613318, "Real Matrix Element"=8.457511685842656}, {"Real Matrix Element"=-9.905105301418647, "Real Matrix Element"=8.369713674885086}, {"Real Matrix Element"=-9.791603262055443, "Real Matrix Element"=8.191453923331878}, {"Real Matrix Element"=-9.748260221686213, "Real Matrix Element"=8.088808152236046}, {"Real Matrix Element"=-9.627984469694836, "Real Matrix Element"=7.8341435816722464}, {"Real Matrix Element"=-9.565841621157219, "Real Matrix Element"=7.602780211738581}, {"Real Matrix Element"=-9.551562699469361, "Real Matrix Element"=7.357144117897573}, {"Real Matrix Element"=-9.613159720461073, "Real Matrix Element"=7.284044944839619}, {"Real Matrix Element"=-9.584138043138203, "Real Matrix Element"=7.342180604914518}, {"Real Matrix Element"=-9.497361403029931, "Real Matrix Element"=7.034098998036428}, {"Real Matrix Element"=-9.4756388982028, "Real Matrix Element"=6.97163988498242}, {"Real Matrix Element"=-9.439931447890158, "Real Matrix Element"=7.03399166329044}, {"Real Matrix Element"=-9.382531094618487, "Real Matrix Element"=6.894637229881391}, {"Real Matrix Element"=-9.23723723563261, "Real Matrix Element"=6.591521757003052}, {"Real Matrix Element"=-9.161679603577854, "Real Matrix Element"=6.395840099137495}, {"Real Matrix Element"=-9.112720270458732, "Real Matrix Element"=6.337059062549551}, {"Real Matrix Element"=-9.239361105051438, "Real Matrix Element"=6.478800134437494}, {"Real Matrix Element"=-9.158076491940731, "Real Matrix Element"=6.3418215578384975}, {"Real Matrix Element"=-9.12910356481767, "Real Matrix Element"=6.32252707561224}, {"Real Matrix Element"=-9.010802554588986, "Real Matrix Element"=6.128022173520232}, {"Real Matrix Element"=-9.035901375688903, "Real Matrix Element"=6.133012659761219}, {"Real Matrix Element"=-8.982971736332969, "Real Matrix Element"=6.077718828511109}, {"Real Matrix Element"=-8.936988385043236, "Real Matrix Element"=5.854790463221662}, {"Real Matrix Element"=-8.918448602058477, "Real Matrix Element"=5.694840127909285}, {"Real Matrix Element"=-8.90915359095002, "Real Matrix Element"=5.585235695447742}, {"Real Matrix Element"=-8.979326139958324, "Real Matrix Element"=5.674981660060146}, {"Real Matrix Element"=-8.959656321313783, "Real Matrix Element"=5.55735399440483}, {"Real Matrix Element"=-8.901873852567906, "Real Matrix Element"=5.546355274514736}, {"Real Matrix Element"=-8.953153212658753, "Real Matrix Element"=5.625024019127606}, {"Real Matrix Element"=-8.800518005382045, "Real Matrix Element"=5.285102985693751}, {"Real Matrix Element"=-8.859448920303684, "Real Matrix Element"=5.275393853527409}, {"Real Matrix Element"=-8.816349985249776, "Real Matrix Element"=5.2533966733122055}, {"Real Matrix Element"=-8.627310082919823, "Real Matrix Element"=4.783032194344177}, {"Real Matrix Element"=-8.630885235726467, "Real Matrix Element"=4.859543897106574}, {"Real Matrix Element"=-8.615664495824063, "Real Matrix Element"=4.864654298605316}, {"Real Matrix Element"=-8.533264476928178, "Real Matrix Element"=4.644527102713774}, {"Real Matrix Element"=-8.466068093726912, "Real Matrix Element"=4.641687945516618}, {"Real Matrix Element"=-8.404648200872714, "Real Matrix Element"=4.682902207100471}, {"Real Matrix Element"=-8.382862294730334, "Real Matrix Element"=4.5869395955578085}, {"Real Matrix Element"=-8.164556487535256, "Real Matrix Element"=4.474387288442273}, {"Real Matrix Element"=-8.084602643552635, "Real Matrix Element"=4.363425332033597}, {"Real Matrix Element"=-8.222753869252701, "Real Matrix Element"=4.513409070054083}, {"Real Matrix Element"=-8.038668936549524, "Real Matrix Element"=4.323735302252803}, {"Real Matrix Element"=-7.866088410063709, "Real Matrix Element"=4.080698562686548}, {"Real Matrix Element"=-7.7161863686882795, "Real Matrix Element"=3.8722394400367963}, {"Real Matrix Element"=-7.783451393026299, "Real Matrix Element"=3.8941497489882804}, {"Real Matrix Element"=-7.778841607426628, "Real Matrix Element"=3.8682047447568975}, {"Real Matrix Element"=-7.725121457967291, "Real Matrix Element"=3.7948065182575914}, {"Real Matrix Element"=-7.726012029026685, "Real Matrix Element"=3.766101248834909}, {"Real Matrix Element"=-7.570690690385876, "Real Matrix Element"=3.5484546615680057}, {"Real Matrix Element"=-7.695328559588584, "Real Matrix Element"=3.704582586624135}, {"Real Matrix Element"=-7.653706587881133, "Real Matrix Element"=3.6421022909425274}, {"Real Matrix Element"=-7.588656172758382, "Real Matrix Element"=3.530750959256342}, {"Real Matrix Element"=-7.430752144438466, "Real Matrix Element"=3.259829612697665}, {"Real Matrix Element"=-7.355238538006462, "Real Matrix Element"=3.108990096975488}, {"Real Matrix Element"=-7.379093027204378, "Real Matrix Element"=3.2114389517045194}, {"Real Matrix Element"=-7.304606077094906, "Real Matrix Element"=3.1035536131316688}, {"Real Matrix Element"=-7.178213319684464, "Real Matrix Element"=3.006819994351996}, {"Real Matrix Element"=-7.274386467955736, "Real Matrix Element"=3.0944145392096605}, {"Real Matrix Element"=-7.038692580582773, "Real Matrix Element"=2.9324645727046175}, {"Real Matrix Element"=-6.7760399070323745, "Real Matrix Element"=2.7687240103644686}, {"Real Matrix Element"=-6.825536656961252, "Real Matrix Element"=2.8138308948455992}, {"Real Matrix Element"=-6.589532106448522, "Real Matrix Element"=2.625695961597279}, {"Real Matrix Element"=-6.6408942389508265, "Real Matrix Element"=2.6019277111057213}, {"Real Matrix Element"=-6.684871035041256, "Real Matrix Element"=2.6534494856874904}, {"Real Matrix Element"=-6.849879734279698, "Real Matrix Element"=2.7083659408499807}, {"Real Matrix Element"=-6.645014267627354, "Real Matrix Element"=2.5939935611173897}, {"Real Matrix Element"=-6.379627614509241, "Real Matrix Element"=2.432248363150846}, {"Real Matrix Element"=-6.209334695182468, "Real Matrix Element"=2.339858641077935}, {"Real Matrix Element"=-6.1389242982833325, "Real Matrix Element"=2.282201744821764}, {"Real Matrix Element"=-6.233767807538561, "Real Matrix Element"=2.3246839929949634}, {"Real Matrix Element"=-6.248184105766464, "Real Matrix Element"=2.3219295677992466}, {"Real Matrix Element"=-6.107972594651465, "Real Matrix Element"=2.154355390572905}, {"Real Matrix Element"=-5.922027456301764, "Real Matrix Element"=1.9798984957785233}, {"Real Matrix Element"=-5.935168292435575, "Real Matrix Element"=2.0116762170575337}, {"Real Matrix Element"=-5.78392793560016, "Real Matrix Element"=1.9346149257198568}, {"Real Matrix Element"=-5.8002810358183226, "Real Matrix Element"=1.874281743576818}, {"Real Matrix Element"=-5.62763103279624, "Real Matrix Element"=1.6861871842420348}, {"Real Matrix Element"=-5.477979948074627, "Real Matrix Element"=1.5597250988237925}, {"Real Matrix Element"=-5.486129146312208, "Real Matrix Element"=1.5734176596228784}, {"Real Matrix Element"=-5.442692689826321, "Real Matrix Element"=1.489282336586151}, {"Real Matrix Element"=-5.2939843241784175, "Real Matrix Element"=1.4372287721229628}, {"Real Matrix Element"=-5.357304131427993, "Real Matrix Element"=1.5310608832897672}, {"Real Matrix Element"=-5.0954208961810865, "Real Matrix Element"=1.5037706636641546}, {"Real Matrix Element"=-5.057975599406152, "Real Matrix Element"=1.4154026875705301}, {"Real Matrix Element"=-4.995653035151117, "Real Matrix Element"=1.3217330495422401}, {"Real Matrix Element"=-4.913551906245581, "Real Matrix Element"=1.3228207098344609}, {"Real Matrix Element"=-4.8428643529416044, "Real Matrix Element"=1.390610330890255}, {"Real Matrix Element"=-4.655835831545926, "Real Matrix Element"=1.3007468383674627}, {"Real Matrix Element"=-4.549479459110537, "Real Matrix Element"=1.1274219004127886}, {"Real Matrix Element"=-4.345308832229479, "Real Matrix Element"=1.0552718794213016}, {"Real Matrix Element"=-4.515663303703823, "Real Matrix Element"=1.156122606807663}, {"Real Matrix Element"=-4.414295405458624, "Real Matrix Element"=1.1526859147638304}, {"Real Matrix Element"=-4.206874707206558, "Real Matrix Element"=1.0680689179108522}, {"Real Matrix Element"=-4.099116046199024, "Real Matrix Element"=0.9701826543018748}, {"Real Matrix Element"=-4.030356449370558, "Real Matrix Element"=1.0147464597611238}, {"Real Matrix Element"=-4.036315864561008, "Real Matrix Element"=0.9022144875190019}, {"Real Matrix Element"=-3.895272758476922, "Real Matrix Element"=0.798521284404001}, {"Real Matrix Element"=-3.941693527569419, "Real Matrix Element"=0.8109108187870046}, {"Real Matrix Element"=-3.7535219454346613, "Real Matrix Element"=0.7856697902790329}, {"Real Matrix Element"=-3.5192647160295305, "Real Matrix Element"=0.630068932932053}, {"Real Matrix Element"=-3.5176136814660075, "Real Matrix Element"=0.6439524519520858}, {"Real Matrix Element"=-3.4648096712747862, "Real Matrix Element"=0.6057876042943932}, {"Real Matrix Element"=-3.5063010891013615, "Real Matrix Element"=0.6111560262439781}, {"Real Matrix Element"=-3.377877233881448, "Real Matrix Element"=0.5911500177504763}, {"Real Matrix Element"=-3.14690158366852, "Real Matrix Element"=0.47341849771718075}, {"Real Matrix Element"=-3.0490995228301245, "Real Matrix Element"=0.42689493001799345}, {"Real Matrix Element"=-2.7557116500250234, "Real Matrix Element"=0.3806716434745836}, {"Real Matrix Element"=-2.792983385618109, "Real Matrix Element"=0.38590806864939536}, {"Real Matrix Element"=-2.833526667566114, "Real Matrix Element"=0.40992656055418997}, {"Real Matrix Element"=-2.5844338141324417, "Real Matrix Element"=0.2750911871990285}, {"Real Matrix Element"=-2.6042861041307623, "Real Matrix Element"=0.331892515329684}, {"Real Matrix Element"=-2.5374861445407193, "Real Matrix Element"=0.34231691087221783}, {"Real Matrix Element"=-2.3572022472718794, "Real Matrix Element"=0.2921516092968695}, {"Real Matrix Element"=-2.119799963506989, "Real Matrix Element"=0.19303344195971767}, {"Real Matrix Element"=-2.0458714883080207, "Real Matrix Element"=0.11630591211116548}, {"Real Matrix Element"=-2.1866237101570545, "Real Matrix Element"=0.19349015480168413}, {"Real Matrix Element"=-1.923129741346614, "Real Matrix Element"=0.13783071026578972}, {"Real Matrix Element"=-2.0121067290735395, "Real Matrix Element"=0.15857262050643978}, {"Real Matrix Element"=-1.8508442668189387, "Real Matrix Element"=0.16250288571348856}, {"Real Matrix Element"=-1.9013977679104104, "Real Matrix Element"=0.1780905127120426}, {"Real Matrix Element"=-1.8075719712693503, "Real Matrix Element"=0.180762332767096}, {"Real Matrix Element"=-1.6737509864591378, "Real Matrix Element"=0.10320346836069397}, {"Real Matrix Element"=-1.5148766550176302, "Real Matrix Element"=-0.04319276409272923}, {"Real Matrix Element"=-1.2445135860368128, "Real Matrix Element"=-0.17326082230508838}, {"Real Matrix Element"=-1.1020134153205992, "Real Matrix Element"=0.03337844653332904}, {"Real Matrix Element"=-1.1304729353995082, "Real Matrix Element"=0.06989063763962523}, {"Real Matrix Element"=-0.8387331176711392, "Real Matrix Element"=0.04485046211030503}, {"Real Matrix Element"=-0.7318516118686567, "Real Matrix Element"=0.026406791167759267}, {"Real Matrix Element"=-0.8480659557785475, "Real Matrix Element"=0.061731464843775036}, {"Real Matrix Element"=-0.6770552586075285, "Real Matrix Element"=0.05187691539196896}, {"Real Matrix Element"=-0.6994004616241641, "Real Matrix Element"=0.06136042379904781}, {"Real Matrix Element"=-0.6967062763343094, "Real Matrix Element"=0.058563219475802335}, {"Real Matrix Element"=-0.463149442300336, "Real Matrix Element"=0.01713503713388993}, {"Real Matrix Element"=-0.35726900546629, "Real Matrix Element"=0.019815241143033777}, {"Real Matrix Element"=-0.018862551695274957, "Real Matrix Element"=-0.06202520189795914}, {"Real Matrix Element"=-0.020517769781202226, "Real Matrix Element"=-0.01891428869316744}, {"Real Matrix Element"=0.078810434439213, "Real Matrix Element"=-0.031175250157681987}, {"Real Matrix Element"=0.2063444357410291, "Real Matrix Element"=-0.025990685359527466}, {"Real Matrix Element"=0.30479237425274236, "Real Matrix Element"=-0.05171233622907592}, {"Real Matrix Element"=0.4339500399666366, "Real Matrix Element"=-0.09064283270125525}, {"Real Matrix Element"=0.5017751419070374, "Real Matrix Element"=-0.08503516608652088}, {"Real Matrix Element"=0.6047586866272789, "Real Matrix Element"=-0.09560922561146608}, {"Real Matrix Element"=0.6657775070641999, "Real Matrix Element"=-0.12642964451958372}, {"Real Matrix Element"=0.6202352086416381, "Real Matrix Element"=-0.09654516433195423}, {"Real Matrix Element"=0.890836417452683, "Real Matrix Element"=-0.1384304477696741}, {"Real Matrix Element"=0.8611615725310442, "Real Matrix Element"=-0.052863877649014866}, {"Real Matrix Element"=0.9706434944306814, "Real Matrix Element"=-0.02109440056917375}, {"Real Matrix Element"=0.8631225986166146, "Real Matrix Element"=0.007339526493731156}, {"Real Matrix Element"=1.0816789874191082, "Real Matrix Element"=0.1109691545875745}, {"Real Matrix Element"=1.0752890533308783, "Real Matrix Element"=0.07798841343832194}, {"Real Matrix Element"=1.420182668935363, "Real Matrix Element"=0.16736997636363582}, {"Real Matrix Element"=1.386405653481829, "Real Matrix Element"=0.14385711667477258}, {"Real Matrix Element"=1.36319237296584, "Real Matrix Element"=0.14382812400731695}, {"Real Matrix Element"=1.901377077263778, "Real Matrix Element"=0.2648051293155056}, {"Real Matrix Element"=2.0499959473429867, "Real Matrix Element"=0.2947676073731155}, {"Real Matrix Element"=1.8316021705500176, "Real Matrix Element"=0.25729715460068053}, {"Real Matrix Element"=2.1778676148333997, "Real Matrix Element"=0.31756581456269495}, {"Real Matrix Element"=2.1600501584958103, "Real Matrix Element"=0.2896637144876541}, {"Real Matrix Element"=2.127115344223501, "Real Matrix Element"=0.22946596478416853}, {"Real Matrix Element"=2.347101416910192, "Real Matrix Element"=0.21069723503525264}, {"Real Matrix Element"=2.469053623519875, "Real Matrix Element"=0.23061809350391585}, {"Real Matrix Element"=2.472967821925176, "Real Matrix Element"=0.19994940214351445}, {"Real Matrix Element"=2.6148350756107517, "Real Matrix Element"=0.19728405242349548}, {"Real Matrix Element"=2.818511949785148, "Real Matrix Element"=0.2458075468347936}, {"Real Matrix Element"=2.9072252723430028, "Real Matrix Element"=0.34495616671928536}, {"Real Matrix Element"=2.859596162896839, "Real Matrix Element"=0.307029461238684}, {"Real Matrix Element"=3.0932460104369928, "Real Matrix Element"=0.3008900564151603}, {"Real Matrix Element"=3.2154374928376352, "Real Matrix Element"=0.3205018947875342}, {"Real Matrix Element"=3.1526126009628084, "Real Matrix Element"=0.38211258545747007}, {"Real Matrix Element"=3.5061680298126, "Real Matrix Element"=0.44506011648354793}, {"Real Matrix Element"=3.48631157597981, "Real Matrix Element"=0.36114760867738854}, {"Real Matrix Element"=3.6217337141026715, "Real Matrix Element"=0.42343200463058195}, {"Real Matrix Element"=3.705495246244265, "Real Matrix Element"=0.43646375871677967}, {"Real Matrix Element"=3.8594877623084347, "Real Matrix Element"=0.4505030387797332}, {"Real Matrix Element"=3.831298834135413, "Real Matrix Element"=0.4889051860977936}, {"Real Matrix Element"=3.786115731865928, "Real Matrix Element"=0.5108908538145228}, {"Real Matrix Element"=3.9232879075954123, "Real Matrix Element"=0.5356004624306598}, {"Real Matrix Element"=3.9273227106281703, "Real Matrix Element"=0.5462811732078747}, {"Real Matrix Element"=4.14287847849307, "Real Matrix Element"=0.6744878913018975}, {"Real Matrix Element"=4.359523849485221, "Real Matrix Element"=0.798096798858485}, {"Real Matrix Element"=4.269934264515053, "Real Matrix Element"=0.7612594083997133}, {"Real Matrix Element"=4.2185050545217795, "Real Matrix Element"=0.8019553046111364}, {"Real Matrix Element"=4.317508455509712, "Real Matrix Element"=0.9216709447046861}, {"Real Matrix Element"=4.497895382104288, "Real Matrix Element"=0.9936051380823888}, {"Real Matrix Element"=4.649824781624764, "Real Matrix Element"=1.2213647724893422}, {"Real Matrix Element"=4.605884088580395, "Real Matrix Element"=1.227447103696051}, {"Real Matrix Element"=4.657024643645219, "Real Matrix Element"=1.3429408942288545}, {"Real Matrix Element"=4.695468966766193, "Real Matrix Element"=1.2819472391589615}, {"Real Matrix Element"=4.828902620347267, "Real Matrix Element"=1.28361041015122}, {"Real Matrix Element"=5.246351414165038, "Real Matrix Element"=1.3773379820702805}, {"Real Matrix Element"=5.2196597598346015, "Real Matrix Element"=1.4009702364098822}, {"Real Matrix Element"=5.209587951358343, "Real Matrix Element"=1.2996644024280517}, {"Real Matrix Element"=5.340982039345069, "Real Matrix Element"=1.6648925442112832}, {"Real Matrix Element"=5.30481730866645, "Real Matrix Element"=1.631413341112202}, {"Real Matrix Element"=5.4392975944673045, "Real Matrix Element"=1.77910499536639}, {"Real Matrix Element"=5.449715604007051, "Real Matrix Element"=1.7009799458169295}, {"Real Matrix Element"=5.521580783863512, "Real Matrix Element"=1.7231047523326355}, {"Real Matrix Element"=5.7488778104727745, "Real Matrix Element"=1.8423565607655987}, {"Real Matrix Element"=5.973197033856639, "Real Matrix Element"=1.875434582271313}, {"Real Matrix Element"=5.959645511277334, "Real Matrix Element"=1.8973710635691865}, {"Real Matrix Element"=6.154868457241486, "Real Matrix Element"=1.9952594485763988}, {"Real Matrix Element"=6.151249355882856, "Real Matrix Element"=1.9674928232675808}, {"Real Matrix Element"=6.290333626653814, "Real Matrix Element"=2.1378270587603088}, {"Real Matrix Element"=6.348235493689309, "Real Matrix Element"=2.2628937356279244}, {"Real Matrix Element"=6.322576464066768, "Real Matrix Element"=2.2207780317683943}, {"Real Matrix Element"=6.395481547984261, "Real Matrix Element"=2.320936835383303}, {"Real Matrix Element"=6.530197353030712, "Real Matrix Element"=2.4351520254329486}, {"Real Matrix Element"=6.554224311353989, "Real Matrix Element"=2.4774153392580858}, {"Real Matrix Element"=6.578023131944982, "Real Matrix Element"=2.5395223999666463}, {"Real Matrix Element"=6.616367565211313, "Real Matrix Element"=2.5239670024202794}, {"Real Matrix Element"=6.684693936902913, "Real Matrix Element"=2.5380760575226575}, {"Real Matrix Element"=6.652520937169329, "Real Matrix Element"=2.492158066849897}, {"Real Matrix Element"=6.812106783787717, "Real Matrix Element"=2.6292562492080975}, {"Real Matrix Element"=7.0336497818453525, "Real Matrix Element"=2.8867625703228037}, {"Real Matrix Element"=6.960505634313455, "Real Matrix Element"=2.912206173749329}, {"Real Matrix Element"=7.153284176774176, "Real Matrix Element"=3.0444105705762254}, {"Real Matrix Element"=7.070344080654263, "Real Matrix Element"=2.9566318697069645}, {"Real Matrix Element"=7.073531595513894, "Real Matrix Element"=3.0306956873792514}, {"Real Matrix Element"=7.216266733469173, "Real Matrix Element"=3.1196637592677763}, {"Real Matrix Element"=7.084224810706213, "Real Matrix Element"=3.0437122373886676}, {"Real Matrix Element"=7.371429850969804, "Real Matrix Element"=3.2550958318549523}, {"Real Matrix Element"=7.478787052181694, "Real Matrix Element"=3.2951865663330144}, {"Real Matrix Element"=7.7449848650713715, "Real Matrix Element"=3.458903074012456}, {"Real Matrix Element"=7.636116522302284, "Real Matrix Element"=3.4368116253296894}, {"Real Matrix Element"=7.790723982197722, "Real Matrix Element"=3.5475302623745133}, {"Real Matrix Element"=7.737166685110266, "Real Matrix Element"=3.5501673220863013}, {"Real Matrix Element"=7.806652188813347, "Real Matrix Element"=3.7620215915896305}, {"Real Matrix Element"=7.986100677254747, "Real Matrix Element"=4.05858509421652}, {"Real Matrix Element"=8.011877118534404, "Real Matrix Element"=4.144818754356533}, {"Real Matrix Element"=7.961203701360732, "Real Matrix Element"=4.03411613926865}, {"Real Matrix Element"=7.997963272121903, "Real Matrix Element"=4.201210784536696}, {"Real Matrix Element"=8.039029787303399, "Real Matrix Element"=4.180450125000687}, {"Real Matrix Element"=8.101922438234626, "Real Matrix Element"=4.22784676812608}, {"Real Matrix Element"=8.105243355026337, "Real Matrix Element"=4.238331078394418}, {"Real Matrix Element"=8.187708793366141, "Real Matrix Element"=4.399438351506242}, {"Real Matrix Element"=8.22299835919839, "Real Matrix Element"=4.475479781663413}, {"Real Matrix Element"=8.378034706023717, "Real Matrix Element"=4.60810392142537}, {"Real Matrix Element"=8.46820684498497, "Real Matrix Element"=4.698643960628395}, {"Real Matrix Element"=8.34556392474826, "Real Matrix Element"=4.630719512478485}, {"Real Matrix Element"=8.33374386956588, "Real Matrix Element"=4.659012467791613}, {"Real Matrix Element"=8.604187332372602, "Real Matrix Element"=4.907160200884222}, {"Real Matrix Element"=8.457416677070281, "Real Matrix Element"=4.684101375955797}, {"Real Matrix Element"=8.690456733476566, "Real Matrix Element"=4.902085785367835}, {"Real Matrix Element"=8.720830001755996, "Real Matrix Element"=5.157122435970386}, {"Real Matrix Element"=8.89582462703551, "Real Matrix Element"=5.333705021527724}, {"Real Matrix Element"=8.995852208979377, "Real Matrix Element"=5.199975031361572}, {"Real Matrix Element"=9.025441848115557, "Real Matrix Element"=5.311496039682403}, {"Real Matrix Element"=9.16543530395395, "Real Matrix Element"=5.478043083628443}, {"Real Matrix Element"=9.064399260196199, "Real Matrix Element"=5.7265805494984}, {"Real Matrix Element"=9.037342971314647, "Real Matrix Element"=5.802200642840099}, {"Real Matrix Element"=8.84787758953912, "Real Matrix Element"=5.61091788087624}, {"Real Matrix Element"=9.01499179772259, "Real Matrix Element"=5.892439280287693}, {"Real Matrix Element"=9.006864892420458, "Real Matrix Element"=6.027045867159803}, {"Real Matrix Element"=9.385005252836171, "Real Matrix Element"=6.041794935065768}, {"Real Matrix Element"=9.530871092075161, "Real Matrix Element"=6.2739268007338875}, {"Real Matrix Element"=9.545555091176013, "Real Matrix Element"=6.254189623543784}, {"Real Matrix Element"=9.085924081444134, "Real Matrix Element"=6.329821722536879}, {"Real Matrix Element"=9.060927902992885, "Real Matrix Element"=6.430389012306283}, {"Real Matrix Element"=9.009645248495886, "Real Matrix Element"=6.399489369075351}, {"Real Matrix Element"=9.16938212690825, "Real Matrix Element"=6.506179902284164}, {"Real Matrix Element"=9.167419365784161, "Real Matrix Element"=6.467937034631238}, {"Real Matrix Element"=9.036905673379605, "Real Matrix Element"=6.651190160676676}, {"Real Matrix Element"=9.398590467270887, "Real Matrix Element"=6.90145101385031}, {"Real Matrix Element"=9.480232753341493, "Real Matrix Element"=6.829420894801919}, {"Real Matrix Element"=9.513851606777862, "Real Matrix Element"=7.037623235157222}, {"Real Matrix Element"=9.507779282527904, "Real Matrix Element"=7.037413579268474}, {"Real Matrix Element"=9.55408920261566, "Real Matrix Element"=7.072311363561782}, {"Real Matrix Element"=9.568110974025895, "Real Matrix Element"=7.059791681570048}, {"Real Matrix Element"=9.497684426817477, "Real Matrix Element"=7.390756094145931}, {"Real Matrix Element"=9.595339727890115, "Real Matrix Element"=7.391489619883513}, {"Real Matrix Element"=9.615917835443328, "Real Matrix Element"=7.5587296980654735}, {"Real Matrix Element"=9.635161900194651, "Real Matrix Element"=7.6521629898124415}, {"Real Matrix Element"=9.647681635233113, "Real Matrix Element"=7.844126012024932}, {"Real Matrix Element"=9.661187764066488, "Real Matrix Element"=7.973193073681779}, {"Real Matrix Element"=9.668439442058046, "Real Matrix Element"=7.949438754040896}, {"Real Matrix Element"=9.670585343512977, "Real Matrix Element"=7.8704673314461715}, {"Real Matrix Element"=9.673950519108521, "Real Matrix Element"=8.096761800202238}, {"Real Matrix Element"=9.695794480379451, "Real Matrix Element"=8.171559057287482}, {"Real Matrix Element"=9.810533786068492, "Real Matrix Element"=8.338275416361368}, {"Real Matrix Element"=9.737694121199244, "Real Matrix Element"=8.39451592322194}, {"Real Matrix Element"=9.799810381790959, "Real Matrix Element"=8.568466903444344}, {"Real Matrix Element"=9.732794616328095, "Real Matrix Element"=8.55492635088381}, {"Real Matrix Element"=9.854964182764393, "Real Matrix Element"=8.697752818133946}, {"Real Matrix Element"=10.04580970877778, "Real Matrix Element"=9.065114151665364}, {"Real Matrix Element"=10.023425295389977, "Real Matrix Element"=9.042470922214896}, {"Real Matrix Element"=10.031609539376495, "Real Matrix Element"=9.049676996411623}, {"Real Matrix Element"=10.034712046164104, "Real Matrix Element"=9.089114503662893}, {"Real Matrix Element"=10.176683853248958, "Real Matrix Element"=9.477659795895729}, {"Real Matrix Element"=10.153225517727957, "Real Matrix Element"=9.496264175023581}, {"Real Matrix Element"=10.156376498432559, "Real Matrix Element"=9.500840590045158}, {"Real Matrix Element"=10.215334765900854, "Real Matrix Element"=9.763299251683584}, {"Real Matrix Element"=10.13107693613301, "Real Matrix Element"=9.953384555486274}, {"Real Matrix Element"=10.16565673419323, "Real Matrix Element"=10.126888711026323}, {"Real Matrix Element"=10.157493611730994, "Real Matrix Element"=10.101000197768558}, {"Real Matrix Element"=10.211208383395977, "Real Matrix Element"=10.226782478557624}, {"Real Matrix Element"=10.225532542447555, "Real Matrix Element"=10.138087085891184}, {"Real Matrix Element"=10.190123120590611, "Real Matrix Element"=10.211179480399021}, {"Real Matrix Element"=10.139176745516188, "Real Matrix Element"=10.405087274216287}, {"Real Matrix Element"=10.076044034336979, "Real Matrix Element"=10.625673589342489}, {"Real Matrix Element"=10.110947458352653, "Real Matrix Element"=10.54442248687473}, {"Real Matrix Element"=10.047700733962246, "Real Matrix Element"=10.716548400816365}, {"Real Matrix Element"=10.0847980628698, "Real Matrix Element"=10.691402785094553}, {"Real Matrix Element"=10.055931465540297, "Real Matrix Element"=10.839742335277798}, {"Real Matrix Element"=10.076446010600424, "Real Matrix Element"=10.869814782252755}, {"Real Matrix Element"=10.066480732128213, "Real Matrix Element"=11.086195225309392}, {"Real Matrix Element"=10.00571636179211, "Real Matrix Element"=11.192052584568922}, {"Real Matrix Element"=10.040603367168627, "Real Matrix Element"=11.207345128773174}, {"Real Matrix Element"=9.990214518934115, "Real Matrix Element"=11.47239536550801}, {"Real Matrix Element"=9.962827052575943, "Real Matrix Element"=11.565594572485185}, {"Real Matrix Element"=9.953680216241205, "Real Matrix Element"=11.635564943724402}, {"Real Matrix Element"=9.920218888854672, "Real Matrix Element"=11.549639878121505}, {"Real Matrix Element"=9.85425158136896, "Real Matrix Element"=11.79041574467308}, {"Real Matrix Element"=9.858815204798137, "Real Matrix Element"=11.776817215071961}, {"Real Matrix Element"=9.83662586938727, "Real Matrix Element"=11.924354337683297}, {"Real Matrix Element"=9.770803075776131, "Real Matrix Element"=12.046019539202069}, {"Real Matrix Element"=9.715780589156635, "Real Matrix Element"=12.238076148801614}, {"Real Matrix Element"=9.736679985405164, "Real Matrix Element"=12.19695078489821}, {"Real Matrix Element"=9.70171412652014, "Real Matrix Element"=12.32514632488217}, {"Real Matrix Element"=9.694715916066075, "Real Matrix Element"=12.445966894108171}, {"Real Matrix Element"=9.662510862752372, "Real Matrix Element"=12.392747427472036}, {"Real Matrix Element"=9.65522744598126, "Real Matrix Element"=12.411074891934959}, {"Real Matrix Element"=9.714408624840312, "Real Matrix Element"=12.657616573800755}, {"Real Matrix Element"=9.565952807766715, "Real Matrix Element"=12.858663658635223}, {"Real Matrix Element"=9.570532350037702, "Real Matrix Element"=12.776122543960495}, {"Real Matrix Element"=9.536180612440045, "Real Matrix Element"=13.036339998773151}, {"Real Matrix Element"=9.580644879561971, "Real Matrix Element"=13.106572614344287}, {"Real Matrix Element"=9.524116249371303, "Real Matrix Element"=13.07830820122902}, {"Real Matrix Element"=9.489851517183169, "Real Matrix Element"=13.281482795790884}, {"Real Matrix Element"=9.413868256110238, "Real Matrix Element"=13.254049364118334}, {"Real Matrix Element"=9.390035444101105, "Real Matrix Element"=13.361614792950231}, {"Real Matrix Element"=9.36458056443312, "Real Matrix Element"=13.428433900769058}, {"Real Matrix Element"=9.389686480405889, "Real Matrix Element"=13.510499990638365}, {"Real Matrix Element"=9.349103262946539, "Real Matrix Element"=13.757907273506245}, {"Real Matrix Element"=9.37062142114718, "Real Matrix Element"=13.750663973901586}, {"Real Matrix Element"=9.391697362374186, "Real Matrix Element"=13.756960347450997}, {"Real Matrix Element"=9.359952967460648, "Real Matrix Element"=13.95220677443584}, {"Real Matrix Element"=9.352107674847453, "Real Matrix Element"=14.12219297882027}, {"Real Matrix Element"=9.323125841290782, "Real Matrix Element"=14.216012363410467}, {"Real Matrix Element"=9.195434806469493, "Real Matrix Element"=14.435486035520189}, {"Real Matrix Element"=9.112957479485358, "Real Matrix Element"=14.554022731800057}, {"Real Matrix Element"=9.084403030766035, "Real Matrix Element"=14.657617240467646}, {"Real Matrix Element"=9.04119660796903, "Real Matrix Element"=14.629436808695447}, {"Real Matrix Element"=9.118871471050209, "Real Matrix Element"=14.485359365870318}, {"Real Matrix Element"=8.95605654638763, "Real Matrix Element"=14.760195779760181}, {"Real Matrix Element"=8.9130521080895, "Real Matrix Element"=14.939528192688671}, {"Real Matrix Element"=8.880777910645952, "Real Matrix Element"=14.933122644995171}, {"Real Matrix Element"=8.657252919272286, "Real Matrix Element"=15.120837385708302}, {"Real Matrix Element"=8.64940339844664, "Real Matrix Element"=15.058405118044385}, {"Real Matrix Element"=8.535114815280675, "Real Matrix Element"=15.115802033476875}, {"Real Matrix Element"=8.553971740987528, "Real Matrix Element"=15.119411215974045}, {"Real Matrix Element"=8.55017952317347, "Real Matrix Element"=15.48832976317972}, {"Real Matrix Element"=8.538205801442002, "Real Matrix Element"=15.577533660329712}, {"Real Matrix Element"=8.461785465771806, "Real Matrix Element"=15.677656358174998}, {"Real Matrix Element"=8.339752961005733, "Real Matrix Element"=15.828857289222427}, {"Real Matrix Element"=8.25072012858703, "Real Matrix Element"=15.831410589914892}, {"Real Matrix Element"=8.250181012103656, "Real Matrix Element"=15.805041769600972}, {"Real Matrix Element"=8.2037753060873, "Real Matrix Element"=15.831804556053012}, {"Real Matrix Element"=8.135268437391254, "Real Matrix Element"=15.838199579491643}, {"Real Matrix Element"=8.073926475332764, "Real Matrix Element"=16.011066123148805}, {"Real Matrix Element"=8.076244376659307, "Real Matrix Element"=15.979161433229487}, {"Real Matrix Element"=7.9769491307321685, "Real Matrix Element"=16.24543020867896}, {"Real Matrix Element"=7.827600830678277, "Real Matrix Element"=16.40071599987466}, {"Real Matrix Element"=7.926880121088491, "Real Matrix Element"=16.209108367300622}, {"Real Matrix Element"=7.777875469697808, "Real Matrix Element"=16.3595413922502}, {"Real Matrix Element"=7.727193371941798, "Real Matrix Element"=16.404483611843265}, {"Real Matrix Element"=7.5958997180989, "Real Matrix Element"=16.52283099782179}, {"Real Matrix Element"=7.602274495673746, "Real Matrix Element"=16.526373358808147}, {"Real Matrix Element"=7.430296085696809, "Real Matrix Element"=16.675417189314516}, {"Real Matrix Element"=7.3489010119961105, "Real Matrix Element"=16.791727014053816}, {"Real Matrix Element"=7.370456777767877, "Real Matrix Element"=16.84327828012353}, {"Real Matrix Element"=7.246053402709181, "Real Matrix Element"=16.86221321919333}, {"Real Matrix Element"=7.212309244027712, "Real Matrix Element"=16.913987916339032}, {"Real Matrix Element"=7.104284278346356, "Real Matrix Element"=17.00257371116475}, {"Real Matrix Element"=6.993213966782519, "Real Matrix Element"=17.05291070278489}, {"Real Matrix Element"=6.937874527599412, "Real Matrix Element"=17.111984127977603}, {"Real Matrix Element"=6.77112322633132, "Real Matrix Element"=17.229811430579087}, {"Real Matrix Element"=6.846007176124099, "Real Matrix Element"=17.314735198496262}, {"Real Matrix Element"=6.7696431044977095, "Real Matrix Element"=17.39009223350552}, {"Real Matrix Element"=6.644831529836419, "Real Matrix Element"=17.485128731014722}, {"Real Matrix Element"=6.515531468619004, "Real Matrix Element"=17.572394026584362}, {"Real Matrix Element"=6.6036266950456515, "Real Matrix Element"=17.511456411627407}, {"Real Matrix Element"=6.412793237399653, "Real Matrix Element"=17.638041329345512}, {"Real Matrix Element"=6.4230311372150135, "Real Matrix Element"=17.634941525850458}, {"Real Matrix Element"=6.241724477353788, "Real Matrix Element"=17.76198878008885}, {"Real Matrix Element"=6.051005356497278, "Real Matrix Element"=17.9479184554995}, {"Real Matrix Element"=6.159422625936549, "Real Matrix Element"=17.887227837432594}, {"Real Matrix Element"=6.0476863011064586, "Real Matrix Element"=17.929251729683543}, {"Real Matrix Element"=6.082855378239043, "Real Matrix Element"=17.97732594844851}, {"Real Matrix Element"=5.900358329777791, "Real Matrix Element"=18.094685409166612}, {"Real Matrix Element"=5.766551612543064, "Real Matrix Element"=18.199307778429343}, {"Real Matrix Element"=5.726668691522898, "Real Matrix Element"=18.270742180878035}, {"Real Matrix Element"=5.657663377114256, "Real Matrix Element"=18.349140807846698}, {"Real Matrix Element"=5.443177003251751, "Real Matrix Element"=18.473461456211375}, {"Real Matrix Element"=5.368188947618676, "Real Matrix Element"=18.543990716826126}, {"Real Matrix Element"=5.467740261124743, "Real Matrix Element"=18.42906555951827}, {"Real Matrix Element"=5.178215357397653, "Real Matrix Element"=18.66043486991587}, {"Real Matrix Element"=5.264249536982099, "Real Matrix Element"=18.562953257066294}, {"Real Matrix Element"=5.090858432883762, "Real Matrix Element"=18.725349263219723}, {"Real Matrix Element"=5.189410033537606, "Real Matrix Element"=18.67060189932878}, {"Real Matrix Element"=5.172945534436973, "Real Matrix Element"=18.660052713970927}, {"Real Matrix Element"=4.812997374090412, "Real Matrix Element"=18.918950665524036}, {"Real Matrix Element"=4.734454786781033, "Real Matrix Element"=18.926641271228526}, {"Real Matrix Element"=4.756338385615206, "Real Matrix Element"=18.88352256586228}, {"Real Matrix Element"=4.701901053051475, "Real Matrix Element"=18.923292355630924}, {"Real Matrix Element"=4.446869430316737, "Real Matrix Element"=19.029258930410897}, {"Real Matrix Element"=4.402330903706256, "Real Matrix Element"=18.952587566314833}, {"Real Matrix Element"=4.283856580194994, "Real Matrix Element"=19.00984415548166}, {"Real Matrix Element"=4.210986170064335, "Real Matrix Element"=19.00413895468584}, {"Real Matrix Element"=4.13098774757933, "Real Matrix Element"=18.994157310837842}, {"Real Matrix Element"=3.977080260799407, "Real Matrix Element"=19.036680624612796}, {"Real Matrix Element"=4.013795168454562, "Real Matrix Element"=19.047877389210605}, {"Real Matrix Element"=3.6915300183418234, "Real Matrix Element"=19.078478396195454}, {"Real Matrix Element"=3.7462818018857824, "Real Matrix Element"=19.09199959967914}, {"Real Matrix Element"=3.6363032223612826, "Real Matrix Element"=19.205094098289997}, {"Real Matrix Element"=3.65729364676608, "Real Matrix Element"=19.16179591226212}, {"Real Matrix Element"=3.585787318916145, "Real Matrix Element"=19.270921319912564}, {"Real Matrix Element"=3.3866350416979554, "Real Matrix Element"=19.293876523313184}, {"Real Matrix Element"=3.368323396671493, "Real Matrix Element"=19.329566585325036}, {"Real Matrix Element"=3.232954456081798, "Real Matrix Element"=19.385502401118114}, {"Real Matrix Element"=3.1192788872844823, "Real Matrix Element"=19.46042942233144}, {"Real Matrix Element"=3.0701337232985306, "Real Matrix Element"=19.52759680155863}, {"Real Matrix Element"=2.9711446387457006, "Real Matrix Element"=19.56612014336654}, {"Real Matrix Element"=2.8792215196651507, "Real Matrix Element"=19.637026031930983}, {"Real Matrix Element"=2.79473265471474, "Real Matrix Element"=19.67577312945314}, {"Real Matrix Element"=2.6807725512306537, "Real Matrix Element"=19.643230949341064}, {"Real Matrix Element"=2.6271299816820752, "Real Matrix Element"=19.709433959408162}, {"Real Matrix Element"=2.6229130151876174, "Real Matrix Element"=19.700277021086052}, {"Real Matrix Element"=2.4591610958915577, "Real Matrix Element"=19.698225129998036}, {"Real Matrix Element"=2.3303674845459508, "Real Matrix Element"=19.737800059416447}, {"Real Matrix Element"=2.437744800169993, "Real Matrix Element"=19.716809189969865}, {"Real Matrix Element"=2.34422464137074, "Real Matrix Element"=19.707454050733798}, {"Real Matrix Element"=2.1377850788806714, "Real Matrix Element"=19.689313477219226}, {"Real Matrix Element"=1.6941705575750539, "Real Matrix Element"=19.71708150437458}, {"Real Matrix Element"=1.5750711697178004, "Real Matrix Element"=19.74661729399427}, {"Real Matrix Element"=1.65336233046077, "Real Matrix Element"=19.725489436324935}, {"Real Matrix Element"=1.6586673614253589, "Real Matrix Element"=19.73668346487463}, {"Real Matrix Element"=1.2164861157415088, "Real Matrix Element"=19.81930415149781}, {"Real Matrix Element"=1.297322544631022, "Real Matrix Element"=19.86537653267215}, {"Real Matrix Element"=1.0586081508202092, "Real Matrix Element"=19.954521722222864}, {"Real Matrix Element"=1.235345631776539, "Real Matrix Element"=19.93900555338125}, {"Real Matrix Element"=0.99901901977108, "Real Matrix Element"=19.97215241151789}, {"Real Matrix Element"=0.7705801729061066, "Real Matrix Element"=19.884924769450798}, {"Real Matrix Element"=0.774002929220503, "Real Matrix Element"=19.960302700580055}, {"Real Matrix Element"=0.7908587406508215, "Real Matrix Element"=19.972298348741315}, {"Real Matrix Element"=0.7388160088667297, "Real Matrix Element"=19.96657319409759}, {"Real Matrix Element"=0.6633185690829392, "Real Matrix Element"=19.94417227125666}, {"Real Matrix Element"=0.5050190917112496, "Real Matrix Element"=19.97806608280855}, {"Real Matrix Element"=0.569748226423683, "Real Matrix Element"=19.949658349668727}, {"Real Matrix Element"=0.23641420741684055, "Real Matrix Element"=19.919003136714142}, {"Real Matrix Element"=-0.03360664871020329, "Real Matrix Element"=19.90779427036137}, {"Real Matrix Element"=-0.0463920506290849, "Real Matrix Element"=19.895163746914715}, {"Real Matrix Element"=-0.04274712769146437, "Real Matrix Element"=19.89640885504025}, {"Real Matrix Element"=-0.208711316077694, "Real Matrix Element"=19.912722536875236}, {"Real Matrix Element"=-0.3145891536513091, "Real Matrix Element"=19.943999995533126}, {"Real Matrix Element"=-0.32444244540449313, "Real Matrix Element"=19.962179077599803}, {"Real Matrix Element"=-0.28371498759705716, "Real Matrix Element"=19.97168195286686}, {"Real Matrix Element"=-0.46607183548132397, "Real Matrix Element"=19.932916257011392}, {"Real Matrix Element"=-0.6300266952578559, "Real Matrix Element"=20.050293555685844}, {"Real Matrix Element"=-0.6996201409624847, "Real Matrix Element"=20.077594347417094}, {"Real Matrix Element"=-0.8330239514419594, "Real Matrix Element"=20.020220201701573}, {"Real Matrix Element"=-0.7070351427993969, "Real Matrix Element"=19.994261061846107}, {"Real Matrix Element"=-0.9324591025991544, "Real Matrix Element"=20.040832629702678}, {"Real Matrix Element"=-1.2014768777707545, "Real Matrix Element"=20.001641280297218}, {"Real Matrix Element"=-1.171969115984433, "Real Matrix Element"=19.970737119433153}, {"Real Matrix Element"=-1.1491247632147983, "Real Matrix Element"=19.99852655773894}, {"Real Matrix Element"=-1.270052736926906, "Real Matrix Element"=20.005144399877704}, {"Real Matrix Element"=-1.4527437223635318, "Real Matrix Element"=19.99876073378097}, {"Real Matrix Element"=-1.4836381056116044, "Real Matrix Element"=19.980298429785176}, {"Real Matrix Element"=-1.5975964335596975, "Real Matrix Element"=19.989258750481753}, {"Real Matrix Element"=-1.7820196339704715, "Real Matrix Element"=19.87029893569233}, {"Real Matrix Element"=-1.8632147509125563, "Real Matrix Element"=19.825922028993293}, {"Real Matrix Element"=-2.114303634945072, "Real Matrix Element"=19.807553031177623}, {"Real Matrix Element"=-2.0666634432514055, "Real Matrix Element"=19.81669428141548}, {"Real Matrix Element"=-2.21762262863997, "Real Matrix Element"=19.8166610056586}, {"Real Matrix Element"=-2.1666579168062294, "Real Matrix Element"=19.804512602736825}, {"Real Matrix Element"=-2.2481756867509426, "Real Matrix Element"=19.77537815591074}, {"Real Matrix Element"=-2.263009189794852, "Real Matrix Element"=19.801996228550763}, {"Real Matrix Element"=-2.4673504327671343, "Real Matrix Element"=19.723677595762823}, {"Real Matrix Element"=-2.5232305344513013, "Real Matrix Element"=19.688933779189338}, {"Real Matrix Element"=-2.4144028723386524, "Real Matrix Element"=19.74535722793795}, {"Real Matrix Element"=-2.8100271514869397, "Real Matrix Element"=19.575180679925868}, {"Real Matrix Element"=-2.862328310527549, "Real Matrix Element"=19.490098836576237}, {"Real Matrix Element"=-3.0537660847964543, "Real Matrix Element"=19.359596063266274}, {"Real Matrix Element"=-3.070630950729245, "Real Matrix Element"=19.38788598637505}, {"Real Matrix Element"=-3.3733499727511247, "Real Matrix Element"=19.219849320903993}, {"Real Matrix Element"=-3.3029422632051575, "Real Matrix Element"=19.236803549708373}, {"Real Matrix Element"=-3.4753307668877924, "Real Matrix Element"=19.139849166973374}, {"Real Matrix Element"=-3.5565768928938533, "Real Matrix Element"=19.062812944944998}, {"Real Matrix Element"=-3.644572139664749, "Real Matrix Element"=19.01320496220404}, {"Real Matrix Element"=-3.804060922390485, "Real Matrix Element"=18.913980791554067}, {"Real Matrix Element"=-3.8354390751688094, "Real Matrix Element"=18.83952587542442}, {"Real Matrix Element"=-3.932680416374816, "Real Matrix Element"=18.82176422327245}, {"Real Matrix Element"=-4.151521518412326, "Real Matrix Element"=18.816125410797007}, {"Real Matrix Element"=-4.201798897355065, "Real Matrix Element"=18.75211271228031}, {"Real Matrix Element"=-4.503817499161698, "Real Matrix Element"=18.80189867054168}, {"Real Matrix Element"=-4.32334478144657, "Real Matrix Element"=18.920101026081323}, {"Real Matrix Element"=-4.372137421002963, "Real Matrix Element"=18.9563476207334}, {"Real Matrix Element"=-4.602936381573318, "Real Matrix Element"=18.865906777543756}, {"Real Matrix Element"=-4.476183398540397, "Real Matrix Element"=18.911305316973205}, {"Real Matrix Element"=-4.48919001501171, "Real Matrix Element"=18.90933574120923}, {"Real Matrix Element"=-4.642243988312725, "Real Matrix Element"=18.835956074942793}, {"Real Matrix Element"=-4.836710403616123, "Real Matrix Element"=18.704184360820477}, {"Real Matrix Element"=-4.873165530661675, "Real Matrix Element"=18.698844777741087}, {"Real Matrix Element"=-5.022740498937969, "Real Matrix Element"=18.642480332526635}, {"Real Matrix Element"=-5.037910539531527, "Real Matrix Element"=18.55677832064859}, {"Real Matrix Element"=-5.010441372870882, "Real Matrix Element"=18.614446888412175}, {"Real Matrix Element"=-5.206133246888482, "Real Matrix Element"=18.519385419723072}, {"Real Matrix Element"=-5.425953738557817, "Real Matrix Element"=18.467262555649157}, {"Real Matrix Element"=-5.467041704524981, "Real Matrix Element"=18.43178402769134}, {"Real Matrix Element"=-5.488464330436733, "Real Matrix Element"=18.450022767593854}, {"Real Matrix Element"=-5.431304787920068, "Real Matrix Element"=18.460088745097128}, {"Real Matrix Element"=-5.5156125582552695, "Real Matrix Element"=18.393481601556633}, {"Real Matrix Element"=-5.6928976049715345, "Real Matrix Element"=18.300485951733798}, {"Real Matrix Element"=-5.599693718932936, "Real Matrix Element"=18.329813580862865}, {"Real Matrix Element"=-5.792516352996589, "Real Matrix Element"=18.20719817098942}, {"Real Matrix Element"=-5.905286388210416, "Real Matrix Element"=18.048290988165068}, {"Real Matrix Element"=-6.165339554833317, "Real Matrix Element"=17.79948057305406}, {"Real Matrix Element"=-6.147817977937764, "Real Matrix Element"=17.819698275384585}, {"Real Matrix Element"=-6.193917857863027, "Real Matrix Element"=17.706928028727663}, {"Real Matrix Element"=-6.282098610343407, "Real Matrix Element"=17.590406051329254}, {"Real Matrix Element"=-6.174097547741047, "Real Matrix Element"=17.662948056020323}, {"Real Matrix Element"=-6.323786545073036, "Real Matrix Element"=17.51653812395365}, {"Real Matrix Element"=-6.474762478760597, "Real Matrix Element"=17.369009223762735}, {"Real Matrix Element"=-6.4913576239756745, "Real Matrix Element"=17.30939744649333}, {"Real Matrix Element"=-6.492742242820168, "Real Matrix Element"=17.34793168210304}, {"Real Matrix Element"=-6.989258387352259, "Real Matrix Element"=17.089352341794253}, {"Real Matrix Element"=-7.028805953947648, "Real Matrix Element"=17.080466194240973}, {"Real Matrix Element"=-7.001555678953996, "Real Matrix Element"=17.104895704118025}, {"Real Matrix Element"=-7.057714981746209, "Real Matrix Element"=17.086450840633592}, {"Real Matrix Element"=-6.90353802060849, "Real Matrix Element"=17.171588049164676}, {"Real Matrix Element"=-7.137814167036626, "Real Matrix Element"=17.05392414240027}, {"Real Matrix Element"=-7.139685972071022, "Real Matrix Element"=17.034063203012526}, {"Real Matrix Element"=-7.26523163758515, "Real Matrix Element"=16.965445245156026}, {"Real Matrix Element"=-7.181929562600727, "Real Matrix Element"=17.015407833174507}, {"Real Matrix Element"=-7.281860309916006, "Real Matrix Element"=16.949017050471983}, {"Real Matrix Element"=-7.478015136736144, "Real Matrix Element"=16.795038293914025}, {"Real Matrix Element"=-7.5079130815075255, "Real Matrix Element"=16.737716141258364}, {"Real Matrix Element"=-7.599346237297007, "Real Matrix Element"=16.637596190796465}, {"Real Matrix Element"=-7.6358331862225235, "Real Matrix Element"=16.5705250290947}, {"Real Matrix Element"=-7.833945715682453, "Real Matrix Element"=16.311763656680263}, {"Real Matrix Element"=-7.897448173497947, "Real Matrix Element"=16.257336779225458}, {"Real Matrix Element"=-7.84215968044275, "Real Matrix Element"=16.32800847420927}, {"Real Matrix Element"=-7.865976079757685, "Real Matrix Element"=16.248241838019986}, {"Real Matrix Element"=-7.8690575404357315, "Real Matrix Element"=16.15263400139316}, {"Real Matrix Element"=-7.9796645083198925, "Real Matrix Element"=16.096708787606516}, {"Real Matrix Element"=-7.999204619826109, "Real Matrix Element"=16.00004260606954}, {"Real Matrix Element"=-8.06642456906802, "Real Matrix Element"=15.947827878053944}, {"Real Matrix Element"=-8.267055212068675, "Real Matrix Element"=15.584996893829008}, {"Real Matrix Element"=-8.424986966391206, "Real Matrix Element"=15.471313185830008}, {"Real Matrix Element"=-8.359237755743774, "Real Matrix Element"=15.558367210702189}, {"Real Matrix Element"=-8.457689733945282, "Real Matrix Element"=15.366367472842821}, {"Real Matrix Element"=-8.44552747069262, "Real Matrix Element"=15.386715857471971}, {"Real Matrix Element"=-8.494638593344062, "Real Matrix Element"=15.361790796005714}, {"Real Matrix Element"=-8.488442824382352, "Real Matrix Element"=15.383211394051102}, {"Real Matrix Element"=-8.588607146523888, "Real Matrix Element"=15.12290554796981}, {"Real Matrix Element"=-8.707172009513558, "Real Matrix Element"=14.991008004248993}, {"Real Matrix Element"=-8.67751919197885, "Real Matrix Element"=15.017033840565174}, {"Real Matrix Element"=-8.774743418880682, "Real Matrix Element"=14.887323320758904}, {"Real Matrix Element"=-8.746598752207024, "Real Matrix Element"=14.759835919224706}, {"Real Matrix Element"=-8.709967977321512, "Real Matrix Element"=14.756936466732784}, {"Real Matrix Element"=-8.73675644699182, "Real Matrix Element"=14.68069340710222}, {"Real Matrix Element"=-8.98290580703087, "Real Matrix Element"=14.36096667058768}, {"Real Matrix Element"=-9.05383950501643, "Real Matrix Element"=14.271301256704684}, {"Real Matrix Element"=-8.992739039945441, "Real Matrix Element"=14.306911657562948}, {"Real Matrix Element"=-9.1467950128603, "Real Matrix Element"=14.048113497356304}, {"Real Matrix Element"=-9.18079387522726, "Real Matrix Element"=13.978395590019007}, {"Real Matrix Element"=-9.2331255108197, "Real Matrix Element"=13.7504989358109}, {"Real Matrix Element"=-9.224400755680769, "Real Matrix Element"=13.78067292179773}, {"Real Matrix Element"=-9.183864588583807, "Real Matrix Element"=13.854809837188766}, {"Real Matrix Element"=-9.128129739317748, "Real Matrix Element"=13.966323772461257}, {"Real Matrix Element"=-9.209477675706896, "Real Matrix Element"=13.856351877357344}, {"Real Matrix Element"=-9.268402676372046, "Real Matrix Element"=13.727906453712624}, {"Real Matrix Element"=-9.321841873046095, "Real Matrix Element"=13.66169276301748}, {"Real Matrix Element"=-9.368288097206817, "Real Matrix Element"=13.582616225546138}, {"Real Matrix Element"=-9.403923804010793, "Real Matrix Element"=13.47351917109946}, {"Real Matrix Element"=-9.47694253212317, "Real Matrix Element"=13.238841520773047}, {"Real Matrix Element"=-9.501942045602153, "Real Matrix Element"=13.035942044404521}, {"Real Matrix Element"=-9.488446293924557, "Real Matrix Element"=13.11164219928918}, {"Real Matrix Element"=-9.493262366279913, "Real Matrix Element"=13.125355700727315}, {"Real Matrix Element"=-9.545772924467943, "Real Matrix Element"=12.888235039272733}, {"Real Matrix Element"=-9.556169944258098, "Real Matrix Element"=12.74606808477927}, {"Real Matrix Element"=-9.561993374130902, "Real Matrix Element"=12.586735489916249}, {"Real Matrix Element"=-9.548781006396316, "Real Matrix Element"=12.551787195245776}, {"Real Matrix Element"=-9.595731317233062, "Real Matrix Element"=12.616892376950371}, {"Real Matrix Element"=-9.609073147204723, "Real Matrix Element"=12.514121530912476}, {"Real Matrix Element"=-9.594699454549655, "Real Matrix Element"=12.192160189533254}, {"Real Matrix Element"=-9.616982580333103, "Real Matrix Element"=12.045983328067777}, {"Real Matrix Element"=-9.649645040381921, "Real Matrix Element"=11.96677265206224}, {"Real Matrix Element"=-9.688786368677992, "Real Matrix Element"=11.93807373884613}, {"Real Matrix Element"=-9.718175531939261, "Real Matrix Element"=11.83245804176071}, {"Real Matrix Element"=-9.717049880091993, "Real Matrix Element"=11.83955421340816}, {"Real Matrix Element"=-9.780689351283096, "Real Matrix Element"=11.691301328352896}, {"Real Matrix Element"=-9.871027900426869, "Real Matrix Element"=11.642798218953718}, {"Real Matrix Element"=-9.852784802300846, "Real Matrix Element"=11.59990898124774}, {"Real Matrix Element"=-9.975979463055578, "Real Matrix Element"=11.39296897719755}, {"Real Matrix Element"=-9.953269413672569, "Real Matrix Element"=11.23151913662336}, {"Real Matrix Element"=-10.015388053040283, "Real Matrix Element"=11.164764289729495}, {"Real Matrix Element"=-9.948575963782949, "Real Matrix Element"=11.31195020848033}, {"Real Matrix Element"=-9.914464778518564, "Real Matrix Element"=10.983012825171905}, {"Real Matrix Element"=-10.01052645440373, "Real Matrix Element"=11.057600367073471}, {"Real Matrix Element"=-10.112879698937759, "Real Matrix Element"=10.93326762418633}, {"Real Matrix Element"=-10.192487549482674, "Real Matrix Element"=10.977367164878283}, {"Real Matrix Element"=-10.093806083037547, "Real Matrix Element"=10.823326742125666}, {"Real Matrix Element"=-10.083852706694785, "Real Matrix Element"=10.58656213234937}, {"Real Matrix Element"=-10.05351465104368, "Real Matrix Element"=10.40137767381322}, {"Real Matrix Element"=-10.061055217494175, "Real Matrix Element"=10.238971413576738}, {"Real Matrix Element"=-10.059395958954696, "Real Matrix Element"=10.248805703840151}, {"Real Matrix Element"=-10.030192912241908, "Real Matrix Element"=10.02749390500707}, {"Real Matrix Element"=-10.047495683099948, "Real Matrix Element"=10.228211213808057}, {"Real Matrix Element"=-10.03945962873185, "Real Matrix Element"=9.814777071175323}, {"Real Matrix Element"=-10.049243553397334, "Real Matrix Element"=10.018365902719049}, {"Real Matrix Element"=-10.09472465374756, "Real Matrix Element"=9.784761132278643}, {"Real Matrix Element"=-10.055485026382009, "Real Matrix Element"=9.794052216259496}, {"Real Matrix Element"=-9.964656496863979, "Real Matrix Element"=9.56606421533437}, {"Real Matrix Element"=-9.961464216996019, "Real Matrix Element"=9.399089774596074}, {"Real Matrix Element"=-9.993300308714543, "Real Matrix Element"=9.356075952815836}, {"Real Matrix Element"=-9.925131080302595, "Real Matrix Element"=9.06618776379775}, {"Real Matrix Element"=-9.918695866938652, "Real Matrix Element"=9.125934047275257}, {"Real Matrix Element"=-9.744650130934934, "Real Matrix Element"=8.775485094624898}, {"Real Matrix Element"=-9.689935425940073, "Real Matrix Element"=8.628030162923174}, {"Real Matrix Element"=-9.891810412618948, "Real Matrix Element"=8.91065071980556}, {"Real Matrix Element"=-9.844089341280242, "Real Matrix Element"=8.815900726168612}, {"Real Matrix Element"=-9.688161414716152, "Real Matrix Element"=8.496632854692862}, {"Real Matrix Element"=-9.559128586271095, "Real Matrix Element"=8.352497923273852}, {"Real Matrix Element"=-9.708760047742107, "Real Matrix Element"=8.510294245062548}, {"Real Matrix Element"=-9.750439766675807, "Real Matrix Element"=8.590477325970756}, {"Real Matrix Element"=-9.723451250744384, "Real Matrix Element"=8.207737888069142}, {"Real Matrix Element"=-9.725013776423635, "Real Matrix Element"=8.129893474515596}, {"Real Matrix Element"=-9.77285893048977, "Real Matrix Element"=7.969356618272259}, {"Real Matrix Element"=-9.777392194207097, "Real Matrix Element"=7.87803255021089}, {"Real Matrix Element"=-9.738814903615786, "Real Matrix Element"=7.69499971852915}, {"Real Matrix Element"=-9.746309818921379, "Real Matrix Element"=7.691971149152192}, {"Real Matrix Element"=-9.690359414778182, "Real Matrix Element"=7.494088631547395}, {"Real Matrix Element"=-9.578613912290672, "Real Matrix Element"=7.290215180436431}, {"Real Matrix Element"=-9.540963355590334, "Real Matrix Element"=7.268888268534923}, {"Real Matrix Element"=-9.479492383486605, "Real Matrix Element"=7.219939904559749}, {"Real Matrix Element"=-9.528190966821366, "Real Matrix Element"=7.266972502251751}, {"Real Matrix Element"=-9.59385505392414, "Real Matrix Element"=7.375710469226992}, {"Real Matrix Element"=-9.434073737054089, "Real Matrix Element"=7.051329947354203}, {"Real Matrix Element"=-9.17780673164187, "Real Matrix Element"=6.595226310024634}, {"Real Matrix Element"=-9.162335493845625, "Real Matrix Element"=6.577661415752084}, {"Real Matrix Element"=-9.191899525956366, "Real Matrix Element"=6.651468607093566}, {"Real Matrix Element"=-9.323099908458774, "Real Matrix Element"=6.798396077663155}, {"Real Matrix Element"=-9.360403493075491, "Real Matrix Element"=6.804910751093326}, {"Real Matrix Element"=-9.312799130723546, "Real Matrix Element"=6.592321443241647}, {"Real Matrix Element"=-9.176883698540117, "Real Matrix Element"=6.380393519457769}, {"Real Matrix Element"=-9.135165908380003, "Real Matrix Element"=6.288706375219793}, {"Real Matrix Element"=-9.008569848404534, "Real Matrix Element"=6.087264980972538}, {"Real Matrix Element"=-8.948982517205092, "Real Matrix Element"=5.981924901340226}, {"Real Matrix Element"=-8.974825502512651, "Real Matrix Element"=5.984745065458795}, {"Real Matrix Element"=-9.006539093644363, "Real Matrix Element"=6.027193547401524}, {"Real Matrix Element"=-8.952150000765057, "Real Matrix Element"=5.6553466261982805}, {"Real Matrix Element"=-8.991975102560879, "Real Matrix Element"=5.8141611943197695}, {"Real Matrix Element"=-8.935129973617121, "Real Matrix Element"=5.703084573295303}, {"Real Matrix Element"=-8.747618466927, "Real Matrix Element"=5.340799248016019}, {"Real Matrix Element"=-8.66472452166784, "Real Matrix Element"=5.311256856231637}, {"Real Matrix Element"=-8.76947181313265, "Real Matrix Element"=5.41025473233554}, {"Real Matrix Element"=-8.735061142705705, "Real Matrix Element"=5.219472270583303}, {"Real Matrix Element"=-8.721416845469344, "Real Matrix Element"=5.253601069254292}, {"Real Matrix Element"=-8.75271649149798, "Real Matrix Element"=5.315061750899354}, {"Real Matrix Element"=-8.712579447970024, "Real Matrix Element"=5.271117872848421}, {"Real Matrix Element"=-8.592159635095953, "Real Matrix Element"=4.924694051444345}, {"Real Matrix Element"=-8.585285468389957, "Real Matrix Element"=4.902254442817707}, {"Real Matrix Element"=-8.569825601405986, "Real Matrix Element"=4.864609284447702}, {"Real Matrix Element"=-8.532545932119195, "Real Matrix Element"=4.733856395380565}, {"Real Matrix Element"=-8.431014571561043, "Real Matrix Element"=4.440099257483511}, {"Real Matrix Element"=-8.408824518771294, "Real Matrix Element"=4.422996160098765}, {"Real Matrix Element"=-8.336772499883999, "Real Matrix Element"=4.369551680440586}, {"Real Matrix Element"=-8.283764741100722, "Real Matrix Element"=4.306809505491363}, {"Real Matrix Element"=-8.166875545722982, "Real Matrix Element"=4.181214673763531}, {"Real Matrix Element"=-8.096861389488048, "Real Matrix Element"=4.049507446760605}, {"Real Matrix Element"=-8.050710572245494, "Real Matrix Element"=3.996885225352017}, {"Real Matrix Element"=-8.045915155238903, "Real Matrix Element"=3.9608979458050237}, {"Real Matrix Element"=-7.951591329640788, "Real Matrix Element"=3.8682058026573745}, {"Real Matrix Element"=-7.859464650425699, "Real Matrix Element"=3.823545800108545}, {"Real Matrix Element"=-7.695639695844096, "Real Matrix Element"=3.60798353331431}, {"Real Matrix Element"=-7.6616055301383765, "Real Matrix Element"=3.6905243539807184}, {"Real Matrix Element"=-7.629852135666079, "Real Matrix Element"=3.728523597663263}, {"Real Matrix Element"=-7.474241670304554, "Real Matrix Element"=3.5052113676683723}, {"Real Matrix Element"=-7.462328768658254, "Real Matrix Element"=3.4665893546949706}, {"Real Matrix Element"=-7.474324067417682, "Real Matrix Element"=3.443195831418122}, {"Real Matrix Element"=-7.309979662355666, "Real Matrix Element"=3.2842940445295072}, {"Real Matrix Element"=-7.278401520319894, "Real Matrix Element"=3.3087198002839693}, {"Real Matrix Element"=-7.0912053907628145, "Real Matrix Element"=3.139883261715214}, {"Real Matrix Element"=-7.111904341196526, "Real Matrix Element"=3.117771082933576}, {"Real Matrix Element"=-7.10984270523166, "Real Matrix Element"=3.102967201561775}, {"Real Matrix Element"=-6.910122741059148, "Real Matrix Element"=2.985100923289249}, {"Real Matrix Element"=-6.682620288894481, "Real Matrix Element"=2.7861121033184735}, {"Real Matrix Element"=-6.929837397172074, "Real Matrix Element"=2.9568765007369078}, {"Real Matrix Element"=-6.833345415723629, "Real Matrix Element"=2.8629028973001183}, {"Real Matrix Element"=-6.809788613989425, "Real Matrix Element"=2.8661456052190433}, {"Real Matrix Element"=-6.594071107549028, "Real Matrix Element"=2.6921248403462488}, {"Real Matrix Element"=-6.433786272138008, "Real Matrix Element"=2.550865342289259}, {"Real Matrix Element"=-6.413669900288211, "Real Matrix Element"=2.543191304929715}, {"Real Matrix Element"=-6.451583065388174, "Real Matrix Element"=2.5800791784757573}, {"Real Matrix Element"=-6.218361852301557, "Real Matrix Element"=2.3531672366855174}, {"Real Matrix Element"=-6.189432810873765, "Real Matrix Element"=2.308714211221647}, {"Real Matrix Element"=-6.26486923607859, "Real Matrix Element"=2.3460996789729216}, {"Real Matrix Element"=-6.210464705416754, "Real Matrix Element"=2.291549209778796}, {"Real Matrix Element"=-6.24074833221362, "Real Matrix Element"=2.3147844135824163}, {"Real Matrix Element"=-5.943632791375722, "Real Matrix Element"=2.040264693449921}, {"Real Matrix Element"=-5.829400338746148, "Real Matrix Element"=1.9953597629139244}, {"Real Matrix Element"=-5.7166584354105, "Real Matrix Element"=1.9069832296097302}, {"Real Matrix Element"=-5.6421816479556455, "Real Matrix Element"=1.8419986337598369}, {"Real Matrix Element"=-5.733595652194592, "Real Matrix Element"=1.941034673701249}, {"Real Matrix Element"=-5.5417163346791725, "Real Matrix Element"=1.7929064811662996}, {"Real Matrix Element"=-5.563446113937198, "Real Matrix Element"=1.808762686816973}, {"Real Matrix Element"=-5.396534353520526, "Real Matrix Element"=1.6520763385463517}, {"Real Matrix Element"=-5.198298850941057, "Real Matrix Element"=1.508637603397411}, {"Real Matrix Element"=-5.253309976209384, "Real Matrix Element"=1.555825111641721}, {"Real Matrix Element"=-5.237215206248882, "Real Matrix Element"=1.5722465104477552}, {"Real Matrix Element"=-5.173479881111607, "Real Matrix Element"=1.5479500009075209}, {"Real Matrix Element"=-5.15055236088833, "Real Matrix Element"=1.5496604578635047}, {"Real Matrix Element"=-4.920517440782683, "Real Matrix Element"=1.4533516129504893}, {"Real Matrix Element"=-4.758024570467654, "Real Matrix Element"=1.3544779481515798}, {"Real Matrix Element"=-4.6793872042194, "Real Matrix Element"=1.3005848698723832}, {"Real Matrix Element"=-4.623167791065971, "Real Matrix Element"=1.1988696507053604}, {"Real Matrix Element"=-4.4886469678144865, "Real Matrix Element"=1.1996568675261765}, {"Real Matrix Element"=-4.627704623448605, "Real Matrix Element"=1.2207846674722571}, {"Real Matrix Element"=-4.518690246248496, "Real Matrix Element"=1.1482523220372798}, {"Real Matrix Element"=-4.467325954851071, "Real Matrix Element"=1.1355101142011714}, {"Real Matrix Element"=-4.160848079114981, "Real Matrix Element"=0.9495509038227349}, {"Real Matrix Element"=-3.955013516280184, "Real Matrix Element"=0.943358787413967}, {"Real Matrix Element"=-4.062658102403786, "Real Matrix Element"=0.9235571508937089}, {"Real Matrix Element"=-4.046593649986399, "Real Matrix Element"=0.907937896197378}, {"Real Matrix Element"=-3.953095475805898, "Real Matrix Element"=0.8496074445573033}, {"Real Matrix Element"=-3.730268709421943, "Real Matrix Element"=0.6981852052397058}, {"Real Matrix Element"=-3.4775468771314366, "Real Matrix Element"=0.6330286974503996}, {"Real Matrix Element"=-3.6286556066641857, "Real Matrix Element"=0.6906150437740726}, {"Real Matrix Element"=-3.4828269866581003, "Real Matrix Element"=0.6051548875539672}, {"Real Matrix Element"=-3.370163356408738, "Real Matrix Element"=0.5466465182135332}, {"Real Matrix Element"=-3.281561021428518, "Real Matrix Element"=0.5121989073440176}, {"Real Matrix Element"=-3.181677569406428, "Real Matrix Element"=0.4845688912325016}, {"Real Matrix Element"=-3.168274799261499, "Real Matrix Element"=0.4387477488073718}, {"Real Matrix Element"=-3.0159284214558273, "Real Matrix Element"=0.3847398031930702}, {"Real Matrix Element"=-3.0078767564268265, "Real Matrix Element"=0.4212166825970692}, {"Real Matrix Element"=-2.6359276162201244, "Real Matrix Element"=0.26476993380167624}, {"Real Matrix Element"=-2.57990615400404, "Real Matrix Element"=0.2997513848458314}, {"Real Matrix Element"=-2.623910960162819, "Real Matrix Element"=0.3834694169922049}, {"Real Matrix Element"=-2.6894853297769323, "Real Matrix Element"=0.41995330510649886}, {"Real Matrix Element"=-2.595103864443463, "Real Matrix Element"=0.4132270729202433}, {"Real Matrix Element"=-2.2230699120121264, "Real Matrix Element"=0.24781529336660268}, {"Real Matrix Element"=-2.190674383237053, "Real Matrix Element"=0.1383860831207615}, {"Real Matrix Element"=-2.1106156682617696, "Real Matrix Element"=0.15106254359591795}, {"Real Matrix Element"=-1.9167538201482763, "Real Matrix Element"=0.06149118822238597}, {"Real Matrix Element"=-1.941266378824414, "Real Matrix Element"=0.12110808948308609}, {"Real Matrix Element"=-1.8043382544598456, "Real Matrix Element"=0.15621463204590003}, {"Real Matrix Element"=-1.6219462310567825, "Real Matrix Element"=0.07726863870205906}, {"Real Matrix Element"=-1.3871504596848219, "Real Matrix Element"=-0.001308520472705262}, {"Real Matrix Element"=-1.525270139950925, "Real Matrix Element"=0.03589710228575325}, {"Real Matrix Element"=-1.2692714970399803, "Real Matrix Element"=-0.05482529516145362}, {"Real Matrix Element"=-1.0191024640818365, "Real Matrix Element"=-0.048525247587771804}, {"Real Matrix Element"=-1.2262668698442103, "Real Matrix Element"=-0.03076118457810692}, {"Real Matrix Element"=-1.1727558130402498, "Real Matrix Element"=-0.03189624835585215}, {"Real Matrix Element"=-1.0194769215751267, "Real Matrix Element"=0.07393699138152111}, {"Real Matrix Element"=-1.026946279275472, "Real Matrix Element"=0.017411699647389187}, {"Real Matrix Element"=-0.8652938509394852, "Real Matrix Element"=0.06591268352073265}, {"Real Matrix Element"=-0.8910042247888766, "Real Matrix Element"=0.04305355020157959}, {"Real Matrix Element"=-0.7457607384969562, "Real Matrix Element"=0.09068066134046925}, {"Real Matrix Element"=-0.5580988428924414, "Real Matrix Element"=0.1137450837050803}, {"Real Matrix Element"=-0.6123110079405143, "Real Matrix Element"=0.03787358258815484}, {"Real Matrix Element"=-0.41127532983097936, "Real Matrix Element"=0.05231035260642025}, {"Real Matrix Element"=-0.17804612070570902, "Real Matrix Element"=0.1130189544218284}, {"Real Matrix Element"=0.10948489670094116, "Real Matrix Element"=0.1218077680586402}, {"Real Matrix Element"=0.27473453413535354, "Real Matrix Element"=0.08671512575789803}, {"Real Matrix Element"=0.28359232721081334, "Real Matrix Element"=0.04700656156931428}, {"Real Matrix Element"=0.24717586754693174, "Real Matrix Element"=0.05543362159610545}, {"Real Matrix Element"=0.27097775189195217, "Real Matrix Element"=0.05319634317392857}, {"Real Matrix Element"=0.37138497107487484, "Real Matrix Element"=0.058701508337669205}, {"Real Matrix Element"=0.69972088492577, "Real Matrix Element"=0.053025246669122686}, {"Real Matrix Element"=0.5696903381082261, "Real Matrix Element"=0.04218292786150626}, {"Real Matrix Element"=0.6593412978184934, "Real Matrix Element"=0.016991541280886254}, {"Real Matrix Element"=0.6649301180711227, "Real Matrix Element"=0.017845628209736338}, {"Real Matrix Element"=0.8213085569459039, "Real Matrix Element"=-0.017621281277275563}, {"Real Matrix Element"=0.8399021044211257, "Real Matrix Element"=-0.032579384934981886}, {"Real Matrix Element"=0.953311021494735, "Real Matrix Element"=-0.018886745351736747}, {"Real Matrix Element"=1.2539784155314544, "Real Matrix Element"=-0.028947619577457565}, {"Real Matrix Element"=1.2232115895252655, "Real Matrix Element"=-0.03344941644518303}, {"Real Matrix Element"=1.4137116574014845, "Real Matrix Element"=-0.01790413838871692}, {"Real Matrix Element"=1.4662258597846265, "Real Matrix Element"=-0.0029696748781400254}, {"Real Matrix Element"=1.5958517813716082, "Real Matrix Element"=0.05163263474504268}, {"Real Matrix Element"=1.64666764275189, "Real Matrix Element"=0.09965442824593759}, {"Real Matrix Element"=1.7920761590090273, "Real Matrix Element"=0.1574669482233957}, {"Real Matrix Element"=1.6750442794400031, "Real Matrix Element"=0.13260497044376737}, {"Real Matrix Element"=1.9759706301247961, "Real Matrix Element"=0.14422630874767037}, {"Real Matrix Element"=2.0933555168935976, "Real Matrix Element"=0.1559429791869376}, {"Real Matrix Element"=2.021137221130001, "Real Matrix Element"=0.17158560840060852}, {"Real Matrix Element"=2.348851650866907, "Real Matrix Element"=0.19943812735760746}, {"Real Matrix Element"=2.260363574253451, "Real Matrix Element"=0.18308940236029914}, {"Real Matrix Element"=2.7034477958240903, "Real Matrix Element"=0.1584395348511924}, {"Real Matrix Element"=2.808962129568583, "Real Matrix Element"=0.19054470501938017}, {"Real Matrix Element"=2.7935811032145845, "Real Matrix Element"=0.19664656262588825}, {"Real Matrix Element"=2.8479635903117453, "Real Matrix Element"=0.2544079128250215}, {"Real Matrix Element"=2.9099581448524052, "Real Matrix Element"=0.26166317839041964}, {"Real Matrix Element"=2.9941008825727495, "Real Matrix Element"=0.37724731663750566}, {"Real Matrix Element"=3.0696322037673434, "Real Matrix Element"=0.43616587849537897}, {"Real Matrix Element"=3.313607933134788, "Real Matrix Element"=0.5377973732469223}, {"Real Matrix Element"=3.407363071618096, "Real Matrix Element"=0.5454551929218919}, {"Real Matrix Element"=3.5932194887442543, "Real Matrix Element"=0.6116917336731797}, {"Real Matrix Element"=3.3589035471419906, "Real Matrix Element"=0.4567263611684425}, {"Real Matrix Element"=3.695917876136339, "Real Matrix Element"=0.593581636176077}, {"Real Matrix Element"=3.6457952940222915, "Real Matrix Element"=0.5315292352998695}, {"Real Matrix Element"=3.714346392393845, "Real Matrix Element"=0.5702353304797363}, {"Real Matrix Element"=3.6786998407803813, "Real Matrix Element"=0.6054636907309058}, {"Real Matrix Element"=3.9695654037603383, "Real Matrix Element"=0.7474117378265733}, {"Real Matrix Element"=3.9679436409539326, "Real Matrix Element"=0.7798697252331893}, {"Real Matrix Element"=4.032111785642433, "Real Matrix Element"=0.7438287849427716}, {"Real Matrix Element"=4.283671298121345, "Real Matrix Element"=0.8534035037018595}, {"Real Matrix Element"=4.296721433827482, "Real Matrix Element"=0.8392037518838574}, {"Real Matrix Element"=4.322401435083846, "Real Matrix Element"=0.8249812619384859}, {"Real Matrix Element"=4.5191452140309005, "Real Matrix Element"=0.8878586861185592}, {"Real Matrix Element"=4.5224146622327694, "Real Matrix Element"=0.8969365889990356}, {"Real Matrix Element"=4.644799501912946, "Real Matrix Element"=0.9533337312647675}, {"Real Matrix Element"=4.646817795976238, "Real Matrix Element"=0.9846498532069283}, {"Real Matrix Element"=4.72864785546255, "Real Matrix Element"=1.072949743825018}, {"Real Matrix Element"=4.762008370616068, "Real Matrix Element"=1.1329781860610777}, {"Real Matrix Element"=4.998394591026046, "Real Matrix Element"=1.2913637380332101}, {"Real Matrix Element"=4.941107776346549, "Real Matrix Element"=1.3237196066420804}, {"Real Matrix Element"=5.079805162616702, "Real Matrix Element"=1.3657663460321086}, {"Real Matrix Element"=5.2009481940925175, "Real Matrix Element"=1.4374200056820017}, {"Real Matrix Element"=5.300671821256249, "Real Matrix Element"=1.4261486270785142}, {"Real Matrix Element"=5.518764473948176, "Real Matrix Element"=1.4738522666185208}, {"Real Matrix Element"=5.561120879860021, "Real Matrix Element"=1.5022260931653153}, {"Real Matrix Element"=5.718968926996007, "Real Matrix Element"=1.6260376778838932}, {"Real Matrix Element"=5.609518765708553, "Real Matrix Element"=1.5702823859466093}, {"Real Matrix Element"=5.551225978906439, "Real Matrix Element"=1.663120073974685}, {"Real Matrix Element"=5.67573163820368, "Real Matrix Element"=1.6472246274731763}, {"Real Matrix Element"=5.83000921298988, "Real Matrix Element"=1.7177836762039929}, {"Real Matrix Element"=5.849766426212605, "Real Matrix Element"=1.7565275361323225}, {"Real Matrix Element"=6.015671071456756, "Real Matrix Element"=1.9498133478662885}, {"Real Matrix Element"=6.032895177929508, "Real Matrix Element"=1.9169459000393234}, {"Real Matrix Element"=6.154929016590837, "Real Matrix Element"=2.056307800978188}, {"Real Matrix Element"=6.1463701752768385, "Real Matrix Element"=2.0709064667827093}, {"Real Matrix Element"=6.352949576997795, "Real Matrix Element"=2.1649496004112936}, {"Real Matrix Element"=6.427006560306094, "Real Matrix Element"=2.1905097881923696}, {"Real Matrix Element"=6.455077490021153, "Real Matrix Element"=2.3053947706988565}, {"Real Matrix Element"=6.479497981725081, "Real Matrix Element"=2.3252803019267163}, {"Real Matrix Element"=6.575404223684334, "Real Matrix Element"=2.4901798255409786}, {"Real Matrix Element"=6.595679953418508, "Real Matrix Element"=2.55728300359343}, {"Real Matrix Element"=6.538070571295576, "Real Matrix Element"=2.38340721057176}, {"Real Matrix Element"=6.759127818119429, "Real Matrix Element"=2.728247957954998}, {"Real Matrix Element"=6.770249748489607, "Real Matrix Element"=2.710803614297903}, {"Real Matrix Element"=6.865366575855089, "Real Matrix Element"=2.7959719527754574}, {"Real Matrix Element"=6.966912662090657, "Real Matrix Element"=2.9675313914087886}, {"Real Matrix Element"=7.067150751026892, "Real Matrix Element"=2.9959802631904227}, {"Real Matrix Element"=7.067292435701106, "Real Matrix Element"=2.951171632894142}, {"Real Matrix Element"=7.228725630431952, "Real Matrix Element"=3.11369972385143}, {"Real Matrix Element"=7.214345767950757, "Real Matrix Element"=3.054015089559799}, {"Real Matrix Element"=7.33540453015883, "Real Matrix Element"=3.2591032415120553}, {"Real Matrix Element"=7.330843211640194, "Real Matrix Element"=3.1755961232420145}, {"Real Matrix Element"=7.521946806251719, "Real Matrix Element"=3.4476966087214844}, {"Real Matrix Element"=7.621629826072786, "Real Matrix Element"=3.5495238724228213}, {"Real Matrix Element"=7.576292137032978, "Real Matrix Element"=3.465175674880314}, {"Real Matrix Element"=7.75996328147551, "Real Matrix Element"=3.676281254432389}, {"Real Matrix Element"=7.772080171849247, "Real Matrix Element"=3.662354087911986}, {"Real Matrix Element"=7.834000329010128, "Real Matrix Element"=3.7096879497402053}, {"Real Matrix Element"=8.034444348372084, "Real Matrix Element"=3.8840809597129993}, {"Real Matrix Element"=8.03627660926641, "Real Matrix Element"=3.8581867367868186}, {"Real Matrix Element"=8.051682657951124, "Real Matrix Element"=3.8834318364755642}, {"Real Matrix Element"=8.264548362052455, "Real Matrix Element"=4.076216604079336}, {"Real Matrix Element"=8.47945185253855, "Real Matrix Element"=4.329851817975151}, {"Real Matrix Element"=8.581974483173031, "Real Matrix Element"=4.425543104913617}, {"Real Matrix Element"=8.688143144500973, "Real Matrix Element"=4.529759583774541}, {"Real Matrix Element"=8.695326310305923, "Real Matrix Element"=4.530489334676922}, {"Real Matrix Element"=8.503010705517498, "Real Matrix Element"=4.356729286472276}, {"Real Matrix Element"=8.767311686143184, "Real Matrix Element"=4.597201027556191}, {"Real Matrix Element"=8.798879449785968, "Real Matrix Element"=4.7729663144035035}, {"Real Matrix Element"=8.821188654582679, "Real Matrix Element"=4.970616601426958}, {"Real Matrix Element"=8.59127844987887, "Real Matrix Element"=4.816925671534008}, {"Real Matrix Element"=8.67257110273227, "Real Matrix Element"=5.003563996599393}, {"Real Matrix Element"=8.703059828284593, "Real Matrix Element"=5.126710925947982}, {"Real Matrix Element"=8.741912578927936, "Real Matrix Element"=5.2078628320216405}, {"Real Matrix Element"=8.774671070361357, "Real Matrix Element"=5.275407890372337}, {"Real Matrix Element"=8.765146993325818, "Real Matrix Element"=5.268583018870127}, {"Real Matrix Element"=8.837485711714402, "Real Matrix Element"=5.4110451387601035}, {"Real Matrix Element"=8.959618180332722, "Real Matrix Element"=5.558737694889966}, {"Real Matrix Element"=8.88638163520557, "Real Matrix Element"=5.552457765502023}, {"Real Matrix Element"=9.022574776540285, "Real Matrix Element"=5.742407715488844}, {"Real Matrix Element"=9.032491085430822, "Real Matrix Element"=5.690315046104431}, {"Real Matrix Element"=9.044362899712723, "Real Matrix Element"=5.819343003060082}, {"Real Matrix Element"=9.055583893949986, "Real Matrix Element"=5.816210162409235}, {"Real Matrix Element"=9.066724425620222, "Real Matrix Element"=5.885495598796646}, {"Real Matrix Element"=9.12939138255846, "Real Matrix Element"=5.904572937385332}, {"Real Matrix Element"=9.364040991531096, "Real Matrix Element"=6.088487150459318}, {"Real Matrix Element"=9.43365851443683, "Real Matrix Element"=6.29608305424531}, {"Real Matrix Element"=9.304163971883792, "Real Matrix Element"=6.2765676897949625}, {"Real Matrix Element"=9.247951130808282, "Real Matrix Element"=6.542186264469406}, {"Real Matrix Element"=9.223223617551636, "Real Matrix Element"=6.477753607211691}]}, ...(3 in all)]
  in  "정지":bool
  in  "DT":dbl=2.0
  in  "SIM_TIME":dbl=100.0
  in  "MAX_RANGE":dbl=30.0
  in  "C_SIGMA1":dbl=0.1
  in  "STATE_SIZE":i32=3
  in  "R_sim deg":dbl=10.0 format="%#_13g"
  in  "R_sim range":dbl=0.1 format="%#_13g"
  in  "Q_sim range":dbl=0.2 format="%#_13g"
  in  "Q_sim deg":dbl=1.0 format="%#_13g"
  in  "C_SIGMA2":dbl=0.1
  in  "C_SIGMA3 deg":dbl=1.0 format="%.3f"
  in  "MAX_ITR":u32=20
  out "n":i32
  in  "Status detail":string="\r\n00:38:31.5 - System start \r\n"
  # "Graph Based SLAM"
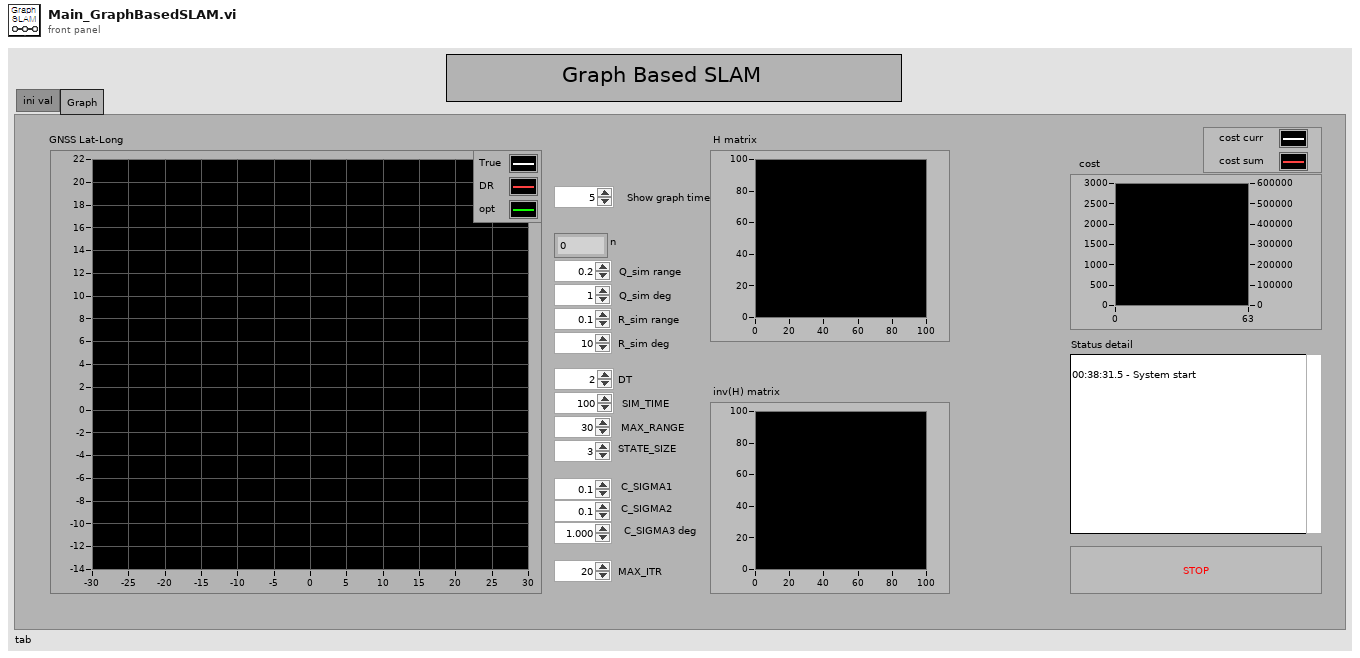
[diagram p1: front panel]
types:
  T1 = cluster{cluster{"Real Matrix Element":dbl, "Real Matrix Element":dbl}[]}[]
  T2 = typedef "cmd_ini-RW.ctl" = enum16{"ini", "read", "write"}
  T3 = typedef "cmd_common.ctl" = enum16{"read", "write"}
  T4 = typedef "NI_Matrix.lvlib/RealMatrix.ctl" = dbl[][]
  T5 = cluster{T4, T4, "DT":dbl, "SIM_TIME":dbl, "MAX_RANGE":dbl, "STATE_SIZE":i32, "C_SIGMA1":dbl, "C_SIGMA2":dbl, "rad":dbl, "MAX_ITR":u32}
  T6 = cluster{"rf_id":cluster{"x":dbl, "y":dbl, "yaw":dbl}[], "xTrue":T4, "xDR":T4}
  T7 = cluster{"Real Matrix Element":dbl, "Real Matrix Element":dbl, "Real Matrix Element":dbl}
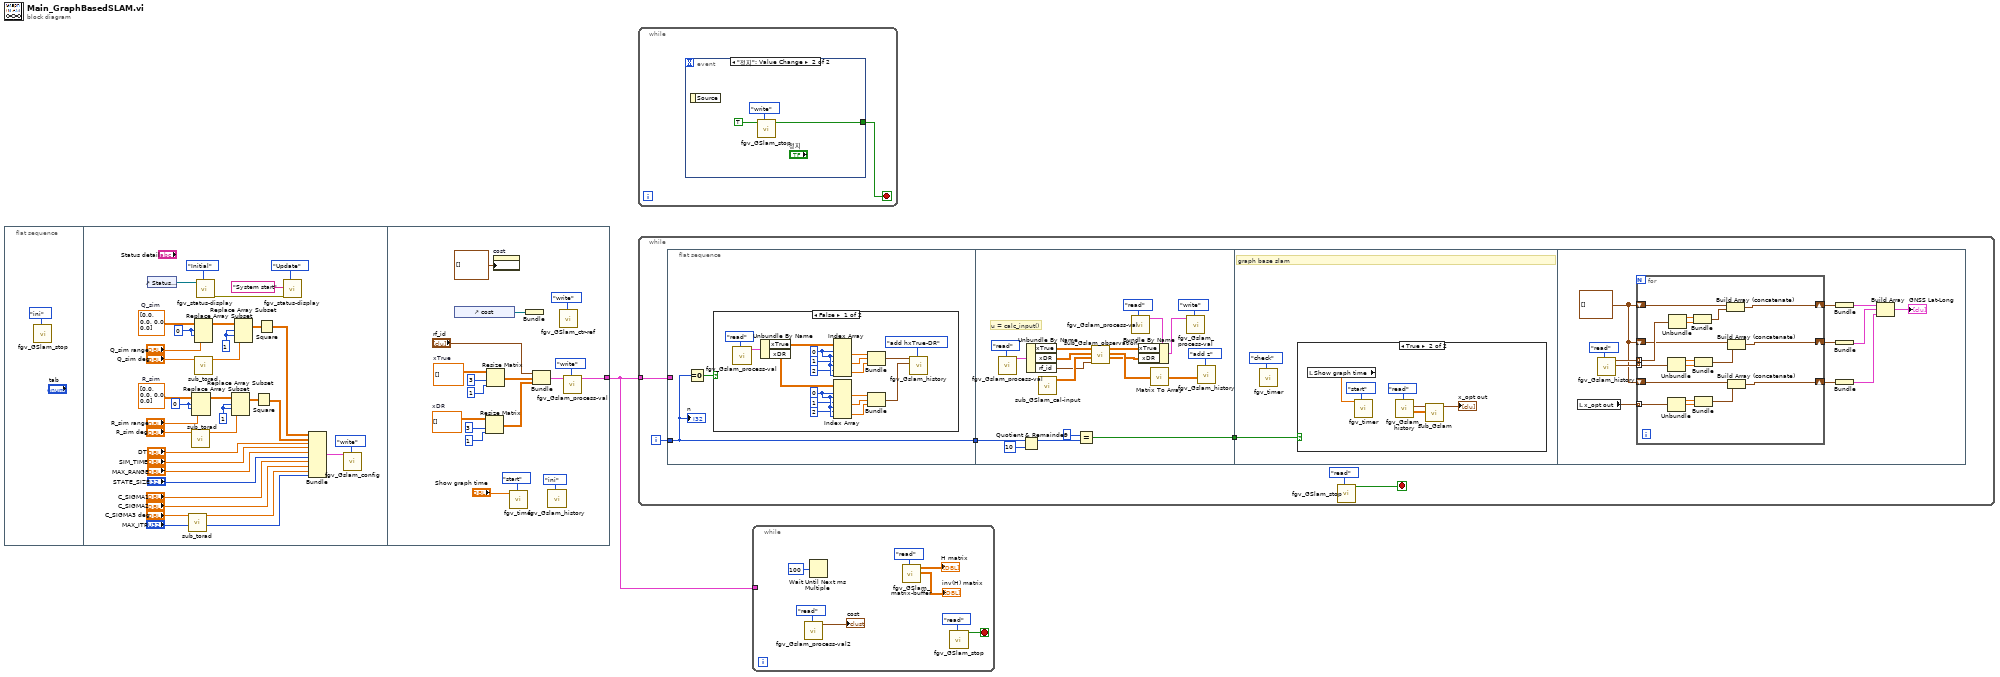
[diagram p0: block diagram]
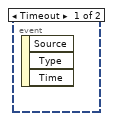
[diagram p2: hidden frame]
diagram:
  n1 = flat-sequence {
    tunnel: [w44] -> w1
    frame #0 {
      n2 = call "fgv_GSlam_stop.vi"("cmd"=cmd_ini-RW."ini") -> ()  [unwired: 10 in, 1 out]
    }
    frame #1 {
      w21 = dbl[][] [[0.0, 0.0], [0.0, 0.0]]  # Q_sim
      w22 = 0 ("인덱스 (행)")
      w20 = 1 ("비활성화된 인덱스 (행)")
      w24 = dbl[][] [[0.0, 0.0], [0.0, 0.0]]  # R_sim
      w23 = 0 ("인덱스 (행)")
      w26 = 1 ("비활성화된 인덱스 (행)")
      n3 = control-ref of="Status detail"() -> (w6:refnum<vi>)
      n4 = call "sub_torad.vi"("φ"="C_SIGMA3 deg") -> ("rad"=w8:dbl)  [unwired: 10 in]
      n5 = call "sub_torad.vi"("φ"="R_sim deg") -> ("rad"=w27:dbl)  [unwired: 10 in]
      n6 = Replace Array Subset(array=w24, new element="R_sim range", index (row)=w23, index (col)=w23) -> (w29:dbl[][])
      n7 = call "sub_torad.vi"("φ"="Q_sim deg") -> ("rad"=w19:dbl)  [unwired: 10 in]
      n8 = Replace Array Subset(array=w21, new element="Q_sim range", index (row)=w22, index (col)=w22) -> (w17:dbl[][])
      n9 = call "fgv_status-display.vi"("Mode"=enum16{"Initial", "Update", "Clear"}."Initial", "System Log"=w6) -> ("error out"=w7:errorcluster)  [unwired: 9 in]
      n10 = Replace Array Subset(array=w29, new element=w27, index (row)=w26, index (col)=w26) -> (w31:T4)
      n11 = Replace Array Subset(array=w17, new element=w19, index (row)=w20, index (col)=w20) -> (w15:T4)
      n12 = Square(x=w31) -> (x^2=w25:T4)
      n13 = Square(x=w15) -> (x^2=w14:T4)
      n14 = call "fgv_status-display.vi"("Mode"=enum16{"Initial", "Update", "Clear"}."Update", "error in"=w7, "title"="System start" ("String in 1")) -> ()  [unwired: 8 in, 1 out]
      n15 = Bundle(w14, w25, "DT"="DT", "SIM_TIME"="SIM_TIME", "MAX_RANGE"="MAX_RANGE", "STATE_SIZE"="STATE_SIZE", "C_SIGMA1"="C_SIGMA1", "C_SIGMA2"="C_SIGMA2", "rad"=w8, "MAX_ITR"="MAX_ITR") -> (w10:T5)  [unwired: 1 in]
      n16 = call "fgv_Gslam_config.vi"("cmd"=cmd_common."write", "G config"=w10) -> ()  [unwired: 9 in, 1 out]
    }
    frame #2 {
      w49 = T4 []  # xDR
      w52 = T4 []  # xTrue
      n17 = control-ref of="cost"() -> (w39:refnum<vi>)
      n18 = Resize Matrix(1:1 ("행의 개수"), 2:3 ("행의 개수"), 4:w49) -> (0:w45:T4)
      n19 = Resize Matrix(1:1 ("행의 개수"), 2:3 ("행의 개수"), 4:w52) -> (0:w46:T4)
      n20 = property on="cost" class="WFChart (strict)"("History Data"=cluster{"cost":dbl, "cost sum":dbl}[] [] ("히스토리 데이터")) -> ()  [unwired: 2 in, 2 out]
      n21 = call "fgv_timer.vi"("cmd"=enum16{"check", "start", "pause"}."start", "target time"="Show graph time") -> ()  [unwired: 7 in, 3 out]
      n22 = Bundle("cost"=w39) -> ()  [unwired: 1 in, 1 out]
      n23 = Bundle("rf_id"="rf_id", "xTrue"=w46, "xDR"=w45) -> (w43:T6)  [unwired: 1 in]
      n24 = call "fgv_Gslam_history.vi"("cmd"=enum16{"ini", "add hxTrue-DR", "add z", "read"}."ini") -> ()  [unwired: 8 in, 3 out]
      n25 = call "fgv_GSlam_ctr-ref.vi"("cmd"=cmd_common."write") -> ()  [unwired: 10 in, 1 out]
      n26 = call "fgv_Gslam_process-val.vi"("cmd"=cmd_common."write", "process val"=w43) -> ("process val out"=w44:T6)  [unwired: 9 in]
    }
  }
  n27 = while {
    stop <- w55 stop-if-true
    n28 = event shown="[1] \"정지\": Value Change" {
      selector: _ -> [_ _]
      dyn-events: _ -> [_ _]
      timeout: _ -> [_ _]
      tunnel: [_ w56] -> w55
      event Timeout {
        n29 = event-data() -> ()  [unwired: 1 in, 3 out]
      }
      event "정지": Value Change {
        n30 = event-data() -> ()  [unwired: 1 in, 1 out]
        n31 = call "fgv_GSlam_stop.vi"("cmd"=cmd_ini-RW."write", "val"=TRUE) -> ("val"=w56:bool)  [unwired: 9 in]
      }
    }
  }
  n32 = while {
    tunnel: w1 -> [w64]
    i -> [w61]
    stop <- w59 stop-if-true
    n33 = flat-sequence {
      tunnel: w61 -> [w65]
      tunnel: w64 -> [_]
      tunnel: [w65] -> w62
      tunnel: [w95] -> w63
      tunnel: w62 -> [w86]
      tunnel: w63 -> [w106]
      frame #0 {
        n34 = Equal To 0?(x=w65) -> (x = 0?=w66:bool)
        n35 = case shown="False" w66 {
          frame False {
            w76 = 0 ("index (row)")
            w73 = 0 ("index (row)")
            n36 = call "fgv_Gslam_process-val.vi"("cmd"=cmd_common."read") -> ("process val out"=w84:T6)  [unwired: 10 in]
            n37 = Unbundle By Name(w84) -> ("xTrue"=w70:T4, "xDR"=w69:T4)
            n38 = Index Array(array=w70, index (row) #1=w73, index (col) #1=w73, index (row) #2=1 ("index (row)"), index (col) #2=w73, index (row) #3=2 ("index (row)"), index (col) #3=w73) -> (element #1=w78:dbl, element #2=w77:dbl, element #3=w81:dbl)
            n39 = Index Array(array=w69, index (row) #1=w76, index (col) #1=w76, index (row) #2=1 ("index (row)"), index (col) #2=w76, index (row) #3=2 ("index (row)"), index (col) #3=w76) -> (element #1=w79:dbl, element #2=w80:dbl, element #3=w82:dbl)
            n40 = Bundle("Real Matrix Element"=w78, "Real Matrix Element"=w77, "Real Matrix Element"=w81) -> (w68:T7)  [unwired: 1 in]
            n41 = Bundle("Real Matrix Element"=w79, "Real Matrix Element"=w80, "Real Matrix Element"=w82) -> (w67:T7)  [unwired: 1 in]
            n42 = call "fgv_Gslam_history.vi"("cmd"=enum16{"ini", "add hxTrue-DR", "add z", "read"}."add hxTrue-DR", "x_dr"=w67, "x_true"=w68) -> ()  [unwired: 6 in, 3 out]
          }
          frame True {
          }
        }
        "n" <- w65
      }
      frame #1 {
        # "u = calc_input()"
        n43 = call "fgv_Gslam_process-val.vi"("cmd"=cmd_common."read") -> ("process val out"=w103:T6)  [unwired: 10 in]
        n44 = Quotient & Remainder(x=w86, y=10) -> (x-y*floor(x/y)=w94:i32)  [unwired: 1 out]
        n45 = Unbundle By Name(w103) -> ("xTrue"=w101:T4, "xDR"=w100:T4, "rf_id"=w102:cluster{"x":dbl, "y":dbl, "yaw":dbl}[])
        n46 = call "sub_GSlam_cal-input.vi"() -> ("u"=w105:T4)  [unwired: 11 in]
        n47 = Equal?(x=9, y=w94) -> (x = y?=w95:bool)
        n48 = call "sub_Gslam_observation.vi"("rf id"=w102, "u"=w105, "xd"=w100, "x_true"=w101) -> ("xd out"=w87:T4, "z"=w99:T4, "x_true out"=w88:T4)  [unwired: 4 in, 1 out]
        n49 = call "fgv_Gslam_process-val.vi"("cmd"=cmd_common."read") -> ("process val out"=w91:T6)  [unwired: 10 in]
        n50 = Bundle By Name(cluster=w91, "xTrue"=w88, "xDR"=w87) -> (w92:T6)
        n51 = call-poly <vilib>:"Matrix To Array.vi"("Real Matrix"=w99) -> ("Real 2D Array"=w98:dbl[][])
        n52 = call "fgv_Gslam_process-val.vi"("cmd"=cmd_common."write", "process val"=w92) -> ()  [unwired: 9 in, 1 out]
        n53 = call "fgv_Gslam_history.vi"("cmd"=enum16{"ini", "add hxTrue-DR", "add z", "read"}."add z", "z"=w98) -> ()  [unwired: 7 in, 3 out]
      }
      frame #2 {
        # "graph base slam"
        n54 = call "fgv_timer.vi"("cmd"=enum16{"check", "start", "pause"}."check") -> ()  [unwired: 8 in, 3 out]
        n55 = case shown="True" w106 {
          frame False {
          }
          frame True {
            n56 = local read "Show graph time"() -> (w112:dbl)
            n57 = call "fgv_timer.vi"("cmd"=enum16{"check", "start", "pause"}."start", "target time"=w112) -> ()  [unwired: 7 in, 3 out]
            n58 = call "fgv_Gslam_history.vi"("cmd"=enum16{"ini", "add hxTrue-DR", "add z", "read"}."read") -> ("hz"=w110:dbl[][][], "hxDR"=w111:cluster{"x":dbl, "y":dbl, "yaw":dbl}[])  [unwired: 8 in, 1 out]
            n59 = call "sub_Gslam.vi"("hz"=w110, "hxDR"=w111) -> ("x_opt out"=→"x_opt out":cluster{"x":dbl, "y":dbl, "yaw":dbl}[])  [unwired: 9 in]
          }
        }
      }
      frame #3 {
        w116 = cluster{"x":dbl, "y":dbl}[] []
        n60 = local read "x_opt out"() -> (w115:cluster{"x":dbl, "y":dbl, "yaw":dbl}[])
        n61 = call "fgv_Gslam_history.vi"("cmd"=enum16{"ini", "add hxTrue-DR", "add z", "read"}."read") -> ("hxDR"=w123:cluster{"x":dbl, "y":dbl, "yaw":dbl}[], "hxTrue"=w124:cluster{"x":dbl, "y":dbl, "yaw":dbl}[])  [unwired: 8 in, 1 out]
        n62 = for {
          tunnel: w124 -> [w143] mode=indexing
          tunnel: w123 -> [w135] mode=indexing
          shift-right: [w138] -> w122
          shift-left: w116 -> [w139]
          shift-right: [w133] -> w121
          shift-left: w116 -> [w134]
          tunnel: w115 -> [w128] mode=indexing
          shift-right: [w130] -> w117
          shift-left: w116 -> [w129]
          n63 = Unbundle(w135) -> ("x"=w136:dbl, "y"=w137:dbl)  [unwired: 1 out]
          n64 = Unbundle(w128) -> ("x"=w127:dbl, "y"=w126:dbl)  [unwired: 1 out]
          n65 = Unbundle(w143) -> ("x"=w142:dbl, "y"=w141:dbl)  [unwired: 1 out]
          n66 = Bundle("x"=w142, "y"=w141) -> (w140:cluster{"x":dbl, "y":dbl})  [unwired: 1 in]
          n67 = Bundle("x"=w136, "y"=w137) -> (w132:cluster{"x":dbl, "y":dbl})  [unwired: 1 in]
          n68 = Bundle("x"=w127, "y"=w126) -> (w131:cluster{"x":dbl, "y":dbl})  [unwired: 1 in]
          n69 = Build Array (concatenate)(w139, w140) -> (w138:cluster{"x":dbl, "y":dbl}[])
          n70 = Build Array (concatenate)(w134, w132) -> (w133:cluster{"x":dbl, "y":dbl}[])
          n71 = Build Array (concatenate)(w129, w131) -> (w130:cluster{"x":dbl, "y":dbl}[])
        }
        n72 = Bundle(w122) -> (w120:cluster{cluster{"x":dbl, "y":dbl}[]})  [unwired: 1 in]
        n73 = Bundle(w121) -> (w119:cluster{cluster{"x":dbl, "y":dbl}[]})  [unwired: 1 in]
        n74 = Bundle(w117) -> (w114:cluster{cluster{"x":dbl, "y":dbl}[]})  [unwired: 1 in]
        n75 = Build Array(w120, w119, w114) -> (→"GNSS Lat-Long":cluster{cluster{"x":dbl, "y":dbl}[]}[])
      }
    }
    n76 = call "fgv_GSlam_stop.vi"("cmd"=cmd_ini-RW."read") -> ("val"=w59:bool)  [unwired: 10 in]
  }
  n77 = while {
    tunnel: w1 -> [_]
    stop <- w144 stop-if-true
    n78 = call "fgv_Gslam_process-val2.vi"("cmd"=cmd_common."read") -> ("data 2"=→"cost":cluster{"cost":dbl, "cost sum":dbl})  [unwired: 10 in]
    n79 = Wait Until Next ms Multiple(millisecond multiple=u32 100 ("대기 시간 (ms)")) -> ()  [unwired: 1 out]
    n80 = call "fgv_GSlam_matrix-buffer.vi"("cmd"=enum16{"write H", "write inv(H)", "read"}."read") -> ("H inv out"=→"inv(H) matrix":T4, "H out"=→"H matrix":T4)  [unwired: 9 in]
    n81 = call "fgv_GSlam_stop.vi"("cmd"=cmd_ini-RW."read") -> ("val"=w144:bool)  [unwired: 10 in]
  }
